vi "Striptest.vi"(1 "Simulation?":bool) -> ()   [LabVIEW 2019]
uses:
  InstrControl/LCRControl/LCRControl.lvclass
  C:/Users/Graham Greig/Desktop/itk-strip-sensor-qc/LabVIEW 2019/InstrControl/InstrControl.lvclass
  general_VIs/globals/QC_MeasurementSetup.vi
  striptest/ProbePlan/ProbePlanParams.vi
  general_VIs/globals/QC_RunInformation.vi
  InstrControl/InstrumentSetup.vi
  <vilib>/regexp/Match Regular Expression.xnode
  InstrControl/SupplyControl/SupplyControl.lvclass
  InstrControl/Switching/Switching.lvclass
  InstrControl/ProbeStationControl/ProbeStationControl.lvclass
  InstrControl/InstrControl.lvclass
  InstrControl/ArduinoControl/ArduinoControl.lvclass
  <vilib>/Analysis/NI_AALBase.lvlib
panel:
  out "Tab Control":enum32{"Striptest Setup", "Striptest"}(tab)
  in  "Switching":string(combo)="LXIPXI Switching"
  in  "Bias Voltage [V]":dbl=-150.0 format="%.1f"
  in  "Frequency [Hz] Setup":i32=1000 caption="Frequency [Hz]" format="%#.3p"
  in  "Minimum fraction\nof good strips":dbl=98.0 format="%.1g"
  in  "Quit":bool
  in  "Continue":bool
  in  "Measurement Configurations":bool
  in  "Pinholes Y/N":bool=TRUE
  in  "Capacitance Y/N":bool=TRUE
  in  "Resistance Y/N":bool=TRUE
  in  "Striptest SMU":string(combo)="Keithley 2657A"
  in  "LCR Meter":string(combo)="WayneKerr 6440B"
  in  "Temperature":enum16{"Read Arduino", "Enter manually"}(ring)
  in  "Bias Supply":string(combo)="Keithley 2410"
  in  "Hardware Configurations":bool
  in  "DB Serial No. IN:":string caption="DB Serial No.:"
  in  "User:":string(combo)="Graham"
  in  "Batch No. IN:":string caption="Batch No.:"
  in  "Device Category IN:":string(combo)="ATLAS12EC" caption="Device Category:"
  in  "Sensor Serial No. IN:":string caption="Sensor Serial No.:"
  in  "From4":u16(ring) items=["Strip 0", "Strip 1", "Strip 2", "Strip 3", "Strip 4", "Strip 5", "Strip 6", "Strip 7", "Strip 8", "Strip 9", "Strip 10", "Strip 11", "Strip 12", "Strip 13", "Strip 14", "Strip 15", "Strip 16", "Strip 17", "Strip 18", "Strip 19", "Strip 20", "Strip 21", "Strip 22", "Strip 23", "Strip 24", "Strip 25", "Strip 26", "Strip 27", "Strip 28", "Strip 29", "Strip 30", "Strip 31", "Strip 32", "Strip 33", "Strip 34", "Strip 35", "Strip 36", "Strip 37", "Strip 38", "Strip 39", "Strip 40", "Strip 41", "Strip 42", "Strip 43", "Strip 44", "Strip 45", "Strip 46", "Strip 47", "Strip 48", "Strip 49", "Strip 50", "Strip 51", "Strip 52", "Strip 53", "Strip 54", "Strip 55", "Strip 56", "Strip 57", "Strip 58", "Strip 59", "Strip 60", "Strip 61", "Strip 62", "Strip 63", "Strip 64", "Strip 65", "Strip 66", "Strip 67", "Strip 68", "Strip 69", "Strip 70", "Strip 71", "Strip 72", "Strip 73", "Strip 74", "Strip 75", "Strip 76", "Strip 77", "Strip 78", "Strip 79", "Strip 80", "Strip 81", "Strip 82", "Strip 83", "Strip 84", "Strip 85", "Strip 86", "Strip 87", "Strip 88", "Strip 89", "Strip 90", "Strip 91", "Strip 92", "Strip 93", "Strip 94", "Strip 95", "Strip 96", "Strip 97", "Strip 98", "Strip 99", "Strip 100", "Strip 101", "Strip 102", "Strip 103", "Strip 104", "Strip 105", "Strip 106", "Strip 107", "Strip 108", "Strip 109", "Strip 110", "Strip 111", "Strip 112", "Strip 113", "Strip 114", "Strip 115", "Strip 116", "Strip 117", "Strip 118", "Strip 119", "Strip 120", "Strip 121", "Strip 122", "Strip 123", "Strip 124", "Strip 125", "Strip 126", "Strip 127", "Strip 128", "Strip 129", "Strip 130", "Strip 131", "Strip 132", "Strip 133", "Strip 134", "Strip 135", "Strip 136", "Strip 137", "Strip 138", "Strip 139", "Strip 140", "Strip 141", "Strip 142", "Strip 143", "Strip 144", "Strip 145", "Strip 146", "Strip 147", "Strip 148", "Strip 149", "Strip 150", "Strip 151", "Strip 152", "Strip 153", "Strip 154", "Strip 155", "Strip 156", "Strip 157", "Strip 158", "Strip 159", "Strip 160", "Strip 161", "Strip 162", "Strip 163", "Strip 164", "Strip 165", "Strip 166", "Strip 167", "Strip 168", "Strip 169", "Strip 170", "Strip 171", "Strip 172", "Strip 173", "Strip 174", "Strip 175", "Strip 176", "Strip 177", "Strip 178", "Strip 179", "Strip 180", "Strip 181", "Strip 182", "Strip 183", "Strip 184", "Strip 185", "Strip 186", "Strip 187", "Strip 188", "Strip 189", "Strip 190", "Strip 191", "Strip 192", "Strip 193", "Strip 194", "Strip 195", "Strip 196", "Strip 197", "Strip 198", "Strip 199", "Strip 200", "Strip 201", "Strip 202", "Strip 203", "Strip 204", "Strip 205", "Strip 206", "Strip 207", "Strip 208", "Strip 209", "Strip 210", "Strip 211", "Strip 212", "Strip 213", "Strip 214", "Strip 215", "Strip 216", "Strip 217", "Strip 218", "Strip 219", "Strip 220", "Strip 221", "Strip 222", "Strip 223", "Strip 224", "Strip 225", "Strip 226", "Strip 227", "Strip 228", "Strip 229", "Strip 230", "Strip 231", "Strip 232", "Strip 233", "Strip 234", "Strip 235", "Strip 236", "Strip 237", "Strip 238", "Strip 239", "Strip 240", "Strip 241", "Strip 242", "Strip 243", "Strip 244", "Strip 245", "Strip 246", "Strip 247", "Strip 248", "Strip 249", "Strip 250", "Strip 251", "Strip 252", "Strip 253", "Strip 254", "Strip 255", "Strip 256", "Strip 257", "Strip 258", "Strip 259", "Strip 260", "Strip 261", "Strip 262", "Strip 263", "Strip 264", "Strip 265", "Strip 266", "Strip 267", "Strip 268", "Strip 269", "Strip 270", "Strip 271", "Strip 272", "Strip 273", "Strip 274", "Strip 275", "Strip 276", "Strip 277", "Strip 278", "Strip 279", "Strip 280", "Strip 281", "Strip 282", "Strip 283", "Strip 284", "Strip 285", "Strip 286", "Strip 287", "Strip 288", "Strip 289", "Strip 290", "Strip 291", "Strip 292", "Strip 293", "Strip 294", "Strip 295", "Strip 296", "Strip 297", "Strip 298", "Strip 299", "Strip 300", "Strip 301", "Strip 302", "Strip 303", "Strip 304", "Strip 305", "Strip 306", "Strip 307", "Strip 308", "Strip 309", "Strip 310", "Strip 311", "Strip 312", "Strip 313", "Strip 314", "Strip 315", "Strip 316", "Strip 317", "Strip 318", "Strip 319", "Strip 320", "Strip 321", "Strip 322", "Strip 323", "Strip 324", "Strip 325", "Strip 326", "Strip 327", "Strip 328", "Strip 329", "Strip 330", "Strip 331", "Strip 332", "Strip 333", "Strip 334", "Strip 335", "Strip 336", "Strip 337", "Strip 338", "Strip 339", "Strip 340", "Strip 341", "Strip 342", "Strip 343", "Strip 344", "Strip 345", "Strip 346", "Strip 347", "Strip 348", "Strip 349", "Strip 350", "Strip 351", "Strip 352", "Strip 353", "Strip 354", "Strip 355", "Strip 356", "Strip 357", "Strip 358", "Strip 359", "Strip 360", "Strip 361", "Strip 362", "Strip 363", "Strip 364", "Strip 365", "Strip 366", "Strip 367", "Strip 368", "Strip 369", "Strip 370", "Strip 371", "Strip 372", "Strip 373", "Strip 374", "Strip 375", "Strip 376", "Strip 377", "Strip 378", "Strip 379", "Strip 380", "Strip 381", "Strip 382", "Strip 383", "Strip 384", "Strip 385", "Strip 386", "Strip 387", "Strip 388", "Strip 389", "Strip 390", "Strip 391", "Strip 392", "Strip 393", "Strip 394", "Strip 395", "Strip 396", "Strip 397", "Strip 398", "Strip 399", "Strip 400", "Strip 401", "Strip 402", "Strip 403", "Strip 404", "Strip 405", "Strip 406", "Strip 407", "Strip 408", "Strip 409", "Strip 410", "Strip 411", "Strip 412", "Strip 413", "Strip 414", "Strip 415", "Strip 416", "Strip 417", "Strip 418", "Strip 419", "Strip 420", "Strip 421", "Strip 422", "Strip 423", "Strip 424", "Strip 425", "Strip 426", "Strip 427", "Strip 428", "Strip 429", "Strip 430", "Strip 431", "Strip 432", "Strip 433", "Strip 434", "Strip 435", "Strip 436", "Strip 437", "Strip 438", "Strip 439", "Strip 440", "Strip 441", "Strip 442", "Strip 443", "Strip 444", "Strip 445", "Strip 446", "Strip 447", "Strip 448", "Strip 449", "Strip 450", "Strip 451", "Strip 452", "Strip 453", "Strip 454", "Strip 455", "Strip 456", "Strip 457", "Strip 458", "Strip 459", "Strip 460", "Strip 461", "Strip 462", "Strip 463", "Strip 464", "Strip 465", "Strip 466", "Strip 467", "Strip 468", "Strip 469", "Strip 470", "Strip 471", "Strip 472", "Strip 473", "Strip 474", "Strip 475", "Strip 476", "Strip 477", "Strip 478", "Strip 479", "Strip 480", "Strip 481", "Strip 482", "Strip 483", "Strip 484", "Strip 485", "Strip 486", "Strip 487", "Strip 488", "Strip 489", "Strip 490", "Strip 491", "Strip 492", "Strip 493", "Strip 494", "Strip 495", "Strip 496", "Strip 497", "Strip 498", "Strip 499", "Strip 500", "Strip 501", "Strip 502", "Strip 503", "Strip 504", "Strip 505", "Strip 506", "Strip 507", "Strip 508", "Strip 509", "Strip 510", "Strip 511", "Strip 512", "Strip 513", "Strip 514", "Strip 515", "Strip 516", "Strip 517", "Strip 518", "Strip 519", "Strip 520", "Strip 521", "Strip 522", "Strip 523", "Strip 524", "Strip 525", "Strip 526", "Strip 527", "Strip 528", "Strip 529", "Strip 530", "Strip 531", "Strip 532", "Strip 533", "Strip 534", "Strip 535", "Strip 536", "Strip 537", "Strip 538", "Strip 539", "Strip 540", "Strip 541", "Strip 542", "Strip 543", "Strip 544", "Strip 545", "Strip 546", "Strip 547", "Strip 548", "Strip 549", "Strip 550", "Strip 551", "Strip 552", "Strip 553", "Strip 554", "Strip 555", "Strip 556", "Strip 557", "Strip 558", "Strip 559", "Strip 560", "Strip 561", "Strip 562", "Strip 563", "Strip 564", "Strip 565", "Strip 566", "Strip 567", "Strip 568", "Strip 569", "Strip 570", "Strip 571", "Strip 572", "Strip 573", "Strip 574", "Strip 575", "Strip 576", "Strip 577", "Strip 578", "Strip 579", "Strip 580", "Strip 581", "Strip 582", "Strip 583", "Strip 584", "Strip 585", "Strip 586", "Strip 587", "Strip 588", "Strip 589", "Strip 590", "Strip 591", "Strip 592", "Strip 593", "Strip 594", "Strip 595", "Strip 596", "Strip 597", "Strip 598", "Strip 599", "Strip 600", "Strip 601", "Strip 602", "Strip 603", "Strip 604", "Strip 605", "Strip 606", "Strip 607", "Strip 608", "Strip 609", "Strip 610", "Strip 611", "Strip 612", "Strip 613", "Strip 614", "Strip 615", "Strip 616", "Strip 617", "Strip 618", "Strip 619", "Strip 620", "Strip 621", "Strip 622", "Strip 623", "Strip 624", "Strip 625", "Strip 626", "Strip 627", "Strip 628", "Strip 629", "Strip 630", "Strip 631", "Strip 632", "Strip 633", "Strip 634", "Strip 635", "Strip 636", "Strip 637", "Strip 638", "Strip 639", "Strip 640", "Strip 641", "Strip 642", "Strip 643", "Strip 644", "Strip 645", "Strip 646", "Strip 647", "Strip 648", "Strip 649", "Strip 650", "Strip 651", "Strip 652", "Strip 653", "Strip 654", "Strip 655", "Strip 656", "Strip 657", "Strip 658", "Strip 659", "Strip 660", "Strip 661", "Strip 662", "Strip 663", "Strip 664", "Strip 665", "Strip 666", "Strip 667", "Strip 668", "Strip 669", "Strip 670", "Strip 671", "Strip 672", "Strip 673", "Strip 674", "Strip 675", "Strip 676", "Strip 677", "Strip 678", "Strip 679", "Strip 680", "Strip 681", "Strip 682", "Strip 683", "Strip 684", "Strip 685", "Strip 686", "Strip 687", "Strip 688", "Strip 689", "Strip 690", "Strip 691", "Strip 692", "Strip 693", "Strip 694", "Strip 695", "Strip 696", "Strip 697", "Strip 698", "Strip 699", "Strip 700", "Strip 701", "Strip 702", "Strip 703", "Strip 704", "Strip 705", "Strip 706", "Strip 707", "Strip 708", "Strip 709", "Strip 710", "Strip 711", "Strip 712", "Strip 713", "Strip 714", "Strip 715", "Strip 716", "Strip 717", "Strip 718", "Strip 719", "Strip 720", "Strip 721", "Strip 722", "Strip 723", "Strip 724", "Strip 725", "Strip 726", "Strip 727", "Strip 728", "Strip 729", "Strip 730", "Strip 731", "Strip 732", "Strip 733", "Strip 734", "Strip 735", "Strip 736", "Strip 737", "Strip 738", "Strip 739", "Strip 740", "Strip 741", "Strip 742", "Strip 743", "Strip 744", "Strip 745", "Strip 746", "Strip 747", "Strip 748", "Strip 749", "Strip 750", "Strip 751", "Strip 752", "Strip 753", "Strip 754", "Strip 755", "Strip 756", "Strip 757", "Strip 758", "Strip 759", "Strip 760", "Strip 761", "Strip 762", "Strip 763", "Strip 764", "Strip 765", "Strip 766", "Strip 767", "Strip 768", "Strip 769", "Strip 770", "Strip 771", "Strip 772", "Strip 773", "Strip 774", "Strip 775", "Strip 776", "Strip 777", "Strip 778", "Strip 779", "Strip 780", "Strip 781", "Strip 782", "Strip 783", "Strip 784", "Strip 785", "Strip 786", "Strip 787", "Strip 788", "Strip 789", "Strip 790", "Strip 791", "Strip 792", "Strip 793", "Strip 794", "Strip 795", "Strip 796", "Strip 797", "Strip 798", "Strip 799", "Strip 800", "Strip 801", "Strip 802", "Strip 803", "Strip 804", "Strip 805", "Strip 806", "Strip 807", "Strip 808", "Strip 809", "Strip 810", "Strip 811", "Strip 812", "Strip 813", "Strip 814", "Strip 815", "Strip 816", "Strip 817", "Strip 818", "Strip 819", "Strip 820", "Strip 821", "Strip 822", "Strip 823", "Strip 824", "Strip 825", "Strip 826", "Strip 827", "Strip 828", "Strip 829", "Strip 830", "Strip 831", "Strip 832", "Strip 833", "Strip 834", "Strip 835", "Strip 836", "Strip 837", "Strip 838", "Strip 839", "Strip 840", "Strip 841", "Strip 842", "Strip 843", "Strip 844", "Strip 845", "Strip 846", "Strip 847", "Strip 848", "Strip 849", "Strip 850", "Strip 851", "Strip 852", "Strip 853", "Strip 854", "Strip 855", "Strip 856", "Strip 857", "Strip 858", "Strip 859", "Strip 860", "Strip 861", "Strip 862", "Strip 863", "Strip 864", "Strip 865", "Strip 866", "Strip 867", "Strip 868", "Strip 869", "Strip 870", "Strip 871", "Strip 872", "Strip 873", "Strip 874", "Strip 875", "Strip 876", "Strip 877", "Strip 878", "Strip 879", "Strip 880", "Strip 881", "Strip 882", "Strip 883", "Strip 884", "Strip 885", "Strip 886", "Strip 887", "Strip 888", "Strip 889", "Strip 890", "Strip 891", "Strip 892", "Strip 893", "Strip 894", "Strip 895", "Strip 896", "Strip 897", "Strip 898", "Strip 899", "Strip 900", "Strip 901", "Strip 902", "Strip 903", "Strip 904", "Strip 905", "Strip 906", "Strip 907", "Strip 908", "Strip 909", "Strip 910", "Strip 911", "Strip 912", "Strip 913", "Strip 914", "Strip 915", "Strip 916", "Strip 917", "Strip 918", "Strip 919", "Strip 920", "Strip 921", "Strip 922", "Strip 923", "Strip 924", "Strip 925", "Strip 926", "Strip 927", "Strip 928", "Strip 929", "Strip 930", "Strip 931", "Strip 932", "Strip 933", "Strip 934", "Strip 935", "Strip 936", "Strip 937", "Strip 938", "Strip 939", "Strip 940", "Strip 941", "Strip 942", "Strip 943", "Strip 944", "Strip 945", "Strip 946", "Strip 947", "Strip 948", "Strip 949", "Strip 950", "Strip 951", "Strip 952", "Strip 953", "Strip 954", "Strip 955", "Strip 956", "Strip 957", "Strip 958", "Strip 959", "Strip 960", "Strip 961", "Strip 962", "Strip 963", "Strip 964", "Strip 965", "Strip 966", "Strip 967", "Strip 968", "Strip 969", "Strip 970", "Strip 971", "Strip 972", "Strip 973", "Strip 974", "Strip 975", "Strip 976", "Strip 977", "Strip 978", "Strip 979", "Strip 980", "Strip 981", "Strip 982", "Strip 983", "Strip 984", "Strip 985", "Strip 986", "Strip 987", "Strip 988", "Strip 989", "Strip 990", "Strip 991", "Strip 992", "Strip 993", "Strip 994", "Strip 995", "Strip 996", "Strip 997", "Strip 998", "Strip 999", "Strip 1000", "Strip 1001", "Strip 1002", "Strip 1003", "Strip 1004", "Strip 1005", "Strip 1006", "Strip 1007", "Strip 1008", "Strip 1009", "Strip 1010", "Strip 1011", "Strip 1012", "Strip 1013", "Strip 1014", "Strip 1015", "Strip 1016", "Strip 1017", "Strip 1018", "Strip 1019", "Strip 1020", "Strip 1021", "Strip 1022", "Strip 1023", "Strip 1024", "Strip 1025", "Strip 1026", "Strip 1027", "Strip 1028", "Strip 1029", "Strip 1030", "Strip 1031", "Strip 1032", "Strip 1033", "Strip 1034", "Strip 1035", "Strip 1036", "Strip 1037", "Strip 1038", "Strip 1039", "Strip 1040", "Strip 1041", "Strip 1042", "Strip 1043", "Strip 1044", "Strip 1045", "Strip 1046", "Strip 1047", "Strip 1048", "Strip 1049", "Strip 1050", "Strip 1051", "Strip 1052", "Strip 1053", "Strip 1054", "Strip 1055", "Strip 1056", "Strip 1057", "Strip 1058", "Strip 1059", "Strip 1060", "Strip 1061", "Strip 1062", "Strip 1063", "Strip 1064", "Strip 1065", "Strip 1066", "Strip 1067", "Strip 1068", "Strip 1069", "Strip 1070", "Strip 1071", "Strip 1072", "Strip 1073", "Strip 1074", "Strip 1075", "Strip 1076", "Strip 1077", "Strip 1078", "Strip 1079", "Strip 1080", "Strip 1081", "Strip 1082", "Strip 1083", "Strip 1084", "Strip 1085", "Strip 1086", "Strip 1087", "Strip 1088", "Strip 1089", "Strip 1090", "Strip 1091", "Strip 1092", "Strip 1093", "Strip 1094", "Strip 1095", "Strip 1096", "Strip 1097", "Strip 1098", "Strip 1099", "Strip 1100", "Strip 1101", "Strip 1102", "Strip 1103", "Strip 1104", "Strip 1105", "Strip 1106", "Strip 1107", "Strip 1108", "Strip 1109", "Strip 1110", "Strip 1111", "Strip 1112", "Strip 1113", "Strip 1114", "Strip 1115", "Strip 1116", "Strip 1117", "Strip 1118", "Strip 1119", "Strip 1120", "Strip 1121", "Strip 1122", "Strip 1123", "Strip 1124", "Strip 1125", "Strip 1126", "Strip 1127", "Strip 1128", "Strip 1129", "Strip 1130", "Strip 1131", "Strip 1132", "Strip 1133", "Strip 1134", "Strip 1135", "Strip 1136", "Strip 1137", "Strip 1138", "Strip 1139", "Strip 1140", "Strip 1141", "Strip 1142", "Strip 1143", "Strip 1144", "Strip 1145", "Strip 1146", "Strip 1147", "Strip 1148", "Strip 1149", "Strip 1150", "Strip 1151", "Strip 1152", "Strip 1153", "Strip 1154", "Strip 1155", "Strip 1156", "Strip 1157", "Strip 1158", "Strip 1159", "Strip 1160", "Strip 1161", "Strip 1162", "Strip 1163", "Strip 1164", "Strip 1165", "Strip 1166", "Strip 1167", "Strip 1168", "Strip 1169", "Strip 1170", "Strip 1171", "Strip 1172", "Strip 1173", "Strip 1174", "Strip 1175", "Strip 1176", "Strip 1177", "Strip 1178", "Strip 1179", "Strip 1180", "Strip 1181", "Strip 1182", "Strip 1183", "Strip 1184", "Strip 1185", "Strip 1186", "Strip 1187", "Strip 1188", "Strip 1189", "Strip 1190", "Strip 1191", "Strip 1192", "Strip 1193", "Strip 1194", "Strip 1195", "Strip 1196", "Strip 1197", "Strip 1198", "Strip 1199", "Strip 1200", "Strip 1201", "Strip 1202", "Strip 1203", "Strip 1204", "Strip 1205", "Strip 1206", "Strip 1207", "Strip 1208", "Strip 1209", "Strip 1210", "Strip 1211", "Strip 1212", "Strip 1213", "Strip 1214", "Strip 1215", "Strip 1216", "Strip 1217", "Strip 1218", "Strip 1219", "Strip 1220", "Strip 1221", "Strip 1222", "Strip 1223", "Strip 1224", "Strip 1225", "Strip 1226", "Strip 1227", "Strip 1228", "Strip 1229", "Strip 1230", "Strip 1231", "Strip 1232", "Strip 1233", "Strip 1234", "Strip 1235", "Strip 1236", "Strip 1237", "Strip 1238", "Strip 1239", "Strip 1240", "Strip 1241", "Strip 1242", "Strip 1243", "Strip 1244", "Strip 1245", "Strip 1246", "Strip 1247", "Strip 1248", "Strip 1249", "Strip 1250", "Strip 1251", "Strip 1252", "Strip 1253", "Strip 1254", "Strip 1255", "Strip 1256", "Strip 1257", "Strip 1258", "Strip 1259", "Strip 1260", "Strip 1261", "Strip 1262", "Strip 1263", "Strip 1264", "Strip 1265", "Strip 1266", "Strip 1267", "Strip 1268", "Strip 1269", "Strip 1270", "Strip 1271", "Strip 1272", "Strip 1273", "Strip 1274", "Strip 1275", "Strip 1276", "Strip 1277", "Strip 1278", "Strip 1279", "Strip 1280", "Strip 1281", "Strip 1282", "Strip 1283", "Strip 1284", "Strip 1285", "Strip 1286", "Strip 1287", "Strip 1288", "Strip 1289", "Strip 1290", "Strip 1291", "Strip 1292", "Strip 1293", "Strip 1294", "Strip 1295", "Strip 1296", "Strip 1297", "Strip 1298", "Strip 1299", "Strip 1300", "Strip 1301", "Strip 1302", "Strip 1303", "Strip 1304", "Strip 1305", "Strip 1306", "Strip 1307", "Strip 1308", "Strip 1309", "Strip 1310", "Strip 1311", "Strip 1312", "Strip 1313", "Strip 1314", "Strip 1315", "Strip 1316", "Strip 1317", "Strip 1318", "Strip 1319", "Strip 1320", "Strip 1321", "Strip 1322", "Strip 1323", "Strip 1324", "Strip 1325", "Strip 1326", "Strip 1327", "Strip 1328", "Strip 1329", "Strip 1330", "Strip 1331", "Strip 1332", "Strip 1333", "Strip 1334", "Strip 1335", "Strip 1336", "Strip 1337", "Strip 1338", "Strip 1339", "Strip 1340", "Strip 1341", "Strip 1342", "Strip 1343", "Strip 1344", "Strip 1345", "Strip 1346", "Strip 1347", "Strip 1348", "Strip 1349", "Strip 1350", "Strip 1351", "Strip 1352", "Strip 1353", "Strip 1354", "Strip 1355", "Strip 1356", "Strip 1357", "Strip 1358", "Strip 1359", "Strip 1360", "Strip 1361", "Strip 1362", "Strip 1363", "Strip 1364", "Strip 1365", "Strip 1366", "Strip 1367", "Strip 1368", "Strip 1369", "Strip 1370", "Strip 1371", "Strip 1372", "Strip 1373", "Strip 1374", "Strip 1375", "Strip 1376", "Strip 1377", "Strip 1378", "Strip 1379", "Strip 1380", "Strip 1381", "Strip 1382", "Strip 1383", "Strip 1384", "Strip 1385", "Strip 1386", "Strip 1387", "Strip 1388", "Strip 1389", "Strip 1390", "Strip 1391", "Strip 1392", "Strip 1393", "Strip 1394", "Strip 1395", "Strip 1396", "Strip 1397", "Strip 1398", "Strip 1399", "Strip 1400", "Strip 1401", "Strip 1402", "Strip 1403", "Strip 1404", "Strip 1405", "Strip 1406", "Strip 1407", "Strip 1408", "Strip 1409"]
  in  "From3":u16(ring) items=["Strip 0", "Strip 1", "Strip 2", "Strip 3", "Strip 4", "Strip 5", "Strip 6", "Strip 7", "Strip 8", "Strip 9", "Strip 10", "Strip 11", "Strip 12", "Strip 13", "Strip 14", "Strip 15", "Strip 16", "Strip 17", "Strip 18", "Strip 19", "Strip 20", "Strip 21", "Strip 22", "Strip 23", "Strip 24", "Strip 25", "Strip 26", "Strip 27", "Strip 28", "Strip 29", "Strip 30", "Strip 31", "Strip 32", "Strip 33", "Strip 34", "Strip 35", "Strip 36", "Strip 37", "Strip 38", "Strip 39", "Strip 40", "Strip 41", "Strip 42", "Strip 43", "Strip 44", "Strip 45", "Strip 46", "Strip 47", "Strip 48", "Strip 49", "Strip 50", "Strip 51", "Strip 52", "Strip 53", "Strip 54", "Strip 55", "Strip 56", "Strip 57", "Strip 58", "Strip 59", "Strip 60", "Strip 61", "Strip 62", "Strip 63", "Strip 64", "Strip 65", "Strip 66", "Strip 67", "Strip 68", "Strip 69", "Strip 70", "Strip 71", "Strip 72", "Strip 73", "Strip 74", "Strip 75", "Strip 76", "Strip 77", "Strip 78", "Strip 79", "Strip 80", "Strip 81", "Strip 82", "Strip 83", "Strip 84", "Strip 85", "Strip 86", "Strip 87", "Strip 88", "Strip 89", "Strip 90", "Strip 91", "Strip 92", "Strip 93", "Strip 94", "Strip 95", "Strip 96", "Strip 97", "Strip 98", "Strip 99", "Strip 100", "Strip 101", "Strip 102", "Strip 103", "Strip 104", "Strip 105", "Strip 106", "Strip 107", "Strip 108", "Strip 109", "Strip 110", "Strip 111", "Strip 112", "Strip 113", "Strip 114", "Strip 115", "Strip 116", "Strip 117", "Strip 118", "Strip 119", "Strip 120", "Strip 121", "Strip 122", "Strip 123", "Strip 124", "Strip 125", "Strip 126", "Strip 127", "Strip 128", "Strip 129", "Strip 130", "Strip 131", "Strip 132", "Strip 133", "Strip 134", "Strip 135", "Strip 136", "Strip 137", "Strip 138", "Strip 139", "Strip 140", "Strip 141", "Strip 142", "Strip 143", "Strip 144", "Strip 145", "Strip 146", "Strip 147", "Strip 148", "Strip 149", "Strip 150", "Strip 151", "Strip 152", "Strip 153", "Strip 154", "Strip 155", "Strip 156", "Strip 157", "Strip 158", "Strip 159", "Strip 160", "Strip 161", "Strip 162", "Strip 163", "Strip 164", "Strip 165", "Strip 166", "Strip 167", "Strip 168", "Strip 169", "Strip 170", "Strip 171", "Strip 172", "Strip 173", "Strip 174", "Strip 175", "Strip 176", "Strip 177", "Strip 178", "Strip 179", "Strip 180", "Strip 181", "Strip 182", "Strip 183", "Strip 184", "Strip 185", "Strip 186", "Strip 187", "Strip 188", "Strip 189", "Strip 190", "Strip 191", "Strip 192", "Strip 193", "Strip 194", "Strip 195", "Strip 196", "Strip 197", "Strip 198", "Strip 199", "Strip 200", "Strip 201", "Strip 202", "Strip 203", "Strip 204", "Strip 205", "Strip 206", "Strip 207", "Strip 208", "Strip 209", "Strip 210", "Strip 211", "Strip 212", "Strip 213", "Strip 214", "Strip 215", "Strip 216", "Strip 217", "Strip 218", "Strip 219", "Strip 220", "Strip 221", "Strip 222", "Strip 223", "Strip 224", "Strip 225", "Strip 226", "Strip 227", "Strip 228", "Strip 229", "Strip 230", "Strip 231", "Strip 232", "Strip 233", "Strip 234", "Strip 235", "Strip 236", "Strip 237", "Strip 238", "Strip 239", "Strip 240", "Strip 241", "Strip 242", "Strip 243", "Strip 244", "Strip 245", "Strip 246", "Strip 247", "Strip 248", "Strip 249", "Strip 250", "Strip 251", "Strip 252", "Strip 253", "Strip 254", "Strip 255", "Strip 256", "Strip 257", "Strip 258", "Strip 259", "Strip 260", "Strip 261", "Strip 262", "Strip 263", "Strip 264", "Strip 265", "Strip 266", "Strip 267", "Strip 268", "Strip 269", "Strip 270", "Strip 271", "Strip 272", "Strip 273", "Strip 274", "Strip 275", "Strip 276", "Strip 277", "Strip 278", "Strip 279", "Strip 280", "Strip 281", "Strip 282", "Strip 283", "Strip 284", "Strip 285", "Strip 286", "Strip 287", "Strip 288", "Strip 289", "Strip 290", "Strip 291", "Strip 292", "Strip 293", "Strip 294", "Strip 295", "Strip 296", "Strip 297", "Strip 298", "Strip 299", "Strip 300", "Strip 301", "Strip 302", "Strip 303", "Strip 304", "Strip 305", "Strip 306", "Strip 307", "Strip 308", "Strip 309", "Strip 310", "Strip 311", "Strip 312", "Strip 313", "Strip 314", "Strip 315", "Strip 316", "Strip 317", "Strip 318", "Strip 319", "Strip 320", "Strip 321", "Strip 322", "Strip 323", "Strip 324", "Strip 325", "Strip 326", "Strip 327", "Strip 328", "Strip 329", "Strip 330", "Strip 331", "Strip 332", "Strip 333", "Strip 334", "Strip 335", "Strip 336", "Strip 337", "Strip 338", "Strip 339", "Strip 340", "Strip 341", "Strip 342", "Strip 343", "Strip 344", "Strip 345", "Strip 346", "Strip 347", "Strip 348", "Strip 349", "Strip 350", "Strip 351", "Strip 352", "Strip 353", "Strip 354", "Strip 355", "Strip 356", "Strip 357", "Strip 358", "Strip 359", "Strip 360", "Strip 361", "Strip 362", "Strip 363", "Strip 364", "Strip 365", "Strip 366", "Strip 367", "Strip 368", "Strip 369", "Strip 370", "Strip 371", "Strip 372", "Strip 373", "Strip 374", "Strip 375", "Strip 376", "Strip 377", "Strip 378", "Strip 379", "Strip 380", "Strip 381", "Strip 382", "Strip 383", "Strip 384", "Strip 385", "Strip 386", "Strip 387", "Strip 388", "Strip 389", "Strip 390", "Strip 391", "Strip 392", "Strip 393", "Strip 394", "Strip 395", "Strip 396", "Strip 397", "Strip 398", "Strip 399", "Strip 400", "Strip 401", "Strip 402", "Strip 403", "Strip 404", "Strip 405", "Strip 406", "Strip 407", "Strip 408", "Strip 409", "Strip 410", "Strip 411", "Strip 412", "Strip 413", "Strip 414", "Strip 415", "Strip 416", "Strip 417", "Strip 418", "Strip 419", "Strip 420", "Strip 421", "Strip 422", "Strip 423", "Strip 424", "Strip 425", "Strip 426", "Strip 427", "Strip 428", "Strip 429", "Strip 430", "Strip 431", "Strip 432", "Strip 433", "Strip 434", "Strip 435", "Strip 436", "Strip 437", "Strip 438", "Strip 439", "Strip 440", "Strip 441", "Strip 442", "Strip 443", "Strip 444", "Strip 445", "Strip 446", "Strip 447", "Strip 448", "Strip 449", "Strip 450", "Strip 451", "Strip 452", "Strip 453", "Strip 454", "Strip 455", "Strip 456", "Strip 457", "Strip 458", "Strip 459", "Strip 460", "Strip 461", "Strip 462", "Strip 463", "Strip 464", "Strip 465", "Strip 466", "Strip 467", "Strip 468", "Strip 469", "Strip 470", "Strip 471", "Strip 472", "Strip 473", "Strip 474", "Strip 475", "Strip 476", "Strip 477", "Strip 478", "Strip 479", "Strip 480", "Strip 481", "Strip 482", "Strip 483", "Strip 484", "Strip 485", "Strip 486", "Strip 487", "Strip 488", "Strip 489", "Strip 490", "Strip 491", "Strip 492", "Strip 493", "Strip 494", "Strip 495", "Strip 496", "Strip 497", "Strip 498", "Strip 499", "Strip 500", "Strip 501", "Strip 502", "Strip 503", "Strip 504", "Strip 505", "Strip 506", "Strip 507", "Strip 508", "Strip 509", "Strip 510", "Strip 511", "Strip 512", "Strip 513", "Strip 514", "Strip 515", "Strip 516", "Strip 517", "Strip 518", "Strip 519", "Strip 520", "Strip 521", "Strip 522", "Strip 523", "Strip 524", "Strip 525", "Strip 526", "Strip 527", "Strip 528", "Strip 529", "Strip 530", "Strip 531", "Strip 532", "Strip 533", "Strip 534", "Strip 535", "Strip 536", "Strip 537", "Strip 538", "Strip 539", "Strip 540", "Strip 541", "Strip 542", "Strip 543", "Strip 544", "Strip 545", "Strip 546", "Strip 547", "Strip 548", "Strip 549", "Strip 550", "Strip 551", "Strip 552", "Strip 553", "Strip 554", "Strip 555", "Strip 556", "Strip 557", "Strip 558", "Strip 559", "Strip 560", "Strip 561", "Strip 562", "Strip 563", "Strip 564", "Strip 565", "Strip 566", "Strip 567", "Strip 568", "Strip 569", "Strip 570", "Strip 571", "Strip 572", "Strip 573", "Strip 574", "Strip 575", "Strip 576", "Strip 577", "Strip 578", "Strip 579", "Strip 580", "Strip 581", "Strip 582", "Strip 583", "Strip 584", "Strip 585", "Strip 586", "Strip 587", "Strip 588", "Strip 589", "Strip 590", "Strip 591", "Strip 592", "Strip 593", "Strip 594", "Strip 595", "Strip 596", "Strip 597", "Strip 598", "Strip 599", "Strip 600", "Strip 601", "Strip 602", "Strip 603", "Strip 604", "Strip 605", "Strip 606", "Strip 607", "Strip 608", "Strip 609", "Strip 610", "Strip 611", "Strip 612", "Strip 613", "Strip 614", "Strip 615", "Strip 616", "Strip 617", "Strip 618", "Strip 619", "Strip 620", "Strip 621", "Strip 622", "Strip 623", "Strip 624", "Strip 625", "Strip 626", "Strip 627", "Strip 628", "Strip 629", "Strip 630", "Strip 631", "Strip 632", "Strip 633", "Strip 634", "Strip 635", "Strip 636", "Strip 637", "Strip 638", "Strip 639", "Strip 640", "Strip 641", "Strip 642", "Strip 643", "Strip 644", "Strip 645", "Strip 646", "Strip 647", "Strip 648", "Strip 649", "Strip 650", "Strip 651", "Strip 652", "Strip 653", "Strip 654", "Strip 655", "Strip 656", "Strip 657", "Strip 658", "Strip 659", "Strip 660", "Strip 661", "Strip 662", "Strip 663", "Strip 664", "Strip 665", "Strip 666", "Strip 667", "Strip 668", "Strip 669", "Strip 670", "Strip 671", "Strip 672", "Strip 673", "Strip 674", "Strip 675", "Strip 676", "Strip 677", "Strip 678", "Strip 679", "Strip 680", "Strip 681", "Strip 682", "Strip 683", "Strip 684", "Strip 685", "Strip 686", "Strip 687", "Strip 688", "Strip 689", "Strip 690", "Strip 691", "Strip 692", "Strip 693", "Strip 694", "Strip 695", "Strip 696", "Strip 697", "Strip 698", "Strip 699", "Strip 700", "Strip 701", "Strip 702", "Strip 703", "Strip 704", "Strip 705", "Strip 706", "Strip 707", "Strip 708", "Strip 709", "Strip 710", "Strip 711", "Strip 712", "Strip 713", "Strip 714", "Strip 715", "Strip 716", "Strip 717", "Strip 718", "Strip 719", "Strip 720", "Strip 721", "Strip 722", "Strip 723", "Strip 724", "Strip 725", "Strip 726", "Strip 727", "Strip 728", "Strip 729", "Strip 730", "Strip 731", "Strip 732", "Strip 733", "Strip 734", "Strip 735", "Strip 736", "Strip 737", "Strip 738", "Strip 739", "Strip 740", "Strip 741", "Strip 742", "Strip 743", "Strip 744", "Strip 745", "Strip 746", "Strip 747", "Strip 748", "Strip 749", "Strip 750", "Strip 751", "Strip 752", "Strip 753", "Strip 754", "Strip 755", "Strip 756", "Strip 757", "Strip 758", "Strip 759", "Strip 760", "Strip 761", "Strip 762", "Strip 763", "Strip 764", "Strip 765", "Strip 766", "Strip 767", "Strip 768", "Strip 769", "Strip 770", "Strip 771", "Strip 772", "Strip 773", "Strip 774", "Strip 775", "Strip 776", "Strip 777", "Strip 778", "Strip 779", "Strip 780", "Strip 781", "Strip 782", "Strip 783", "Strip 784", "Strip 785", "Strip 786", "Strip 787", "Strip 788", "Strip 789", "Strip 790", "Strip 791", "Strip 792", "Strip 793", "Strip 794", "Strip 795", "Strip 796", "Strip 797", "Strip 798", "Strip 799", "Strip 800", "Strip 801", "Strip 802", "Strip 803", "Strip 804", "Strip 805", "Strip 806", "Strip 807", "Strip 808", "Strip 809", "Strip 810", "Strip 811", "Strip 812", "Strip 813", "Strip 814", "Strip 815", "Strip 816", "Strip 817", "Strip 818", "Strip 819", "Strip 820", "Strip 821", "Strip 822", "Strip 823", "Strip 824", "Strip 825", "Strip 826", "Strip 827", "Strip 828", "Strip 829", "Strip 830", "Strip 831", "Strip 832", "Strip 833", "Strip 834", "Strip 835", "Strip 836", "Strip 837", "Strip 838", "Strip 839", "Strip 840", "Strip 841", "Strip 842", "Strip 843", "Strip 844", "Strip 845", "Strip 846", "Strip 847", "Strip 848", "Strip 849", "Strip 850", "Strip 851", "Strip 852", "Strip 853", "Strip 854", "Strip 855", "Strip 856", "Strip 857", "Strip 858", "Strip 859", "Strip 860", "Strip 861", "Strip 862", "Strip 863", "Strip 864", "Strip 865", "Strip 866", "Strip 867", "Strip 868", "Strip 869", "Strip 870", "Strip 871", "Strip 872", "Strip 873", "Strip 874", "Strip 875", "Strip 876", "Strip 877", "Strip 878", "Strip 879", "Strip 880", "Strip 881", "Strip 882", "Strip 883", "Strip 884", "Strip 885", "Strip 886", "Strip 887", "Strip 888", "Strip 889", "Strip 890", "Strip 891", "Strip 892", "Strip 893", "Strip 894", "Strip 895", "Strip 896", "Strip 897", "Strip 898", "Strip 899", "Strip 900", "Strip 901", "Strip 902", "Strip 903", "Strip 904", "Strip 905", "Strip 906", "Strip 907", "Strip 908", "Strip 909", "Strip 910", "Strip 911", "Strip 912", "Strip 913", "Strip 914", "Strip 915", "Strip 916", "Strip 917", "Strip 918", "Strip 919", "Strip 920", "Strip 921", "Strip 922", "Strip 923", "Strip 924", "Strip 925", "Strip 926", "Strip 927", "Strip 928", "Strip 929", "Strip 930", "Strip 931", "Strip 932", "Strip 933", "Strip 934", "Strip 935", "Strip 936", "Strip 937", "Strip 938", "Strip 939", "Strip 940", "Strip 941", "Strip 942", "Strip 943", "Strip 944", "Strip 945", "Strip 946", "Strip 947", "Strip 948", "Strip 949", "Strip 950", "Strip 951", "Strip 952", "Strip 953", "Strip 954", "Strip 955", "Strip 956", "Strip 957", "Strip 958", "Strip 959", "Strip 960", "Strip 961", "Strip 962", "Strip 963", "Strip 964", "Strip 965", "Strip 966", "Strip 967", "Strip 968", "Strip 969", "Strip 970", "Strip 971", "Strip 972", "Strip 973", "Strip 974", "Strip 975", "Strip 976", "Strip 977", "Strip 978", "Strip 979", "Strip 980", "Strip 981", "Strip 982", "Strip 983", "Strip 984", "Strip 985", "Strip 986", "Strip 987", "Strip 988", "Strip 989", "Strip 990", "Strip 991", "Strip 992", "Strip 993", "Strip 994", "Strip 995", "Strip 996", "Strip 997", "Strip 998", "Strip 999", "Strip 1000", "Strip 1001", "Strip 1002", "Strip 1003", "Strip 1004", "Strip 1005", "Strip 1006", "Strip 1007", "Strip 1008", "Strip 1009", "Strip 1010", "Strip 1011", "Strip 1012", "Strip 1013", "Strip 1014", "Strip 1015", "Strip 1016", "Strip 1017", "Strip 1018", "Strip 1019", "Strip 1020", "Strip 1021", "Strip 1022", "Strip 1023", "Strip 1024", "Strip 1025", "Strip 1026", "Strip 1027", "Strip 1028", "Strip 1029", "Strip 1030", "Strip 1031", "Strip 1032", "Strip 1033", "Strip 1034", "Strip 1035", "Strip 1036", "Strip 1037", "Strip 1038", "Strip 1039", "Strip 1040", "Strip 1041", "Strip 1042", "Strip 1043", "Strip 1044", "Strip 1045", "Strip 1046", "Strip 1047", "Strip 1048", "Strip 1049", "Strip 1050", "Strip 1051", "Strip 1052", "Strip 1053", "Strip 1054", "Strip 1055", "Strip 1056", "Strip 1057", "Strip 1058", "Strip 1059", "Strip 1060", "Strip 1061", "Strip 1062", "Strip 1063", "Strip 1064", "Strip 1065", "Strip 1066", "Strip 1067", "Strip 1068", "Strip 1069", "Strip 1070", "Strip 1071", "Strip 1072", "Strip 1073", "Strip 1074", "Strip 1075", "Strip 1076", "Strip 1077", "Strip 1078", "Strip 1079", "Strip 1080", "Strip 1081", "Strip 1082", "Strip 1083", "Strip 1084", "Strip 1085", "Strip 1086", "Strip 1087", "Strip 1088", "Strip 1089", "Strip 1090", "Strip 1091", "Strip 1092", "Strip 1093", "Strip 1094", "Strip 1095", "Strip 1096", "Strip 1097", "Strip 1098", "Strip 1099", "Strip 1100", "Strip 1101", "Strip 1102", "Strip 1103", "Strip 1104", "Strip 1105", "Strip 1106", "Strip 1107", "Strip 1108", "Strip 1109", "Strip 1110", "Strip 1111", "Strip 1112", "Strip 1113", "Strip 1114", "Strip 1115", "Strip 1116", "Strip 1117", "Strip 1118", "Strip 1119", "Strip 1120", "Strip 1121", "Strip 1122", "Strip 1123", "Strip 1124", "Strip 1125", "Strip 1126", "Strip 1127", "Strip 1128", "Strip 1129", "Strip 1130", "Strip 1131", "Strip 1132", "Strip 1133", "Strip 1134", "Strip 1135", "Strip 1136", "Strip 1137", "Strip 1138", "Strip 1139", "Strip 1140", "Strip 1141", "Strip 1142", "Strip 1143", "Strip 1144", "Strip 1145", "Strip 1146", "Strip 1147", "Strip 1148", "Strip 1149", "Strip 1150", "Strip 1151", "Strip 1152", "Strip 1153", "Strip 1154", "Strip 1155", "Strip 1156", "Strip 1157", "Strip 1158", "Strip 1159", "Strip 1160", "Strip 1161", "Strip 1162", "Strip 1163", "Strip 1164", "Strip 1165", "Strip 1166", "Strip 1167", "Strip 1168", "Strip 1169", "Strip 1170", "Strip 1171", "Strip 1172", "Strip 1173", "Strip 1174", "Strip 1175", "Strip 1176", "Strip 1177", "Strip 1178", "Strip 1179", "Strip 1180", "Strip 1181", "Strip 1182", "Strip 1183", "Strip 1184", "Strip 1185", "Strip 1186", "Strip 1187", "Strip 1188", "Strip 1189", "Strip 1190", "Strip 1191", "Strip 1192", "Strip 1193", "Strip 1194", "Strip 1195", "Strip 1196", "Strip 1197", "Strip 1198", "Strip 1199", "Strip 1200", "Strip 1201", "Strip 1202", "Strip 1203", "Strip 1204", "Strip 1205", "Strip 1206", "Strip 1207", "Strip 1208", "Strip 1209", "Strip 1210", "Strip 1211", "Strip 1212", "Strip 1213", "Strip 1214", "Strip 1215", "Strip 1216", "Strip 1217", "Strip 1218", "Strip 1219", "Strip 1220", "Strip 1221", "Strip 1222", "Strip 1223", "Strip 1224", "Strip 1225", "Strip 1226", "Strip 1227", "Strip 1228", "Strip 1229", "Strip 1230", "Strip 1231", "Strip 1232", "Strip 1233", "Strip 1234", "Strip 1235", "Strip 1236", "Strip 1237", "Strip 1238", "Strip 1239", "Strip 1240", "Strip 1241", "Strip 1242", "Strip 1243", "Strip 1244", "Strip 1245", "Strip 1246", "Strip 1247", "Strip 1248", "Strip 1249", "Strip 1250", "Strip 1251", "Strip 1252", "Strip 1253", "Strip 1254", "Strip 1255", "Strip 1256", "Strip 1257", "Strip 1258", "Strip 1259", "Strip 1260", "Strip 1261", "Strip 1262", "Strip 1263", "Strip 1264", "Strip 1265", "Strip 1266", "Strip 1267", "Strip 1268", "Strip 1269", "Strip 1270", "Strip 1271", "Strip 1272", "Strip 1273", "Strip 1274", "Strip 1275", "Strip 1276", "Strip 1277", "Strip 1278", "Strip 1279", "Strip 1280", "Strip 1281", "Strip 1282", "Strip 1283", "Strip 1284", "Strip 1285", "Strip 1286", "Strip 1287", "Strip 1288", "Strip 1289", "Strip 1290", "Strip 1291", "Strip 1292", "Strip 1293", "Strip 1294", "Strip 1295", "Strip 1296", "Strip 1297", "Strip 1298", "Strip 1299", "Strip 1300", "Strip 1301", "Strip 1302", "Strip 1303", "Strip 1304", "Strip 1305", "Strip 1306", "Strip 1307", "Strip 1308", "Strip 1309", "Strip 1310", "Strip 1311", "Strip 1312", "Strip 1313", "Strip 1314", "Strip 1315", "Strip 1316", "Strip 1317", "Strip 1318", "Strip 1319", "Strip 1320", "Strip 1321", "Strip 1322", "Strip 1323", "Strip 1324", "Strip 1325", "Strip 1326", "Strip 1327", "Strip 1328", "Strip 1329", "Strip 1330", "Strip 1331", "Strip 1332", "Strip 1333", "Strip 1334", "Strip 1335", "Strip 1336", "Strip 1337", "Strip 1338", "Strip 1339", "Strip 1340", "Strip 1341", "Strip 1342", "Strip 1343", "Strip 1344", "Strip 1345", "Strip 1346", "Strip 1347", "Strip 1348", "Strip 1349", "Strip 1350", "Strip 1351", "Strip 1352", "Strip 1353", "Strip 1354", "Strip 1355", "Strip 1356", "Strip 1357", "Strip 1358", "Strip 1359", "Strip 1360", "Strip 1361", "Strip 1362", "Strip 1363", "Strip 1364", "Strip 1365", "Strip 1366", "Strip 1367", "Strip 1368", "Strip 1369", "Strip 1370", "Strip 1371", "Strip 1372", "Strip 1373", "Strip 1374", "Strip 1375", "Strip 1376", "Strip 1377", "Strip 1378", "Strip 1379", "Strip 1380", "Strip 1381", "Strip 1382", "Strip 1383", "Strip 1384", "Strip 1385", "Strip 1386", "Strip 1387", "Strip 1388", "Strip 1389", "Strip 1390", "Strip 1391", "Strip 1392", "Strip 1393", "Strip 1394", "Strip 1395", "Strip 1396", "Strip 1397", "Strip 1398", "Strip 1399", "Strip 1400", "Strip 1401", "Strip 1402", "Strip 1403", "Strip 1404", "Strip 1405", "Strip 1406", "Strip 1407", "Strip 1408", "Strip 1409"]
  in  "From2":u16(ring) items=["Strip 0", "Strip 1", "Strip 2", "Strip 3", "Strip 4", "Strip 5", "Strip 6", "Strip 7", "Strip 8", "Strip 9", "Strip 10", "Strip 11", "Strip 12", "Strip 13", "Strip 14", "Strip 15", "Strip 16", "Strip 17", "Strip 18", "Strip 19", "Strip 20", "Strip 21", "Strip 22", "Strip 23", "Strip 24", "Strip 25", "Strip 26", "Strip 27", "Strip 28", "Strip 29", "Strip 30", "Strip 31", "Strip 32", "Strip 33", "Strip 34", "Strip 35", "Strip 36", "Strip 37", "Strip 38", "Strip 39", "Strip 40", "Strip 41", "Strip 42", "Strip 43", "Strip 44", "Strip 45", "Strip 46", "Strip 47", "Strip 48", "Strip 49", "Strip 50", "Strip 51", "Strip 52", "Strip 53", "Strip 54", "Strip 55", "Strip 56", "Strip 57", "Strip 58", "Strip 59", "Strip 60", "Strip 61", "Strip 62", "Strip 63", "Strip 64", "Strip 65", "Strip 66", "Strip 67", "Strip 68", "Strip 69", "Strip 70", "Strip 71", "Strip 72", "Strip 73", "Strip 74", "Strip 75", "Strip 76", "Strip 77", "Strip 78", "Strip 79", "Strip 80", "Strip 81", "Strip 82", "Strip 83", "Strip 84", "Strip 85", "Strip 86", "Strip 87", "Strip 88", "Strip 89", "Strip 90", "Strip 91", "Strip 92", "Strip 93", "Strip 94", "Strip 95", "Strip 96", "Strip 97", "Strip 98", "Strip 99", "Strip 100", "Strip 101", "Strip 102", "Strip 103", "Strip 104", "Strip 105", "Strip 106", "Strip 107", "Strip 108", "Strip 109", "Strip 110", "Strip 111", "Strip 112", "Strip 113", "Strip 114", "Strip 115", "Strip 116", "Strip 117", "Strip 118", "Strip 119", "Strip 120", "Strip 121", "Strip 122", "Strip 123", "Strip 124", "Strip 125", "Strip 126", "Strip 127", "Strip 128", "Strip 129", "Strip 130", "Strip 131", "Strip 132", "Strip 133", "Strip 134", "Strip 135", "Strip 136", "Strip 137", "Strip 138", "Strip 139", "Strip 140", "Strip 141", "Strip 142", "Strip 143", "Strip 144", "Strip 145", "Strip 146", "Strip 147", "Strip 148", "Strip 149", "Strip 150", "Strip 151", "Strip 152", "Strip 153", "Strip 154", "Strip 155", "Strip 156", "Strip 157", "Strip 158", "Strip 159", "Strip 160", "Strip 161", "Strip 162", "Strip 163", "Strip 164", "Strip 165", "Strip 166", "Strip 167", "Strip 168", "Strip 169", "Strip 170", "Strip 171", "Strip 172", "Strip 173", "Strip 174", "Strip 175", "Strip 176", "Strip 177", "Strip 178", "Strip 179", "Strip 180", "Strip 181", "Strip 182", "Strip 183", "Strip 184", "Strip 185", "Strip 186", "Strip 187", "Strip 188", "Strip 189", "Strip 190", "Strip 191", "Strip 192", "Strip 193", "Strip 194", "Strip 195", "Strip 196", "Strip 197", "Strip 198", "Strip 199", "Strip 200", "Strip 201", "Strip 202", "Strip 203", "Strip 204", "Strip 205", "Strip 206", "Strip 207", "Strip 208", "Strip 209", "Strip 210", "Strip 211", "Strip 212", "Strip 213", "Strip 214", "Strip 215", "Strip 216", "Strip 217", "Strip 218", "Strip 219", "Strip 220", "Strip 221", "Strip 222", "Strip 223", "Strip 224", "Strip 225", "Strip 226", "Strip 227", "Strip 228", "Strip 229", "Strip 230", "Strip 231", "Strip 232", "Strip 233", "Strip 234", "Strip 235", "Strip 236", "Strip 237", "Strip 238", "Strip 239", "Strip 240", "Strip 241", "Strip 242", "Strip 243", "Strip 244", "Strip 245", "Strip 246", "Strip 247", "Strip 248", "Strip 249", "Strip 250", "Strip 251", "Strip 252", "Strip 253", "Strip 254", "Strip 255", "Strip 256", "Strip 257", "Strip 258", "Strip 259", "Strip 260", "Strip 261", "Strip 262", "Strip 263", "Strip 264", "Strip 265", "Strip 266", "Strip 267", "Strip 268", "Strip 269", "Strip 270", "Strip 271", "Strip 272", "Strip 273", "Strip 274", "Strip 275", "Strip 276", "Strip 277", "Strip 278", "Strip 279", "Strip 280", "Strip 281", "Strip 282", "Strip 283", "Strip 284", "Strip 285", "Strip 286", "Strip 287", "Strip 288", "Strip 289", "Strip 290", "Strip 291", "Strip 292", "Strip 293", "Strip 294", "Strip 295", "Strip 296", "Strip 297", "Strip 298", "Strip 299", "Strip 300", "Strip 301", "Strip 302", "Strip 303", "Strip 304", "Strip 305", "Strip 306", "Strip 307", "Strip 308", "Strip 309", "Strip 310", "Strip 311", "Strip 312", "Strip 313", "Strip 314", "Strip 315", "Strip 316", "Strip 317", "Strip 318", "Strip 319", "Strip 320", "Strip 321", "Strip 322", "Strip 323", "Strip 324", "Strip 325", "Strip 326", "Strip 327", "Strip 328", "Strip 329", "Strip 330", "Strip 331", "Strip 332", "Strip 333", "Strip 334", "Strip 335", "Strip 336", "Strip 337", "Strip 338", "Strip 339", "Strip 340", "Strip 341", "Strip 342", "Strip 343", "Strip 344", "Strip 345", "Strip 346", "Strip 347", "Strip 348", "Strip 349", "Strip 350", "Strip 351", "Strip 352", "Strip 353", "Strip 354", "Strip 355", "Strip 356", "Strip 357", "Strip 358", "Strip 359", "Strip 360", "Strip 361", "Strip 362", "Strip 363", "Strip 364", "Strip 365", "Strip 366", "Strip 367", "Strip 368", "Strip 369", "Strip 370", "Strip 371", "Strip 372", "Strip 373", "Strip 374", "Strip 375", "Strip 376", "Strip 377", "Strip 378", "Strip 379", "Strip 380", "Strip 381", "Strip 382", "Strip 383", "Strip 384", "Strip 385", "Strip 386", "Strip 387", "Strip 388", "Strip 389", "Strip 390", "Strip 391", "Strip 392", "Strip 393", "Strip 394", "Strip 395", "Strip 396", "Strip 397", "Strip 398", "Strip 399", "Strip 400", "Strip 401", "Strip 402", "Strip 403", "Strip 404", "Strip 405", "Strip 406", "Strip 407", "Strip 408", "Strip 409", "Strip 410", "Strip 411", "Strip 412", "Strip 413", "Strip 414", "Strip 415", "Strip 416", "Strip 417", "Strip 418", "Strip 419", "Strip 420", "Strip 421", "Strip 422", "Strip 423", "Strip 424", "Strip 425", "Strip 426", "Strip 427", "Strip 428", "Strip 429", "Strip 430", "Strip 431", "Strip 432", "Strip 433", "Strip 434", "Strip 435", "Strip 436", "Strip 437", "Strip 438", "Strip 439", "Strip 440", "Strip 441", "Strip 442", "Strip 443", "Strip 444", "Strip 445", "Strip 446", "Strip 447", "Strip 448", "Strip 449", "Strip 450", "Strip 451", "Strip 452", "Strip 453", "Strip 454", "Strip 455", "Strip 456", "Strip 457", "Strip 458", "Strip 459", "Strip 460", "Strip 461", "Strip 462", "Strip 463", "Strip 464", "Strip 465", "Strip 466", "Strip 467", "Strip 468", "Strip 469", "Strip 470", "Strip 471", "Strip 472", "Strip 473", "Strip 474", "Strip 475", "Strip 476", "Strip 477", "Strip 478", "Strip 479", "Strip 480", "Strip 481", "Strip 482", "Strip 483", "Strip 484", "Strip 485", "Strip 486", "Strip 487", "Strip 488", "Strip 489", "Strip 490", "Strip 491", "Strip 492", "Strip 493", "Strip 494", "Strip 495", "Strip 496", "Strip 497", "Strip 498", "Strip 499", "Strip 500", "Strip 501", "Strip 502", "Strip 503", "Strip 504", "Strip 505", "Strip 506", "Strip 507", "Strip 508", "Strip 509", "Strip 510", "Strip 511", "Strip 512", "Strip 513", "Strip 514", "Strip 515", "Strip 516", "Strip 517", "Strip 518", "Strip 519", "Strip 520", "Strip 521", "Strip 522", "Strip 523", "Strip 524", "Strip 525", "Strip 526", "Strip 527", "Strip 528", "Strip 529", "Strip 530", "Strip 531", "Strip 532", "Strip 533", "Strip 534", "Strip 535", "Strip 536", "Strip 537", "Strip 538", "Strip 539", "Strip 540", "Strip 541", "Strip 542", "Strip 543", "Strip 544", "Strip 545", "Strip 546", "Strip 547", "Strip 548", "Strip 549", "Strip 550", "Strip 551", "Strip 552", "Strip 553", "Strip 554", "Strip 555", "Strip 556", "Strip 557", "Strip 558", "Strip 559", "Strip 560", "Strip 561", "Strip 562", "Strip 563", "Strip 564", "Strip 565", "Strip 566", "Strip 567", "Strip 568", "Strip 569", "Strip 570", "Strip 571", "Strip 572", "Strip 573", "Strip 574", "Strip 575", "Strip 576", "Strip 577", "Strip 578", "Strip 579", "Strip 580", "Strip 581", "Strip 582", "Strip 583", "Strip 584", "Strip 585", "Strip 586", "Strip 587", "Strip 588", "Strip 589", "Strip 590", "Strip 591", "Strip 592", "Strip 593", "Strip 594", "Strip 595", "Strip 596", "Strip 597", "Strip 598", "Strip 599", "Strip 600", "Strip 601", "Strip 602", "Strip 603", "Strip 604", "Strip 605", "Strip 606", "Strip 607", "Strip 608", "Strip 609", "Strip 610", "Strip 611", "Strip 612", "Strip 613", "Strip 614", "Strip 615", "Strip 616", "Strip 617", "Strip 618", "Strip 619", "Strip 620", "Strip 621", "Strip 622", "Strip 623", "Strip 624", "Strip 625", "Strip 626", "Strip 627", "Strip 628", "Strip 629", "Strip 630", "Strip 631", "Strip 632", "Strip 633", "Strip 634", "Strip 635", "Strip 636", "Strip 637", "Strip 638", "Strip 639", "Strip 640", "Strip 641", "Strip 642", "Strip 643", "Strip 644", "Strip 645", "Strip 646", "Strip 647", "Strip 648", "Strip 649", "Strip 650", "Strip 651", "Strip 652", "Strip 653", "Strip 654", "Strip 655", "Strip 656", "Strip 657", "Strip 658", "Strip 659", "Strip 660", "Strip 661", "Strip 662", "Strip 663", "Strip 664", "Strip 665", "Strip 666", "Strip 667", "Strip 668", "Strip 669", "Strip 670", "Strip 671", "Strip 672", "Strip 673", "Strip 674", "Strip 675", "Strip 676", "Strip 677", "Strip 678", "Strip 679", "Strip 680", "Strip 681", "Strip 682", "Strip 683", "Strip 684", "Strip 685", "Strip 686", "Strip 687", "Strip 688", "Strip 689", "Strip 690", "Strip 691", "Strip 692", "Strip 693", "Strip 694", "Strip 695", "Strip 696", "Strip 697", "Strip 698", "Strip 699", "Strip 700", "Strip 701", "Strip 702", "Strip 703", "Strip 704", "Strip 705", "Strip 706", "Strip 707", "Strip 708", "Strip 709", "Strip 710", "Strip 711", "Strip 712", "Strip 713", "Strip 714", "Strip 715", "Strip 716", "Strip 717", "Strip 718", "Strip 719", "Strip 720", "Strip 721", "Strip 722", "Strip 723", "Strip 724", "Strip 725", "Strip 726", "Strip 727", "Strip 728", "Strip 729", "Strip 730", "Strip 731", "Strip 732", "Strip 733", "Strip 734", "Strip 735", "Strip 736", "Strip 737", "Strip 738", "Strip 739", "Strip 740", "Strip 741", "Strip 742", "Strip 743", "Strip 744", "Strip 745", "Strip 746", "Strip 747", "Strip 748", "Strip 749", "Strip 750", "Strip 751", "Strip 752", "Strip 753", "Strip 754", "Strip 755", "Strip 756", "Strip 757", "Strip 758", "Strip 759", "Strip 760", "Strip 761", "Strip 762", "Strip 763", "Strip 764", "Strip 765", "Strip 766", "Strip 767", "Strip 768", "Strip 769", "Strip 770", "Strip 771", "Strip 772", "Strip 773", "Strip 774", "Strip 775", "Strip 776", "Strip 777", "Strip 778", "Strip 779", "Strip 780", "Strip 781", "Strip 782", "Strip 783", "Strip 784", "Strip 785", "Strip 786", "Strip 787", "Strip 788", "Strip 789", "Strip 790", "Strip 791", "Strip 792", "Strip 793", "Strip 794", "Strip 795", "Strip 796", "Strip 797", "Strip 798", "Strip 799", "Strip 800", "Strip 801", "Strip 802", "Strip 803", "Strip 804", "Strip 805", "Strip 806", "Strip 807", "Strip 808", "Strip 809", "Strip 810", "Strip 811", "Strip 812", "Strip 813", "Strip 814", "Strip 815", "Strip 816", "Strip 817", "Strip 818", "Strip 819", "Strip 820", "Strip 821", "Strip 822", "Strip 823", "Strip 824", "Strip 825", "Strip 826", "Strip 827", "Strip 828", "Strip 829", "Strip 830", "Strip 831", "Strip 832", "Strip 833", "Strip 834", "Strip 835", "Strip 836", "Strip 837", "Strip 838", "Strip 839", "Strip 840", "Strip 841", "Strip 842", "Strip 843", "Strip 844", "Strip 845", "Strip 846", "Strip 847", "Strip 848", "Strip 849", "Strip 850", "Strip 851", "Strip 852", "Strip 853", "Strip 854", "Strip 855", "Strip 856", "Strip 857", "Strip 858", "Strip 859", "Strip 860", "Strip 861", "Strip 862", "Strip 863", "Strip 864", "Strip 865", "Strip 866", "Strip 867", "Strip 868", "Strip 869", "Strip 870", "Strip 871", "Strip 872", "Strip 873", "Strip 874", "Strip 875", "Strip 876", "Strip 877", "Strip 878", "Strip 879", "Strip 880", "Strip 881", "Strip 882", "Strip 883", "Strip 884", "Strip 885", "Strip 886", "Strip 887", "Strip 888", "Strip 889", "Strip 890", "Strip 891", "Strip 892", "Strip 893", "Strip 894", "Strip 895", "Strip 896", "Strip 897", "Strip 898", "Strip 899", "Strip 900", "Strip 901", "Strip 902", "Strip 903", "Strip 904", "Strip 905", "Strip 906", "Strip 907", "Strip 908", "Strip 909", "Strip 910", "Strip 911", "Strip 912", "Strip 913", "Strip 914", "Strip 915", "Strip 916", "Strip 917", "Strip 918", "Strip 919", "Strip 920", "Strip 921", "Strip 922", "Strip 923", "Strip 924", "Strip 925", "Strip 926", "Strip 927", "Strip 928", "Strip 929", "Strip 930", "Strip 931", "Strip 932", "Strip 933", "Strip 934", "Strip 935", "Strip 936", "Strip 937", "Strip 938", "Strip 939", "Strip 940", "Strip 941", "Strip 942", "Strip 943", "Strip 944", "Strip 945", "Strip 946", "Strip 947", "Strip 948", "Strip 949", "Strip 950", "Strip 951", "Strip 952", "Strip 953", "Strip 954", "Strip 955", "Strip 956", "Strip 957", "Strip 958", "Strip 959", "Strip 960", "Strip 961", "Strip 962", "Strip 963", "Strip 964", "Strip 965", "Strip 966", "Strip 967", "Strip 968", "Strip 969", "Strip 970", "Strip 971", "Strip 972", "Strip 973", "Strip 974", "Strip 975", "Strip 976", "Strip 977", "Strip 978", "Strip 979", "Strip 980", "Strip 981", "Strip 982", "Strip 983", "Strip 984", "Strip 985", "Strip 986", "Strip 987", "Strip 988", "Strip 989", "Strip 990", "Strip 991", "Strip 992", "Strip 993", "Strip 994", "Strip 995", "Strip 996", "Strip 997", "Strip 998", "Strip 999", "Strip 1000", "Strip 1001", "Strip 1002", "Strip 1003", "Strip 1004", "Strip 1005", "Strip 1006", "Strip 1007", "Strip 1008", "Strip 1009", "Strip 1010", "Strip 1011", "Strip 1012", "Strip 1013", "Strip 1014", "Strip 1015", "Strip 1016", "Strip 1017", "Strip 1018", "Strip 1019", "Strip 1020", "Strip 1021", "Strip 1022", "Strip 1023", "Strip 1024", "Strip 1025", "Strip 1026", "Strip 1027", "Strip 1028", "Strip 1029", "Strip 1030", "Strip 1031", "Strip 1032", "Strip 1033", "Strip 1034", "Strip 1035", "Strip 1036", "Strip 1037", "Strip 1038", "Strip 1039", "Strip 1040", "Strip 1041", "Strip 1042", "Strip 1043", "Strip 1044", "Strip 1045", "Strip 1046", "Strip 1047", "Strip 1048", "Strip 1049", "Strip 1050", "Strip 1051", "Strip 1052", "Strip 1053", "Strip 1054", "Strip 1055", "Strip 1056", "Strip 1057", "Strip 1058", "Strip 1059", "Strip 1060", "Strip 1061", "Strip 1062", "Strip 1063", "Strip 1064", "Strip 1065", "Strip 1066", "Strip 1067", "Strip 1068", "Strip 1069", "Strip 1070", "Strip 1071", "Strip 1072", "Strip 1073", "Strip 1074", "Strip 1075", "Strip 1076", "Strip 1077", "Strip 1078", "Strip 1079", "Strip 1080", "Strip 1081", "Strip 1082", "Strip 1083", "Strip 1084", "Strip 1085", "Strip 1086", "Strip 1087", "Strip 1088", "Strip 1089", "Strip 1090", "Strip 1091", "Strip 1092", "Strip 1093", "Strip 1094", "Strip 1095", "Strip 1096", "Strip 1097", "Strip 1098", "Strip 1099", "Strip 1100", "Strip 1101", "Strip 1102", "Strip 1103", "Strip 1104", "Strip 1105", "Strip 1106", "Strip 1107", "Strip 1108", "Strip 1109", "Strip 1110", "Strip 1111", "Strip 1112", "Strip 1113", "Strip 1114", "Strip 1115", "Strip 1116", "Strip 1117", "Strip 1118", "Strip 1119", "Strip 1120", "Strip 1121", "Strip 1122", "Strip 1123", "Strip 1124", "Strip 1125", "Strip 1126", "Strip 1127", "Strip 1128", "Strip 1129", "Strip 1130", "Strip 1131", "Strip 1132", "Strip 1133", "Strip 1134", "Strip 1135", "Strip 1136", "Strip 1137", "Strip 1138", "Strip 1139", "Strip 1140", "Strip 1141", "Strip 1142", "Strip 1143", "Strip 1144", "Strip 1145", "Strip 1146", "Strip 1147", "Strip 1148", "Strip 1149", "Strip 1150", "Strip 1151", "Strip 1152", "Strip 1153"]
  in  "From 1":u16(ring) caption="From" items=["Strip 0", "Strip 1", "Strip 2", "Strip 3", "Strip 4", "Strip 5", "Strip 6", "Strip 7", "Strip 8", "Strip 9", "Strip 10", "Strip 11", "Strip 12", "Strip 13", "Strip 14", "Strip 15", "Strip 16", "Strip 17", "Strip 18", "Strip 19", "Strip 20", "Strip 21", "Strip 22", "Strip 23", "Strip 24", "Strip 25", "Strip 26", "Strip 27", "Strip 28", "Strip 29", "Strip 30", "Strip 31", "Strip 32", "Strip 33", "Strip 34", "Strip 35", "Strip 36", "Strip 37", "Strip 38", "Strip 39", "Strip 40", "Strip 41", "Strip 42", "Strip 43", "Strip 44", "Strip 45", "Strip 46", "Strip 47", "Strip 48", "Strip 49", "Strip 50", "Strip 51", "Strip 52", "Strip 53", "Strip 54", "Strip 55", "Strip 56", "Strip 57", "Strip 58", "Strip 59", "Strip 60", "Strip 61", "Strip 62", "Strip 63", "Strip 64", "Strip 65", "Strip 66", "Strip 67", "Strip 68", "Strip 69", "Strip 70", "Strip 71", "Strip 72", "Strip 73", "Strip 74", "Strip 75", "Strip 76", "Strip 77", "Strip 78", "Strip 79", "Strip 80", "Strip 81", "Strip 82", "Strip 83", "Strip 84", "Strip 85", "Strip 86", "Strip 87", "Strip 88", "Strip 89", "Strip 90", "Strip 91", "Strip 92", "Strip 93", "Strip 94", "Strip 95", "Strip 96", "Strip 97", "Strip 98", "Strip 99", "Strip 100", "Strip 101", "Strip 102", "Strip 103", "Strip 104", "Strip 105", "Strip 106", "Strip 107", "Strip 108", "Strip 109", "Strip 110", "Strip 111", "Strip 112", "Strip 113", "Strip 114", "Strip 115", "Strip 116", "Strip 117", "Strip 118", "Strip 119", "Strip 120", "Strip 121", "Strip 122", "Strip 123", "Strip 124", "Strip 125", "Strip 126", "Strip 127", "Strip 128", "Strip 129", "Strip 130", "Strip 131", "Strip 132", "Strip 133", "Strip 134", "Strip 135", "Strip 136", "Strip 137", "Strip 138", "Strip 139", "Strip 140", "Strip 141", "Strip 142", "Strip 143", "Strip 144", "Strip 145", "Strip 146", "Strip 147", "Strip 148", "Strip 149", "Strip 150", "Strip 151", "Strip 152", "Strip 153", "Strip 154", "Strip 155", "Strip 156", "Strip 157", "Strip 158", "Strip 159", "Strip 160", "Strip 161", "Strip 162", "Strip 163", "Strip 164", "Strip 165", "Strip 166", "Strip 167", "Strip 168", "Strip 169", "Strip 170", "Strip 171", "Strip 172", "Strip 173", "Strip 174", "Strip 175", "Strip 176", "Strip 177", "Strip 178", "Strip 179", "Strip 180", "Strip 181", "Strip 182", "Strip 183", "Strip 184", "Strip 185", "Strip 186", "Strip 187", "Strip 188", "Strip 189", "Strip 190", "Strip 191", "Strip 192", "Strip 193", "Strip 194", "Strip 195", "Strip 196", "Strip 197", "Strip 198", "Strip 199", "Strip 200", "Strip 201", "Strip 202", "Strip 203", "Strip 204", "Strip 205", "Strip 206", "Strip 207", "Strip 208", "Strip 209", "Strip 210", "Strip 211", "Strip 212", "Strip 213", "Strip 214", "Strip 215", "Strip 216", "Strip 217", "Strip 218", "Strip 219", "Strip 220", "Strip 221", "Strip 222", "Strip 223", "Strip 224", "Strip 225", "Strip 226", "Strip 227", "Strip 228", "Strip 229", "Strip 230", "Strip 231", "Strip 232", "Strip 233", "Strip 234", "Strip 235", "Strip 236", "Strip 237", "Strip 238", "Strip 239", "Strip 240", "Strip 241", "Strip 242", "Strip 243", "Strip 244", "Strip 245", "Strip 246", "Strip 247", "Strip 248", "Strip 249", "Strip 250", "Strip 251", "Strip 252", "Strip 253", "Strip 254", "Strip 255", "Strip 256", "Strip 257", "Strip 258", "Strip 259", "Strip 260", "Strip 261", "Strip 262", "Strip 263", "Strip 264", "Strip 265", "Strip 266", "Strip 267", "Strip 268", "Strip 269", "Strip 270", "Strip 271", "Strip 272", "Strip 273", "Strip 274", "Strip 275", "Strip 276", "Strip 277", "Strip 278", "Strip 279", "Strip 280", "Strip 281", "Strip 282", "Strip 283", "Strip 284", "Strip 285", "Strip 286", "Strip 287", "Strip 288", "Strip 289", "Strip 290", "Strip 291", "Strip 292", "Strip 293", "Strip 294", "Strip 295", "Strip 296", "Strip 297", "Strip 298", "Strip 299", "Strip 300", "Strip 301", "Strip 302", "Strip 303", "Strip 304", "Strip 305", "Strip 306", "Strip 307", "Strip 308", "Strip 309", "Strip 310", "Strip 311", "Strip 312", "Strip 313", "Strip 314", "Strip 315", "Strip 316", "Strip 317", "Strip 318", "Strip 319", "Strip 320", "Strip 321", "Strip 322", "Strip 323", "Strip 324", "Strip 325", "Strip 326", "Strip 327", "Strip 328", "Strip 329", "Strip 330", "Strip 331", "Strip 332", "Strip 333", "Strip 334", "Strip 335", "Strip 336", "Strip 337", "Strip 338", "Strip 339", "Strip 340", "Strip 341", "Strip 342", "Strip 343", "Strip 344", "Strip 345", "Strip 346", "Strip 347", "Strip 348", "Strip 349", "Strip 350", "Strip 351", "Strip 352", "Strip 353", "Strip 354", "Strip 355", "Strip 356", "Strip 357", "Strip 358", "Strip 359", "Strip 360", "Strip 361", "Strip 362", "Strip 363", "Strip 364", "Strip 365", "Strip 366", "Strip 367", "Strip 368", "Strip 369", "Strip 370", "Strip 371", "Strip 372", "Strip 373", "Strip 374", "Strip 375", "Strip 376", "Strip 377", "Strip 378", "Strip 379", "Strip 380", "Strip 381", "Strip 382", "Strip 383", "Strip 384", "Strip 385", "Strip 386", "Strip 387", "Strip 388", "Strip 389", "Strip 390", "Strip 391", "Strip 392", "Strip 393", "Strip 394", "Strip 395", "Strip 396", "Strip 397", "Strip 398", "Strip 399", "Strip 400", "Strip 401", "Strip 402", "Strip 403", "Strip 404", "Strip 405", "Strip 406", "Strip 407", "Strip 408", "Strip 409", "Strip 410", "Strip 411", "Strip 412", "Strip 413", "Strip 414", "Strip 415", "Strip 416", "Strip 417", "Strip 418", "Strip 419", "Strip 420", "Strip 421", "Strip 422", "Strip 423", "Strip 424", "Strip 425", "Strip 426", "Strip 427", "Strip 428", "Strip 429", "Strip 430", "Strip 431", "Strip 432", "Strip 433", "Strip 434", "Strip 435", "Strip 436", "Strip 437", "Strip 438", "Strip 439", "Strip 440", "Strip 441", "Strip 442", "Strip 443", "Strip 444", "Strip 445", "Strip 446", "Strip 447", "Strip 448", "Strip 449", "Strip 450", "Strip 451", "Strip 452", "Strip 453", "Strip 454", "Strip 455", "Strip 456", "Strip 457", "Strip 458", "Strip 459", "Strip 460", "Strip 461", "Strip 462", "Strip 463", "Strip 464", "Strip 465", "Strip 466", "Strip 467", "Strip 468", "Strip 469", "Strip 470", "Strip 471", "Strip 472", "Strip 473", "Strip 474", "Strip 475", "Strip 476", "Strip 477", "Strip 478", "Strip 479", "Strip 480", "Strip 481", "Strip 482", "Strip 483", "Strip 484", "Strip 485", "Strip 486", "Strip 487", "Strip 488", "Strip 489", "Strip 490", "Strip 491", "Strip 492", "Strip 493", "Strip 494", "Strip 495", "Strip 496", "Strip 497", "Strip 498", "Strip 499", "Strip 500", "Strip 501", "Strip 502", "Strip 503", "Strip 504", "Strip 505", "Strip 506", "Strip 507", "Strip 508", "Strip 509", "Strip 510", "Strip 511", "Strip 512", "Strip 513", "Strip 514", "Strip 515", "Strip 516", "Strip 517", "Strip 518", "Strip 519", "Strip 520", "Strip 521", "Strip 522", "Strip 523", "Strip 524", "Strip 525", "Strip 526", "Strip 527", "Strip 528", "Strip 529", "Strip 530", "Strip 531", "Strip 532", "Strip 533", "Strip 534", "Strip 535", "Strip 536", "Strip 537", "Strip 538", "Strip 539", "Strip 540", "Strip 541", "Strip 542", "Strip 543", "Strip 544", "Strip 545", "Strip 546", "Strip 547", "Strip 548", "Strip 549", "Strip 550", "Strip 551", "Strip 552", "Strip 553", "Strip 554", "Strip 555", "Strip 556", "Strip 557", "Strip 558", "Strip 559", "Strip 560", "Strip 561", "Strip 562", "Strip 563", "Strip 564", "Strip 565", "Strip 566", "Strip 567", "Strip 568", "Strip 569", "Strip 570", "Strip 571", "Strip 572", "Strip 573", "Strip 574", "Strip 575", "Strip 576", "Strip 577", "Strip 578", "Strip 579", "Strip 580", "Strip 581", "Strip 582", "Strip 583", "Strip 584", "Strip 585", "Strip 586", "Strip 587", "Strip 588", "Strip 589", "Strip 590", "Strip 591", "Strip 592", "Strip 593", "Strip 594", "Strip 595", "Strip 596", "Strip 597", "Strip 598", "Strip 599", "Strip 600", "Strip 601", "Strip 602", "Strip 603", "Strip 604", "Strip 605", "Strip 606", "Strip 607", "Strip 608", "Strip 609", "Strip 610", "Strip 611", "Strip 612", "Strip 613", "Strip 614", "Strip 615", "Strip 616", "Strip 617", "Strip 618", "Strip 619", "Strip 620", "Strip 621", "Strip 622", "Strip 623", "Strip 624", "Strip 625", "Strip 626", "Strip 627", "Strip 628", "Strip 629", "Strip 630", "Strip 631", "Strip 632", "Strip 633", "Strip 634", "Strip 635", "Strip 636", "Strip 637", "Strip 638", "Strip 639", "Strip 640", "Strip 641", "Strip 642", "Strip 643", "Strip 644", "Strip 645", "Strip 646", "Strip 647", "Strip 648", "Strip 649", "Strip 650", "Strip 651", "Strip 652", "Strip 653", "Strip 654", "Strip 655", "Strip 656", "Strip 657", "Strip 658", "Strip 659", "Strip 660", "Strip 661", "Strip 662", "Strip 663", "Strip 664", "Strip 665", "Strip 666", "Strip 667", "Strip 668", "Strip 669", "Strip 670", "Strip 671", "Strip 672", "Strip 673", "Strip 674", "Strip 675", "Strip 676", "Strip 677", "Strip 678", "Strip 679", "Strip 680", "Strip 681", "Strip 682", "Strip 683", "Strip 684", "Strip 685", "Strip 686", "Strip 687", "Strip 688", "Strip 689", "Strip 690", "Strip 691", "Strip 692", "Strip 693", "Strip 694", "Strip 695", "Strip 696", "Strip 697", "Strip 698", "Strip 699", "Strip 700", "Strip 701", "Strip 702", "Strip 703", "Strip 704", "Strip 705", "Strip 706", "Strip 707", "Strip 708", "Strip 709", "Strip 710", "Strip 711", "Strip 712", "Strip 713", "Strip 714", "Strip 715", "Strip 716", "Strip 717", "Strip 718", "Strip 719", "Strip 720", "Strip 721", "Strip 722", "Strip 723", "Strip 724", "Strip 725", "Strip 726", "Strip 727", "Strip 728", "Strip 729", "Strip 730", "Strip 731", "Strip 732", "Strip 733", "Strip 734", "Strip 735", "Strip 736", "Strip 737", "Strip 738", "Strip 739", "Strip 740", "Strip 741", "Strip 742", "Strip 743", "Strip 744", "Strip 745", "Strip 746", "Strip 747", "Strip 748", "Strip 749", "Strip 750", "Strip 751", "Strip 752", "Strip 753", "Strip 754", "Strip 755", "Strip 756", "Strip 757", "Strip 758", "Strip 759", "Strip 760", "Strip 761", "Strip 762", "Strip 763", "Strip 764", "Strip 765", "Strip 766", "Strip 767", "Strip 768", "Strip 769", "Strip 770", "Strip 771", "Strip 772", "Strip 773", "Strip 774", "Strip 775", "Strip 776", "Strip 777", "Strip 778", "Strip 779", "Strip 780", "Strip 781", "Strip 782", "Strip 783", "Strip 784", "Strip 785", "Strip 786", "Strip 787", "Strip 788", "Strip 789", "Strip 790", "Strip 791", "Strip 792", "Strip 793", "Strip 794", "Strip 795", "Strip 796", "Strip 797", "Strip 798", "Strip 799", "Strip 800", "Strip 801", "Strip 802", "Strip 803", "Strip 804", "Strip 805", "Strip 806", "Strip 807", "Strip 808", "Strip 809", "Strip 810", "Strip 811", "Strip 812", "Strip 813", "Strip 814", "Strip 815", "Strip 816", "Strip 817", "Strip 818", "Strip 819", "Strip 820", "Strip 821", "Strip 822", "Strip 823", "Strip 824", "Strip 825", "Strip 826", "Strip 827", "Strip 828", "Strip 829", "Strip 830", "Strip 831", "Strip 832", "Strip 833", "Strip 834", "Strip 835", "Strip 836", "Strip 837", "Strip 838", "Strip 839", "Strip 840", "Strip 841", "Strip 842", "Strip 843", "Strip 844", "Strip 845", "Strip 846", "Strip 847", "Strip 848", "Strip 849", "Strip 850", "Strip 851", "Strip 852", "Strip 853", "Strip 854", "Strip 855", "Strip 856", "Strip 857", "Strip 858", "Strip 859", "Strip 860", "Strip 861", "Strip 862", "Strip 863", "Strip 864", "Strip 865", "Strip 866", "Strip 867", "Strip 868", "Strip 869", "Strip 870", "Strip 871", "Strip 872", "Strip 873", "Strip 874", "Strip 875", "Strip 876", "Strip 877", "Strip 878", "Strip 879", "Strip 880", "Strip 881", "Strip 882", "Strip 883", "Strip 884", "Strip 885", "Strip 886", "Strip 887", "Strip 888", "Strip 889", "Strip 890", "Strip 891", "Strip 892", "Strip 893", "Strip 894", "Strip 895", "Strip 896", "Strip 897", "Strip 898", "Strip 899", "Strip 900", "Strip 901", "Strip 902", "Strip 903", "Strip 904", "Strip 905", "Strip 906", "Strip 907", "Strip 908", "Strip 909", "Strip 910", "Strip 911", "Strip 912", "Strip 913", "Strip 914", "Strip 915", "Strip 916", "Strip 917", "Strip 918", "Strip 919", "Strip 920", "Strip 921", "Strip 922", "Strip 923", "Strip 924", "Strip 925", "Strip 926", "Strip 927", "Strip 928", "Strip 929", "Strip 930", "Strip 931", "Strip 932", "Strip 933", "Strip 934", "Strip 935", "Strip 936", "Strip 937", "Strip 938", "Strip 939", "Strip 940", "Strip 941", "Strip 942", "Strip 943", "Strip 944", "Strip 945", "Strip 946", "Strip 947", "Strip 948", "Strip 949", "Strip 950", "Strip 951", "Strip 952", "Strip 953", "Strip 954", "Strip 955", "Strip 956", "Strip 957", "Strip 958", "Strip 959", "Strip 960", "Strip 961", "Strip 962", "Strip 963", "Strip 964", "Strip 965", "Strip 966", "Strip 967", "Strip 968", "Strip 969", "Strip 970", "Strip 971", "Strip 972", "Strip 973", "Strip 974", "Strip 975", "Strip 976", "Strip 977", "Strip 978", "Strip 979", "Strip 980", "Strip 981", "Strip 982", "Strip 983", "Strip 984", "Strip 985", "Strip 986", "Strip 987", "Strip 988", "Strip 989", "Strip 990", "Strip 991", "Strip 992", "Strip 993", "Strip 994", "Strip 995", "Strip 996", "Strip 997", "Strip 998", "Strip 999", "Strip 1000", "Strip 1001", "Strip 1002", "Strip 1003", "Strip 1004", "Strip 1005", "Strip 1006", "Strip 1007", "Strip 1008", "Strip 1009", "Strip 1010", "Strip 1011", "Strip 1012", "Strip 1013", "Strip 1014", "Strip 1015", "Strip 1016", "Strip 1017", "Strip 1018", "Strip 1019", "Strip 1020", "Strip 1021", "Strip 1022", "Strip 1023", "Strip 1024", "Strip 1025", "Strip 1026", "Strip 1027", "Strip 1028", "Strip 1029", "Strip 1030", "Strip 1031", "Strip 1032", "Strip 1033", "Strip 1034", "Strip 1035", "Strip 1036", "Strip 1037", "Strip 1038", "Strip 1039", "Strip 1040", "Strip 1041", "Strip 1042", "Strip 1043", "Strip 1044", "Strip 1045", "Strip 1046", "Strip 1047", "Strip 1048", "Strip 1049", "Strip 1050", "Strip 1051", "Strip 1052", "Strip 1053", "Strip 1054", "Strip 1055", "Strip 1056", "Strip 1057", "Strip 1058", "Strip 1059", "Strip 1060", "Strip 1061", "Strip 1062", "Strip 1063", "Strip 1064", "Strip 1065", "Strip 1066", "Strip 1067", "Strip 1068", "Strip 1069", "Strip 1070", "Strip 1071", "Strip 1072", "Strip 1073", "Strip 1074", "Strip 1075", "Strip 1076", "Strip 1077", "Strip 1078", "Strip 1079", "Strip 1080", "Strip 1081", "Strip 1082", "Strip 1083", "Strip 1084", "Strip 1085", "Strip 1086", "Strip 1087", "Strip 1088", "Strip 1089", "Strip 1090", "Strip 1091", "Strip 1092", "Strip 1093", "Strip 1094", "Strip 1095", "Strip 1096", "Strip 1097", "Strip 1098", "Strip 1099", "Strip 1100", "Strip 1101", "Strip 1102", "Strip 1103", "Strip 1104", "Strip 1105", "Strip 1106", "Strip 1107", "Strip 1108", "Strip 1109", "Strip 1110", "Strip 1111", "Strip 1112", "Strip 1113", "Strip 1114", "Strip 1115", "Strip 1116", "Strip 1117", "Strip 1118", "Strip 1119", "Strip 1120", "Strip 1121", "Strip 1122", "Strip 1123", "Strip 1124", "Strip 1125", "Strip 1126", "Strip 1127", "Strip 1128", "Strip 1129", "Strip 1130", "Strip 1131", "Strip 1132", "Strip 1133", "Strip 1134", "Strip 1135", "Strip 1136", "Strip 1137", "Strip 1138", "Strip 1139", "Strip 1140", "Strip 1141", "Strip 1142", "Strip 1143", "Strip 1144", "Strip 1145", "Strip 1146", "Strip 1147", "Strip 1148", "Strip 1149", "Strip 1150", "Strip 1151", "Strip 1152", "Strip 1153"]
  in  "To4":u16(ring) items=["Strip 0", "Strip 1", "Strip 2", "Strip 3", "Strip 4", "Strip 5", "Strip 6", "Strip 7", "Strip 8", "Strip 9", "Strip 10", "Strip 11", "Strip 12", "Strip 13", "Strip 14", "Strip 15", "Strip 16", "Strip 17", "Strip 18", "Strip 19", "Strip 20", "Strip 21", "Strip 22", "Strip 23", "Strip 24", "Strip 25", "Strip 26", "Strip 27", "Strip 28", "Strip 29", "Strip 30", "Strip 31", "Strip 32", "Strip 33", "Strip 34", "Strip 35", "Strip 36", "Strip 37", "Strip 38", "Strip 39", "Strip 40", "Strip 41", "Strip 42", "Strip 43", "Strip 44", "Strip 45", "Strip 46", "Strip 47", "Strip 48", "Strip 49", "Strip 50", "Strip 51", "Strip 52", "Strip 53", "Strip 54", "Strip 55", "Strip 56", "Strip 57", "Strip 58", "Strip 59", "Strip 60", "Strip 61", "Strip 62", "Strip 63", "Strip 64", "Strip 65", "Strip 66", "Strip 67", "Strip 68", "Strip 69", "Strip 70", "Strip 71", "Strip 72", "Strip 73", "Strip 74", "Strip 75", "Strip 76", "Strip 77", "Strip 78", "Strip 79", "Strip 80", "Strip 81", "Strip 82", "Strip 83", "Strip 84", "Strip 85", "Strip 86", "Strip 87", "Strip 88", "Strip 89", "Strip 90", "Strip 91", "Strip 92", "Strip 93", "Strip 94", "Strip 95", "Strip 96", "Strip 97", "Strip 98", "Strip 99", "Strip 100", "Strip 101", "Strip 102", "Strip 103", "Strip 104", "Strip 105", "Strip 106", "Strip 107", "Strip 108", "Strip 109", "Strip 110", "Strip 111", "Strip 112", "Strip 113", "Strip 114", "Strip 115", "Strip 116", "Strip 117", "Strip 118", "Strip 119", "Strip 120", "Strip 121", "Strip 122", "Strip 123", "Strip 124", "Strip 125", "Strip 126", "Strip 127", "Strip 128", "Strip 129", "Strip 130", "Strip 131", "Strip 132", "Strip 133", "Strip 134", "Strip 135", "Strip 136", "Strip 137", "Strip 138", "Strip 139", "Strip 140", "Strip 141", "Strip 142", "Strip 143", "Strip 144", "Strip 145", "Strip 146", "Strip 147", "Strip 148", "Strip 149", "Strip 150", "Strip 151", "Strip 152", "Strip 153", "Strip 154", "Strip 155", "Strip 156", "Strip 157", "Strip 158", "Strip 159", "Strip 160", "Strip 161", "Strip 162", "Strip 163", "Strip 164", "Strip 165", "Strip 166", "Strip 167", "Strip 168", "Strip 169", "Strip 170", "Strip 171", "Strip 172", "Strip 173", "Strip 174", "Strip 175", "Strip 176", "Strip 177", "Strip 178", "Strip 179", "Strip 180", "Strip 181", "Strip 182", "Strip 183", "Strip 184", "Strip 185", "Strip 186", "Strip 187", "Strip 188", "Strip 189", "Strip 190", "Strip 191", "Strip 192", "Strip 193", "Strip 194", "Strip 195", "Strip 196", "Strip 197", "Strip 198", "Strip 199", "Strip 200", "Strip 201", "Strip 202", "Strip 203", "Strip 204", "Strip 205", "Strip 206", "Strip 207", "Strip 208", "Strip 209", "Strip 210", "Strip 211", "Strip 212", "Strip 213", "Strip 214", "Strip 215", "Strip 216", "Strip 217", "Strip 218", "Strip 219", "Strip 220", "Strip 221", "Strip 222", "Strip 223", "Strip 224", "Strip 225", "Strip 226", "Strip 227", "Strip 228", "Strip 229", "Strip 230", "Strip 231", "Strip 232", "Strip 233", "Strip 234", "Strip 235", "Strip 236", "Strip 237", "Strip 238", "Strip 239", "Strip 240", "Strip 241", "Strip 242", "Strip 243", "Strip 244", "Strip 245", "Strip 246", "Strip 247", "Strip 248", "Strip 249", "Strip 250", "Strip 251", "Strip 252", "Strip 253", "Strip 254", "Strip 255", "Strip 256", "Strip 257", "Strip 258", "Strip 259", "Strip 260", "Strip 261", "Strip 262", "Strip 263", "Strip 264", "Strip 265", "Strip 266", "Strip 267", "Strip 268", "Strip 269", "Strip 270", "Strip 271", "Strip 272", "Strip 273", "Strip 274", "Strip 275", "Strip 276", "Strip 277", "Strip 278", "Strip 279", "Strip 280", "Strip 281", "Strip 282", "Strip 283", "Strip 284", "Strip 285", "Strip 286", "Strip 287", "Strip 288", "Strip 289", "Strip 290", "Strip 291", "Strip 292", "Strip 293", "Strip 294", "Strip 295", "Strip 296", "Strip 297", "Strip 298", "Strip 299", "Strip 300", "Strip 301", "Strip 302", "Strip 303", "Strip 304", "Strip 305", "Strip 306", "Strip 307", "Strip 308", "Strip 309", "Strip 310", "Strip 311", "Strip 312", "Strip 313", "Strip 314", "Strip 315", "Strip 316", "Strip 317", "Strip 318", "Strip 319", "Strip 320", "Strip 321", "Strip 322", "Strip 323", "Strip 324", "Strip 325", "Strip 326", "Strip 327", "Strip 328", "Strip 329", "Strip 330", "Strip 331", "Strip 332", "Strip 333", "Strip 334", "Strip 335", "Strip 336", "Strip 337", "Strip 338", "Strip 339", "Strip 340", "Strip 341", "Strip 342", "Strip 343", "Strip 344", "Strip 345", "Strip 346", "Strip 347", "Strip 348", "Strip 349", "Strip 350", "Strip 351", "Strip 352", "Strip 353", "Strip 354", "Strip 355", "Strip 356", "Strip 357", "Strip 358", "Strip 359", "Strip 360", "Strip 361", "Strip 362", "Strip 363", "Strip 364", "Strip 365", "Strip 366", "Strip 367", "Strip 368", "Strip 369", "Strip 370", "Strip 371", "Strip 372", "Strip 373", "Strip 374", "Strip 375", "Strip 376", "Strip 377", "Strip 378", "Strip 379", "Strip 380", "Strip 381", "Strip 382", "Strip 383", "Strip 384", "Strip 385", "Strip 386", "Strip 387", "Strip 388", "Strip 389", "Strip 390", "Strip 391", "Strip 392", "Strip 393", "Strip 394", "Strip 395", "Strip 396", "Strip 397", "Strip 398", "Strip 399", "Strip 400", "Strip 401", "Strip 402", "Strip 403", "Strip 404", "Strip 405", "Strip 406", "Strip 407", "Strip 408", "Strip 409", "Strip 410", "Strip 411", "Strip 412", "Strip 413", "Strip 414", "Strip 415", "Strip 416", "Strip 417", "Strip 418", "Strip 419", "Strip 420", "Strip 421", "Strip 422", "Strip 423", "Strip 424", "Strip 425", "Strip 426", "Strip 427", "Strip 428", "Strip 429", "Strip 430", "Strip 431", "Strip 432", "Strip 433", "Strip 434", "Strip 435", "Strip 436", "Strip 437", "Strip 438", "Strip 439", "Strip 440", "Strip 441", "Strip 442", "Strip 443", "Strip 444", "Strip 445", "Strip 446", "Strip 447", "Strip 448", "Strip 449", "Strip 450", "Strip 451", "Strip 452", "Strip 453", "Strip 454", "Strip 455", "Strip 456", "Strip 457", "Strip 458", "Strip 459", "Strip 460", "Strip 461", "Strip 462", "Strip 463", "Strip 464", "Strip 465", "Strip 466", "Strip 467", "Strip 468", "Strip 469", "Strip 470", "Strip 471", "Strip 472", "Strip 473", "Strip 474", "Strip 475", "Strip 476", "Strip 477", "Strip 478", "Strip 479", "Strip 480", "Strip 481", "Strip 482", "Strip 483", "Strip 484", "Strip 485", "Strip 486", "Strip 487", "Strip 488", "Strip 489", "Strip 490", "Strip 491", "Strip 492", "Strip 493", "Strip 494", "Strip 495", "Strip 496", "Strip 497", "Strip 498", "Strip 499", "Strip 500", "Strip 501", "Strip 502", "Strip 503", "Strip 504", "Strip 505", "Strip 506", "Strip 507", "Strip 508", "Strip 509", "Strip 510", "Strip 511", "Strip 512", "Strip 513", "Strip 514", "Strip 515", "Strip 516", "Strip 517", "Strip 518", "Strip 519", "Strip 520", "Strip 521", "Strip 522", "Strip 523", "Strip 524", "Strip 525", "Strip 526", "Strip 527", "Strip 528", "Strip 529", "Strip 530", "Strip 531", "Strip 532", "Strip 533", "Strip 534", "Strip 535", "Strip 536", "Strip 537", "Strip 538", "Strip 539", "Strip 540", "Strip 541", "Strip 542", "Strip 543", "Strip 544", "Strip 545", "Strip 546", "Strip 547", "Strip 548", "Strip 549", "Strip 550", "Strip 551", "Strip 552", "Strip 553", "Strip 554", "Strip 555", "Strip 556", "Strip 557", "Strip 558", "Strip 559", "Strip 560", "Strip 561", "Strip 562", "Strip 563", "Strip 564", "Strip 565", "Strip 566", "Strip 567", "Strip 568", "Strip 569", "Strip 570", "Strip 571", "Strip 572", "Strip 573", "Strip 574", "Strip 575", "Strip 576", "Strip 577", "Strip 578", "Strip 579", "Strip 580", "Strip 581", "Strip 582", "Strip 583", "Strip 584", "Strip 585", "Strip 586", "Strip 587", "Strip 588", "Strip 589", "Strip 590", "Strip 591", "Strip 592", "Strip 593", "Strip 594", "Strip 595", "Strip 596", "Strip 597", "Strip 598", "Strip 599", "Strip 600", "Strip 601", "Strip 602", "Strip 603", "Strip 604", "Strip 605", "Strip 606", "Strip 607", "Strip 608", "Strip 609", "Strip 610", "Strip 611", "Strip 612", "Strip 613", "Strip 614", "Strip 615", "Strip 616", "Strip 617", "Strip 618", "Strip 619", "Strip 620", "Strip 621", "Strip 622", "Strip 623", "Strip 624", "Strip 625", "Strip 626", "Strip 627", "Strip 628", "Strip 629", "Strip 630", "Strip 631", "Strip 632", "Strip 633", "Strip 634", "Strip 635", "Strip 636", "Strip 637", "Strip 638", "Strip 639", "Strip 640", "Strip 641", "Strip 642", "Strip 643", "Strip 644", "Strip 645", "Strip 646", "Strip 647", "Strip 648", "Strip 649", "Strip 650", "Strip 651", "Strip 652", "Strip 653", "Strip 654", "Strip 655", "Strip 656", "Strip 657", "Strip 658", "Strip 659", "Strip 660", "Strip 661", "Strip 662", "Strip 663", "Strip 664", "Strip 665", "Strip 666", "Strip 667", "Strip 668", "Strip 669", "Strip 670", "Strip 671", "Strip 672", "Strip 673", "Strip 674", "Strip 675", "Strip 676", "Strip 677", "Strip 678", "Strip 679", "Strip 680", "Strip 681", "Strip 682", "Strip 683", "Strip 684", "Strip 685", "Strip 686", "Strip 687", "Strip 688", "Strip 689", "Strip 690", "Strip 691", "Strip 692", "Strip 693", "Strip 694", "Strip 695", "Strip 696", "Strip 697", "Strip 698", "Strip 699", "Strip 700", "Strip 701", "Strip 702", "Strip 703", "Strip 704", "Strip 705", "Strip 706", "Strip 707", "Strip 708", "Strip 709", "Strip 710", "Strip 711", "Strip 712", "Strip 713", "Strip 714", "Strip 715", "Strip 716", "Strip 717", "Strip 718", "Strip 719", "Strip 720", "Strip 721", "Strip 722", "Strip 723", "Strip 724", "Strip 725", "Strip 726", "Strip 727", "Strip 728", "Strip 729", "Strip 730", "Strip 731", "Strip 732", "Strip 733", "Strip 734", "Strip 735", "Strip 736", "Strip 737", "Strip 738", "Strip 739", "Strip 740", "Strip 741", "Strip 742", "Strip 743", "Strip 744", "Strip 745", "Strip 746", "Strip 747", "Strip 748", "Strip 749", "Strip 750", "Strip 751", "Strip 752", "Strip 753", "Strip 754", "Strip 755", "Strip 756", "Strip 757", "Strip 758", "Strip 759", "Strip 760", "Strip 761", "Strip 762", "Strip 763", "Strip 764", "Strip 765", "Strip 766", "Strip 767", "Strip 768", "Strip 769", "Strip 770", "Strip 771", "Strip 772", "Strip 773", "Strip 774", "Strip 775", "Strip 776", "Strip 777", "Strip 778", "Strip 779", "Strip 780", "Strip 781", "Strip 782", "Strip 783", "Strip 784", "Strip 785", "Strip 786", "Strip 787", "Strip 788", "Strip 789", "Strip 790", "Strip 791", "Strip 792", "Strip 793", "Strip 794", "Strip 795", "Strip 796", "Strip 797", "Strip 798", "Strip 799", "Strip 800", "Strip 801", "Strip 802", "Strip 803", "Strip 804", "Strip 805", "Strip 806", "Strip 807", "Strip 808", "Strip 809", "Strip 810", "Strip 811", "Strip 812", "Strip 813", "Strip 814", "Strip 815", "Strip 816", "Strip 817", "Strip 818", "Strip 819", "Strip 820", "Strip 821", "Strip 822", "Strip 823", "Strip 824", "Strip 825", "Strip 826", "Strip 827", "Strip 828", "Strip 829", "Strip 830", "Strip 831", "Strip 832", "Strip 833", "Strip 834", "Strip 835", "Strip 836", "Strip 837", "Strip 838", "Strip 839", "Strip 840", "Strip 841", "Strip 842", "Strip 843", "Strip 844", "Strip 845", "Strip 846", "Strip 847", "Strip 848", "Strip 849", "Strip 850", "Strip 851", "Strip 852", "Strip 853", "Strip 854", "Strip 855", "Strip 856", "Strip 857", "Strip 858", "Strip 859", "Strip 860", "Strip 861", "Strip 862", "Strip 863", "Strip 864", "Strip 865", "Strip 866", "Strip 867", "Strip 868", "Strip 869", "Strip 870", "Strip 871", "Strip 872", "Strip 873", "Strip 874", "Strip 875", "Strip 876", "Strip 877", "Strip 878", "Strip 879", "Strip 880", "Strip 881", "Strip 882", "Strip 883", "Strip 884", "Strip 885", "Strip 886", "Strip 887", "Strip 888", "Strip 889", "Strip 890", "Strip 891", "Strip 892", "Strip 893", "Strip 894", "Strip 895", "Strip 896", "Strip 897", "Strip 898", "Strip 899", "Strip 900", "Strip 901", "Strip 902", "Strip 903", "Strip 904", "Strip 905", "Strip 906", "Strip 907", "Strip 908", "Strip 909", "Strip 910", "Strip 911", "Strip 912", "Strip 913", "Strip 914", "Strip 915", "Strip 916", "Strip 917", "Strip 918", "Strip 919", "Strip 920", "Strip 921", "Strip 922", "Strip 923", "Strip 924", "Strip 925", "Strip 926", "Strip 927", "Strip 928", "Strip 929", "Strip 930", "Strip 931", "Strip 932", "Strip 933", "Strip 934", "Strip 935", "Strip 936", "Strip 937", "Strip 938", "Strip 939", "Strip 940", "Strip 941", "Strip 942", "Strip 943", "Strip 944", "Strip 945", "Strip 946", "Strip 947", "Strip 948", "Strip 949", "Strip 950", "Strip 951", "Strip 952", "Strip 953", "Strip 954", "Strip 955", "Strip 956", "Strip 957", "Strip 958", "Strip 959", "Strip 960", "Strip 961", "Strip 962", "Strip 963", "Strip 964", "Strip 965", "Strip 966", "Strip 967", "Strip 968", "Strip 969", "Strip 970", "Strip 971", "Strip 972", "Strip 973", "Strip 974", "Strip 975", "Strip 976", "Strip 977", "Strip 978", "Strip 979", "Strip 980", "Strip 981", "Strip 982", "Strip 983", "Strip 984", "Strip 985", "Strip 986", "Strip 987", "Strip 988", "Strip 989", "Strip 990", "Strip 991", "Strip 992", "Strip 993", "Strip 994", "Strip 995", "Strip 996", "Strip 997", "Strip 998", "Strip 999", "Strip 1000", "Strip 1001", "Strip 1002", "Strip 1003", "Strip 1004", "Strip 1005", "Strip 1006", "Strip 1007", "Strip 1008", "Strip 1009", "Strip 1010", "Strip 1011", "Strip 1012", "Strip 1013", "Strip 1014", "Strip 1015", "Strip 1016", "Strip 1017", "Strip 1018", "Strip 1019", "Strip 1020", "Strip 1021", "Strip 1022", "Strip 1023", "Strip 1024", "Strip 1025", "Strip 1026", "Strip 1027", "Strip 1028", "Strip 1029", "Strip 1030", "Strip 1031", "Strip 1032", "Strip 1033", "Strip 1034", "Strip 1035", "Strip 1036", "Strip 1037", "Strip 1038", "Strip 1039", "Strip 1040", "Strip 1041", "Strip 1042", "Strip 1043", "Strip 1044", "Strip 1045", "Strip 1046", "Strip 1047", "Strip 1048", "Strip 1049", "Strip 1050", "Strip 1051", "Strip 1052", "Strip 1053", "Strip 1054", "Strip 1055", "Strip 1056", "Strip 1057", "Strip 1058", "Strip 1059", "Strip 1060", "Strip 1061", "Strip 1062", "Strip 1063", "Strip 1064", "Strip 1065", "Strip 1066", "Strip 1067", "Strip 1068", "Strip 1069", "Strip 1070", "Strip 1071", "Strip 1072", "Strip 1073", "Strip 1074", "Strip 1075", "Strip 1076", "Strip 1077", "Strip 1078", "Strip 1079", "Strip 1080", "Strip 1081", "Strip 1082", "Strip 1083", "Strip 1084", "Strip 1085", "Strip 1086", "Strip 1087", "Strip 1088", "Strip 1089", "Strip 1090", "Strip 1091", "Strip 1092", "Strip 1093", "Strip 1094", "Strip 1095", "Strip 1096", "Strip 1097", "Strip 1098", "Strip 1099", "Strip 1100", "Strip 1101", "Strip 1102", "Strip 1103", "Strip 1104", "Strip 1105", "Strip 1106", "Strip 1107", "Strip 1108", "Strip 1109", "Strip 1110", "Strip 1111", "Strip 1112", "Strip 1113", "Strip 1114", "Strip 1115", "Strip 1116", "Strip 1117", "Strip 1118", "Strip 1119", "Strip 1120", "Strip 1121", "Strip 1122", "Strip 1123", "Strip 1124", "Strip 1125", "Strip 1126", "Strip 1127", "Strip 1128", "Strip 1129", "Strip 1130", "Strip 1131", "Strip 1132", "Strip 1133", "Strip 1134", "Strip 1135", "Strip 1136", "Strip 1137", "Strip 1138", "Strip 1139", "Strip 1140", "Strip 1141", "Strip 1142", "Strip 1143", "Strip 1144", "Strip 1145", "Strip 1146", "Strip 1147", "Strip 1148", "Strip 1149", "Strip 1150", "Strip 1151", "Strip 1152", "Strip 1153", "Strip 1154", "Strip 1155", "Strip 1156", "Strip 1157", "Strip 1158", "Strip 1159", "Strip 1160", "Strip 1161", "Strip 1162", "Strip 1163", "Strip 1164", "Strip 1165", "Strip 1166", "Strip 1167", "Strip 1168", "Strip 1169", "Strip 1170", "Strip 1171", "Strip 1172", "Strip 1173", "Strip 1174", "Strip 1175", "Strip 1176", "Strip 1177", "Strip 1178", "Strip 1179", "Strip 1180", "Strip 1181", "Strip 1182", "Strip 1183", "Strip 1184", "Strip 1185", "Strip 1186", "Strip 1187", "Strip 1188", "Strip 1189", "Strip 1190", "Strip 1191", "Strip 1192", "Strip 1193", "Strip 1194", "Strip 1195", "Strip 1196", "Strip 1197", "Strip 1198", "Strip 1199", "Strip 1200", "Strip 1201", "Strip 1202", "Strip 1203", "Strip 1204", "Strip 1205", "Strip 1206", "Strip 1207", "Strip 1208", "Strip 1209", "Strip 1210", "Strip 1211", "Strip 1212", "Strip 1213", "Strip 1214", "Strip 1215", "Strip 1216", "Strip 1217", "Strip 1218", "Strip 1219", "Strip 1220", "Strip 1221", "Strip 1222", "Strip 1223", "Strip 1224", "Strip 1225", "Strip 1226", "Strip 1227", "Strip 1228", "Strip 1229", "Strip 1230", "Strip 1231", "Strip 1232", "Strip 1233", "Strip 1234", "Strip 1235", "Strip 1236", "Strip 1237", "Strip 1238", "Strip 1239", "Strip 1240", "Strip 1241", "Strip 1242", "Strip 1243", "Strip 1244", "Strip 1245", "Strip 1246", "Strip 1247", "Strip 1248", "Strip 1249", "Strip 1250", "Strip 1251", "Strip 1252", "Strip 1253", "Strip 1254", "Strip 1255", "Strip 1256", "Strip 1257", "Strip 1258", "Strip 1259", "Strip 1260", "Strip 1261", "Strip 1262", "Strip 1263", "Strip 1264", "Strip 1265", "Strip 1266", "Strip 1267", "Strip 1268", "Strip 1269", "Strip 1270", "Strip 1271", "Strip 1272", "Strip 1273", "Strip 1274", "Strip 1275", "Strip 1276", "Strip 1277", "Strip 1278", "Strip 1279", "Strip 1280", "Strip 1281", "Strip 1282", "Strip 1283", "Strip 1284", "Strip 1285", "Strip 1286", "Strip 1287", "Strip 1288", "Strip 1289", "Strip 1290", "Strip 1291", "Strip 1292", "Strip 1293", "Strip 1294", "Strip 1295", "Strip 1296", "Strip 1297", "Strip 1298", "Strip 1299", "Strip 1300", "Strip 1301", "Strip 1302", "Strip 1303", "Strip 1304", "Strip 1305", "Strip 1306", "Strip 1307", "Strip 1308", "Strip 1309", "Strip 1310", "Strip 1311", "Strip 1312", "Strip 1313", "Strip 1314", "Strip 1315", "Strip 1316", "Strip 1317", "Strip 1318", "Strip 1319", "Strip 1320", "Strip 1321", "Strip 1322", "Strip 1323", "Strip 1324", "Strip 1325", "Strip 1326", "Strip 1327", "Strip 1328", "Strip 1329", "Strip 1330", "Strip 1331", "Strip 1332", "Strip 1333", "Strip 1334", "Strip 1335", "Strip 1336", "Strip 1337", "Strip 1338", "Strip 1339", "Strip 1340", "Strip 1341", "Strip 1342", "Strip 1343", "Strip 1344", "Strip 1345", "Strip 1346", "Strip 1347", "Strip 1348", "Strip 1349", "Strip 1350", "Strip 1351", "Strip 1352", "Strip 1353", "Strip 1354", "Strip 1355", "Strip 1356", "Strip 1357", "Strip 1358", "Strip 1359", "Strip 1360", "Strip 1361", "Strip 1362", "Strip 1363", "Strip 1364", "Strip 1365", "Strip 1366", "Strip 1367", "Strip 1368", "Strip 1369", "Strip 1370", "Strip 1371", "Strip 1372", "Strip 1373", "Strip 1374", "Strip 1375", "Strip 1376", "Strip 1377", "Strip 1378", "Strip 1379", "Strip 1380", "Strip 1381", "Strip 1382", "Strip 1383", "Strip 1384", "Strip 1385", "Strip 1386", "Strip 1387", "Strip 1388", "Strip 1389", "Strip 1390", "Strip 1391", "Strip 1392", "Strip 1393", "Strip 1394", "Strip 1395", "Strip 1396", "Strip 1397", "Strip 1398", "Strip 1399", "Strip 1400", "Strip 1401", "Strip 1402", "Strip 1403", "Strip 1404", "Strip 1405", "Strip 1406", "Strip 1407", "Strip 1408", "Strip 1409"]
  in  "To3":u16(ring) items=["Strip 0", "Strip 1", "Strip 2", "Strip 3", "Strip 4", "Strip 5", "Strip 6", "Strip 7", "Strip 8", "Strip 9", "Strip 10", "Strip 11", "Strip 12", "Strip 13", "Strip 14", "Strip 15", "Strip 16", "Strip 17", "Strip 18", "Strip 19", "Strip 20", "Strip 21", "Strip 22", "Strip 23", "Strip 24", "Strip 25", "Strip 26", "Strip 27", "Strip 28", "Strip 29", "Strip 30", "Strip 31", "Strip 32", "Strip 33", "Strip 34", "Strip 35", "Strip 36", "Strip 37", "Strip 38", "Strip 39", "Strip 40", "Strip 41", "Strip 42", "Strip 43", "Strip 44", "Strip 45", "Strip 46", "Strip 47", "Strip 48", "Strip 49", "Strip 50", "Strip 51", "Strip 52", "Strip 53", "Strip 54", "Strip 55", "Strip 56", "Strip 57", "Strip 58", "Strip 59", "Strip 60", "Strip 61", "Strip 62", "Strip 63", "Strip 64", "Strip 65", "Strip 66", "Strip 67", "Strip 68", "Strip 69", "Strip 70", "Strip 71", "Strip 72", "Strip 73", "Strip 74", "Strip 75", "Strip 76", "Strip 77", "Strip 78", "Strip 79", "Strip 80", "Strip 81", "Strip 82", "Strip 83", "Strip 84", "Strip 85", "Strip 86", "Strip 87", "Strip 88", "Strip 89", "Strip 90", "Strip 91", "Strip 92", "Strip 93", "Strip 94", "Strip 95", "Strip 96", "Strip 97", "Strip 98", "Strip 99", "Strip 100", "Strip 101", "Strip 102", "Strip 103", "Strip 104", "Strip 105", "Strip 106", "Strip 107", "Strip 108", "Strip 109", "Strip 110", "Strip 111", "Strip 112", "Strip 113", "Strip 114", "Strip 115", "Strip 116", "Strip 117", "Strip 118", "Strip 119", "Strip 120", "Strip 121", "Strip 122", "Strip 123", "Strip 124", "Strip 125", "Strip 126", "Strip 127", "Strip 128", "Strip 129", "Strip 130", "Strip 131", "Strip 132", "Strip 133", "Strip 134", "Strip 135", "Strip 136", "Strip 137", "Strip 138", "Strip 139", "Strip 140", "Strip 141", "Strip 142", "Strip 143", "Strip 144", "Strip 145", "Strip 146", "Strip 147", "Strip 148", "Strip 149", "Strip 150", "Strip 151", "Strip 152", "Strip 153", "Strip 154", "Strip 155", "Strip 156", "Strip 157", "Strip 158", "Strip 159", "Strip 160", "Strip 161", "Strip 162", "Strip 163", "Strip 164", "Strip 165", "Strip 166", "Strip 167", "Strip 168", "Strip 169", "Strip 170", "Strip 171", "Strip 172", "Strip 173", "Strip 174", "Strip 175", "Strip 176", "Strip 177", "Strip 178", "Strip 179", "Strip 180", "Strip 181", "Strip 182", "Strip 183", "Strip 184", "Strip 185", "Strip 186", "Strip 187", "Strip 188", "Strip 189", "Strip 190", "Strip 191", "Strip 192", "Strip 193", "Strip 194", "Strip 195", "Strip 196", "Strip 197", "Strip 198", "Strip 199", "Strip 200", "Strip 201", "Strip 202", "Strip 203", "Strip 204", "Strip 205", "Strip 206", "Strip 207", "Strip 208", "Strip 209", "Strip 210", "Strip 211", "Strip 212", "Strip 213", "Strip 214", "Strip 215", "Strip 216", "Strip 217", "Strip 218", "Strip 219", "Strip 220", "Strip 221", "Strip 222", "Strip 223", "Strip 224", "Strip 225", "Strip 226", "Strip 227", "Strip 228", "Strip 229", "Strip 230", "Strip 231", "Strip 232", "Strip 233", "Strip 234", "Strip 235", "Strip 236", "Strip 237", "Strip 238", "Strip 239", "Strip 240", "Strip 241", "Strip 242", "Strip 243", "Strip 244", "Strip 245", "Strip 246", "Strip 247", "Strip 248", "Strip 249", "Strip 250", "Strip 251", "Strip 252", "Strip 253", "Strip 254", "Strip 255", "Strip 256", "Strip 257", "Strip 258", "Strip 259", "Strip 260", "Strip 261", "Strip 262", "Strip 263", "Strip 264", "Strip 265", "Strip 266", "Strip 267", "Strip 268", "Strip 269", "Strip 270", "Strip 271", "Strip 272", "Strip 273", "Strip 274", "Strip 275", "Strip 276", "Strip 277", "Strip 278", "Strip 279", "Strip 280", "Strip 281", "Strip 282", "Strip 283", "Strip 284", "Strip 285", "Strip 286", "Strip 287", "Strip 288", "Strip 289", "Strip 290", "Strip 291", "Strip 292", "Strip 293", "Strip 294", "Strip 295", "Strip 296", "Strip 297", "Strip 298", "Strip 299", "Strip 300", "Strip 301", "Strip 302", "Strip 303", "Strip 304", "Strip 305", "Strip 306", "Strip 307", "Strip 308", "Strip 309", "Strip 310", "Strip 311", "Strip 312", "Strip 313", "Strip 314", "Strip 315", "Strip 316", "Strip 317", "Strip 318", "Strip 319", "Strip 320", "Strip 321", "Strip 322", "Strip 323", "Strip 324", "Strip 325", "Strip 326", "Strip 327", "Strip 328", "Strip 329", "Strip 330", "Strip 331", "Strip 332", "Strip 333", "Strip 334", "Strip 335", "Strip 336", "Strip 337", "Strip 338", "Strip 339", "Strip 340", "Strip 341", "Strip 342", "Strip 343", "Strip 344", "Strip 345", "Strip 346", "Strip 347", "Strip 348", "Strip 349", "Strip 350", "Strip 351", "Strip 352", "Strip 353", "Strip 354", "Strip 355", "Strip 356", "Strip 357", "Strip 358", "Strip 359", "Strip 360", "Strip 361", "Strip 362", "Strip 363", "Strip 364", "Strip 365", "Strip 366", "Strip 367", "Strip 368", "Strip 369", "Strip 370", "Strip 371", "Strip 372", "Strip 373", "Strip 374", "Strip 375", "Strip 376", "Strip 377", "Strip 378", "Strip 379", "Strip 380", "Strip 381", "Strip 382", "Strip 383", "Strip 384", "Strip 385", "Strip 386", "Strip 387", "Strip 388", "Strip 389", "Strip 390", "Strip 391", "Strip 392", "Strip 393", "Strip 394", "Strip 395", "Strip 396", "Strip 397", "Strip 398", "Strip 399", "Strip 400", "Strip 401", "Strip 402", "Strip 403", "Strip 404", "Strip 405", "Strip 406", "Strip 407", "Strip 408", "Strip 409", "Strip 410", "Strip 411", "Strip 412", "Strip 413", "Strip 414", "Strip 415", "Strip 416", "Strip 417", "Strip 418", "Strip 419", "Strip 420", "Strip 421", "Strip 422", "Strip 423", "Strip 424", "Strip 425", "Strip 426", "Strip 427", "Strip 428", "Strip 429", "Strip 430", "Strip 431", "Strip 432", "Strip 433", "Strip 434", "Strip 435", "Strip 436", "Strip 437", "Strip 438", "Strip 439", "Strip 440", "Strip 441", "Strip 442", "Strip 443", "Strip 444", "Strip 445", "Strip 446", "Strip 447", "Strip 448", "Strip 449", "Strip 450", "Strip 451", "Strip 452", "Strip 453", "Strip 454", "Strip 455", "Strip 456", "Strip 457", "Strip 458", "Strip 459", "Strip 460", "Strip 461", "Strip 462", "Strip 463", "Strip 464", "Strip 465", "Strip 466", "Strip 467", "Strip 468", "Strip 469", "Strip 470", "Strip 471", "Strip 472", "Strip 473", "Strip 474", "Strip 475", "Strip 476", "Strip 477", "Strip 478", "Strip 479", "Strip 480", "Strip 481", "Strip 482", "Strip 483", "Strip 484", "Strip 485", "Strip 486", "Strip 487", "Strip 488", "Strip 489", "Strip 490", "Strip 491", "Strip 492", "Strip 493", "Strip 494", "Strip 495", "Strip 496", "Strip 497", "Strip 498", "Strip 499", "Strip 500", "Strip 501", "Strip 502", "Strip 503", "Strip 504", "Strip 505", "Strip 506", "Strip 507", "Strip 508", "Strip 509", "Strip 510", "Strip 511", "Strip 512", "Strip 513", "Strip 514", "Strip 515", "Strip 516", "Strip 517", "Strip 518", "Strip 519", "Strip 520", "Strip 521", "Strip 522", "Strip 523", "Strip 524", "Strip 525", "Strip 526", "Strip 527", "Strip 528", "Strip 529", "Strip 530", "Strip 531", "Strip 532", "Strip 533", "Strip 534", "Strip 535", "Strip 536", "Strip 537", "Strip 538", "Strip 539", "Strip 540", "Strip 541", "Strip 542", "Strip 543", "Strip 544", "Strip 545", "Strip 546", "Strip 547", "Strip 548", "Strip 549", "Strip 550", "Strip 551", "Strip 552", "Strip 553", "Strip 554", "Strip 555", "Strip 556", "Strip 557", "Strip 558", "Strip 559", "Strip 560", "Strip 561", "Strip 562", "Strip 563", "Strip 564", "Strip 565", "Strip 566", "Strip 567", "Strip 568", "Strip 569", "Strip 570", "Strip 571", "Strip 572", "Strip 573", "Strip 574", "Strip 575", "Strip 576", "Strip 577", "Strip 578", "Strip 579", "Strip 580", "Strip 581", "Strip 582", "Strip 583", "Strip 584", "Strip 585", "Strip 586", "Strip 587", "Strip 588", "Strip 589", "Strip 590", "Strip 591", "Strip 592", "Strip 593", "Strip 594", "Strip 595", "Strip 596", "Strip 597", "Strip 598", "Strip 599", "Strip 600", "Strip 601", "Strip 602", "Strip 603", "Strip 604", "Strip 605", "Strip 606", "Strip 607", "Strip 608", "Strip 609", "Strip 610", "Strip 611", "Strip 612", "Strip 613", "Strip 614", "Strip 615", "Strip 616", "Strip 617", "Strip 618", "Strip 619", "Strip 620", "Strip 621", "Strip 622", "Strip 623", "Strip 624", "Strip 625", "Strip 626", "Strip 627", "Strip 628", "Strip 629", "Strip 630", "Strip 631", "Strip 632", "Strip 633", "Strip 634", "Strip 635", "Strip 636", "Strip 637", "Strip 638", "Strip 639", "Strip 640", "Strip 641", "Strip 642", "Strip 643", "Strip 644", "Strip 645", "Strip 646", "Strip 647", "Strip 648", "Strip 649", "Strip 650", "Strip 651", "Strip 652", "Strip 653", "Strip 654", "Strip 655", "Strip 656", "Strip 657", "Strip 658", "Strip 659", "Strip 660", "Strip 661", "Strip 662", "Strip 663", "Strip 664", "Strip 665", "Strip 666", "Strip 667", "Strip 668", "Strip 669", "Strip 670", "Strip 671", "Strip 672", "Strip 673", "Strip 674", "Strip 675", "Strip 676", "Strip 677", "Strip 678", "Strip 679", "Strip 680", "Strip 681", "Strip 682", "Strip 683", "Strip 684", "Strip 685", "Strip 686", "Strip 687", "Strip 688", "Strip 689", "Strip 690", "Strip 691", "Strip 692", "Strip 693", "Strip 694", "Strip 695", "Strip 696", "Strip 697", "Strip 698", "Strip 699", "Strip 700", "Strip 701", "Strip 702", "Strip 703", "Strip 704", "Strip 705", "Strip 706", "Strip 707", "Strip 708", "Strip 709", "Strip 710", "Strip 711", "Strip 712", "Strip 713", "Strip 714", "Strip 715", "Strip 716", "Strip 717", "Strip 718", "Strip 719", "Strip 720", "Strip 721", "Strip 722", "Strip 723", "Strip 724", "Strip 725", "Strip 726", "Strip 727", "Strip 728", "Strip 729", "Strip 730", "Strip 731", "Strip 732", "Strip 733", "Strip 734", "Strip 735", "Strip 736", "Strip 737", "Strip 738", "Strip 739", "Strip 740", "Strip 741", "Strip 742", "Strip 743", "Strip 744", "Strip 745", "Strip 746", "Strip 747", "Strip 748", "Strip 749", "Strip 750", "Strip 751", "Strip 752", "Strip 753", "Strip 754", "Strip 755", "Strip 756", "Strip 757", "Strip 758", "Strip 759", "Strip 760", "Strip 761", "Strip 762", "Strip 763", "Strip 764", "Strip 765", "Strip 766", "Strip 767", "Strip 768", "Strip 769", "Strip 770", "Strip 771", "Strip 772", "Strip 773", "Strip 774", "Strip 775", "Strip 776", "Strip 777", "Strip 778", "Strip 779", "Strip 780", "Strip 781", "Strip 782", "Strip 783", "Strip 784", "Strip 785", "Strip 786", "Strip 787", "Strip 788", "Strip 789", "Strip 790", "Strip 791", "Strip 792", "Strip 793", "Strip 794", "Strip 795", "Strip 796", "Strip 797", "Strip 798", "Strip 799", "Strip 800", "Strip 801", "Strip 802", "Strip 803", "Strip 804", "Strip 805", "Strip 806", "Strip 807", "Strip 808", "Strip 809", "Strip 810", "Strip 811", "Strip 812", "Strip 813", "Strip 814", "Strip 815", "Strip 816", "Strip 817", "Strip 818", "Strip 819", "Strip 820", "Strip 821", "Strip 822", "Strip 823", "Strip 824", "Strip 825", "Strip 826", "Strip 827", "Strip 828", "Strip 829", "Strip 830", "Strip 831", "Strip 832", "Strip 833", "Strip 834", "Strip 835", "Strip 836", "Strip 837", "Strip 838", "Strip 839", "Strip 840", "Strip 841", "Strip 842", "Strip 843", "Strip 844", "Strip 845", "Strip 846", "Strip 847", "Strip 848", "Strip 849", "Strip 850", "Strip 851", "Strip 852", "Strip 853", "Strip 854", "Strip 855", "Strip 856", "Strip 857", "Strip 858", "Strip 859", "Strip 860", "Strip 861", "Strip 862", "Strip 863", "Strip 864", "Strip 865", "Strip 866", "Strip 867", "Strip 868", "Strip 869", "Strip 870", "Strip 871", "Strip 872", "Strip 873", "Strip 874", "Strip 875", "Strip 876", "Strip 877", "Strip 878", "Strip 879", "Strip 880", "Strip 881", "Strip 882", "Strip 883", "Strip 884", "Strip 885", "Strip 886", "Strip 887", "Strip 888", "Strip 889", "Strip 890", "Strip 891", "Strip 892", "Strip 893", "Strip 894", "Strip 895", "Strip 896", "Strip 897", "Strip 898", "Strip 899", "Strip 900", "Strip 901", "Strip 902", "Strip 903", "Strip 904", "Strip 905", "Strip 906", "Strip 907", "Strip 908", "Strip 909", "Strip 910", "Strip 911", "Strip 912", "Strip 913", "Strip 914", "Strip 915", "Strip 916", "Strip 917", "Strip 918", "Strip 919", "Strip 920", "Strip 921", "Strip 922", "Strip 923", "Strip 924", "Strip 925", "Strip 926", "Strip 927", "Strip 928", "Strip 929", "Strip 930", "Strip 931", "Strip 932", "Strip 933", "Strip 934", "Strip 935", "Strip 936", "Strip 937", "Strip 938", "Strip 939", "Strip 940", "Strip 941", "Strip 942", "Strip 943", "Strip 944", "Strip 945", "Strip 946", "Strip 947", "Strip 948", "Strip 949", "Strip 950", "Strip 951", "Strip 952", "Strip 953", "Strip 954", "Strip 955", "Strip 956", "Strip 957", "Strip 958", "Strip 959", "Strip 960", "Strip 961", "Strip 962", "Strip 963", "Strip 964", "Strip 965", "Strip 966", "Strip 967", "Strip 968", "Strip 969", "Strip 970", "Strip 971", "Strip 972", "Strip 973", "Strip 974", "Strip 975", "Strip 976", "Strip 977", "Strip 978", "Strip 979", "Strip 980", "Strip 981", "Strip 982", "Strip 983", "Strip 984", "Strip 985", "Strip 986", "Strip 987", "Strip 988", "Strip 989", "Strip 990", "Strip 991", "Strip 992", "Strip 993", "Strip 994", "Strip 995", "Strip 996", "Strip 997", "Strip 998", "Strip 999", "Strip 1000", "Strip 1001", "Strip 1002", "Strip 1003", "Strip 1004", "Strip 1005", "Strip 1006", "Strip 1007", "Strip 1008", "Strip 1009", "Strip 1010", "Strip 1011", "Strip 1012", "Strip 1013", "Strip 1014", "Strip 1015", "Strip 1016", "Strip 1017", "Strip 1018", "Strip 1019", "Strip 1020", "Strip 1021", "Strip 1022", "Strip 1023", "Strip 1024", "Strip 1025", "Strip 1026", "Strip 1027", "Strip 1028", "Strip 1029", "Strip 1030", "Strip 1031", "Strip 1032", "Strip 1033", "Strip 1034", "Strip 1035", "Strip 1036", "Strip 1037", "Strip 1038", "Strip 1039", "Strip 1040", "Strip 1041", "Strip 1042", "Strip 1043", "Strip 1044", "Strip 1045", "Strip 1046", "Strip 1047", "Strip 1048", "Strip 1049", "Strip 1050", "Strip 1051", "Strip 1052", "Strip 1053", "Strip 1054", "Strip 1055", "Strip 1056", "Strip 1057", "Strip 1058", "Strip 1059", "Strip 1060", "Strip 1061", "Strip 1062", "Strip 1063", "Strip 1064", "Strip 1065", "Strip 1066", "Strip 1067", "Strip 1068", "Strip 1069", "Strip 1070", "Strip 1071", "Strip 1072", "Strip 1073", "Strip 1074", "Strip 1075", "Strip 1076", "Strip 1077", "Strip 1078", "Strip 1079", "Strip 1080", "Strip 1081", "Strip 1082", "Strip 1083", "Strip 1084", "Strip 1085", "Strip 1086", "Strip 1087", "Strip 1088", "Strip 1089", "Strip 1090", "Strip 1091", "Strip 1092", "Strip 1093", "Strip 1094", "Strip 1095", "Strip 1096", "Strip 1097", "Strip 1098", "Strip 1099", "Strip 1100", "Strip 1101", "Strip 1102", "Strip 1103", "Strip 1104", "Strip 1105", "Strip 1106", "Strip 1107", "Strip 1108", "Strip 1109", "Strip 1110", "Strip 1111", "Strip 1112", "Strip 1113", "Strip 1114", "Strip 1115", "Strip 1116", "Strip 1117", "Strip 1118", "Strip 1119", "Strip 1120", "Strip 1121", "Strip 1122", "Strip 1123", "Strip 1124", "Strip 1125", "Strip 1126", "Strip 1127", "Strip 1128", "Strip 1129", "Strip 1130", "Strip 1131", "Strip 1132", "Strip 1133", "Strip 1134", "Strip 1135", "Strip 1136", "Strip 1137", "Strip 1138", "Strip 1139", "Strip 1140", "Strip 1141", "Strip 1142", "Strip 1143", "Strip 1144", "Strip 1145", "Strip 1146", "Strip 1147", "Strip 1148", "Strip 1149", "Strip 1150", "Strip 1151", "Strip 1152", "Strip 1153", "Strip 1154", "Strip 1155", "Strip 1156", "Strip 1157", "Strip 1158", "Strip 1159", "Strip 1160", "Strip 1161", "Strip 1162", "Strip 1163", "Strip 1164", "Strip 1165", "Strip 1166", "Strip 1167", "Strip 1168", "Strip 1169", "Strip 1170", "Strip 1171", "Strip 1172", "Strip 1173", "Strip 1174", "Strip 1175", "Strip 1176", "Strip 1177", "Strip 1178", "Strip 1179", "Strip 1180", "Strip 1181", "Strip 1182", "Strip 1183", "Strip 1184", "Strip 1185", "Strip 1186", "Strip 1187", "Strip 1188", "Strip 1189", "Strip 1190", "Strip 1191", "Strip 1192", "Strip 1193", "Strip 1194", "Strip 1195", "Strip 1196", "Strip 1197", "Strip 1198", "Strip 1199", "Strip 1200", "Strip 1201", "Strip 1202", "Strip 1203", "Strip 1204", "Strip 1205", "Strip 1206", "Strip 1207", "Strip 1208", "Strip 1209", "Strip 1210", "Strip 1211", "Strip 1212", "Strip 1213", "Strip 1214", "Strip 1215", "Strip 1216", "Strip 1217", "Strip 1218", "Strip 1219", "Strip 1220", "Strip 1221", "Strip 1222", "Strip 1223", "Strip 1224", "Strip 1225", "Strip 1226", "Strip 1227", "Strip 1228", "Strip 1229", "Strip 1230", "Strip 1231", "Strip 1232", "Strip 1233", "Strip 1234", "Strip 1235", "Strip 1236", "Strip 1237", "Strip 1238", "Strip 1239", "Strip 1240", "Strip 1241", "Strip 1242", "Strip 1243", "Strip 1244", "Strip 1245", "Strip 1246", "Strip 1247", "Strip 1248", "Strip 1249", "Strip 1250", "Strip 1251", "Strip 1252", "Strip 1253", "Strip 1254", "Strip 1255", "Strip 1256", "Strip 1257", "Strip 1258", "Strip 1259", "Strip 1260", "Strip 1261", "Strip 1262", "Strip 1263", "Strip 1264", "Strip 1265", "Strip 1266", "Strip 1267", "Strip 1268", "Strip 1269", "Strip 1270", "Strip 1271", "Strip 1272", "Strip 1273", "Strip 1274", "Strip 1275", "Strip 1276", "Strip 1277", "Strip 1278", "Strip 1279", "Strip 1280", "Strip 1281", "Strip 1282", "Strip 1283", "Strip 1284", "Strip 1285", "Strip 1286", "Strip 1287", "Strip 1288", "Strip 1289", "Strip 1290", "Strip 1291", "Strip 1292", "Strip 1293", "Strip 1294", "Strip 1295", "Strip 1296", "Strip 1297", "Strip 1298", "Strip 1299", "Strip 1300", "Strip 1301", "Strip 1302", "Strip 1303", "Strip 1304", "Strip 1305", "Strip 1306", "Strip 1307", "Strip 1308", "Strip 1309", "Strip 1310", "Strip 1311", "Strip 1312", "Strip 1313", "Strip 1314", "Strip 1315", "Strip 1316", "Strip 1317", "Strip 1318", "Strip 1319", "Strip 1320", "Strip 1321", "Strip 1322", "Strip 1323", "Strip 1324", "Strip 1325", "Strip 1326", "Strip 1327", "Strip 1328", "Strip 1329", "Strip 1330", "Strip 1331", "Strip 1332", "Strip 1333", "Strip 1334", "Strip 1335", "Strip 1336", "Strip 1337", "Strip 1338", "Strip 1339", "Strip 1340", "Strip 1341", "Strip 1342", "Strip 1343", "Strip 1344", "Strip 1345", "Strip 1346", "Strip 1347", "Strip 1348", "Strip 1349", "Strip 1350", "Strip 1351", "Strip 1352", "Strip 1353", "Strip 1354", "Strip 1355", "Strip 1356", "Strip 1357", "Strip 1358", "Strip 1359", "Strip 1360", "Strip 1361", "Strip 1362", "Strip 1363", "Strip 1364", "Strip 1365", "Strip 1366", "Strip 1367", "Strip 1368", "Strip 1369", "Strip 1370", "Strip 1371", "Strip 1372", "Strip 1373", "Strip 1374", "Strip 1375", "Strip 1376", "Strip 1377", "Strip 1378", "Strip 1379", "Strip 1380", "Strip 1381", "Strip 1382", "Strip 1383", "Strip 1384", "Strip 1385", "Strip 1386", "Strip 1387", "Strip 1388", "Strip 1389", "Strip 1390", "Strip 1391", "Strip 1392", "Strip 1393", "Strip 1394", "Strip 1395", "Strip 1396", "Strip 1397", "Strip 1398", "Strip 1399", "Strip 1400", "Strip 1401", "Strip 1402", "Strip 1403", "Strip 1404", "Strip 1405", "Strip 1406", "Strip 1407", "Strip 1408", "Strip 1409"]
  in  "To2":u16(ring) items=["Strip 0", "Strip 1", "Strip 2", "Strip 3", "Strip 4", "Strip 5", "Strip 6", "Strip 7", "Strip 8", "Strip 9", "Strip 10", "Strip 11", "Strip 12", "Strip 13", "Strip 14", "Strip 15", "Strip 16", "Strip 17", "Strip 18", "Strip 19", "Strip 20", "Strip 21", "Strip 22", "Strip 23", "Strip 24", "Strip 25", "Strip 26", "Strip 27", "Strip 28", "Strip 29", "Strip 30", "Strip 31", "Strip 32", "Strip 33", "Strip 34", "Strip 35", "Strip 36", "Strip 37", "Strip 38", "Strip 39", "Strip 40", "Strip 41", "Strip 42", "Strip 43", "Strip 44", "Strip 45", "Strip 46", "Strip 47", "Strip 48", "Strip 49", "Strip 50", "Strip 51", "Strip 52", "Strip 53", "Strip 54", "Strip 55", "Strip 56", "Strip 57", "Strip 58", "Strip 59", "Strip 60", "Strip 61", "Strip 62", "Strip 63", "Strip 64", "Strip 65", "Strip 66", "Strip 67", "Strip 68", "Strip 69", "Strip 70", "Strip 71", "Strip 72", "Strip 73", "Strip 74", "Strip 75", "Strip 76", "Strip 77", "Strip 78", "Strip 79", "Strip 80", "Strip 81", "Strip 82", "Strip 83", "Strip 84", "Strip 85", "Strip 86", "Strip 87", "Strip 88", "Strip 89", "Strip 90", "Strip 91", "Strip 92", "Strip 93", "Strip 94", "Strip 95", "Strip 96", "Strip 97", "Strip 98", "Strip 99", "Strip 100", "Strip 101", "Strip 102", "Strip 103", "Strip 104", "Strip 105", "Strip 106", "Strip 107", "Strip 108", "Strip 109", "Strip 110", "Strip 111", "Strip 112", "Strip 113", "Strip 114", "Strip 115", "Strip 116", "Strip 117", "Strip 118", "Strip 119", "Strip 120", "Strip 121", "Strip 122", "Strip 123", "Strip 124", "Strip 125", "Strip 126", "Strip 127", "Strip 128", "Strip 129", "Strip 130", "Strip 131", "Strip 132", "Strip 133", "Strip 134", "Strip 135", "Strip 136", "Strip 137", "Strip 138", "Strip 139", "Strip 140", "Strip 141", "Strip 142", "Strip 143", "Strip 144", "Strip 145", "Strip 146", "Strip 147", "Strip 148", "Strip 149", "Strip 150", "Strip 151", "Strip 152", "Strip 153", "Strip 154", "Strip 155", "Strip 156", "Strip 157", "Strip 158", "Strip 159", "Strip 160", "Strip 161", "Strip 162", "Strip 163", "Strip 164", "Strip 165", "Strip 166", "Strip 167", "Strip 168", "Strip 169", "Strip 170", "Strip 171", "Strip 172", "Strip 173", "Strip 174", "Strip 175", "Strip 176", "Strip 177", "Strip 178", "Strip 179", "Strip 180", "Strip 181", "Strip 182", "Strip 183", "Strip 184", "Strip 185", "Strip 186", "Strip 187", "Strip 188", "Strip 189", "Strip 190", "Strip 191", "Strip 192", "Strip 193", "Strip 194", "Strip 195", "Strip 196", "Strip 197", "Strip 198", "Strip 199", "Strip 200", "Strip 201", "Strip 202", "Strip 203", "Strip 204", "Strip 205", "Strip 206", "Strip 207", "Strip 208", "Strip 209", "Strip 210", "Strip 211", "Strip 212", "Strip 213", "Strip 214", "Strip 215", "Strip 216", "Strip 217", "Strip 218", "Strip 219", "Strip 220", "Strip 221", "Strip 222", "Strip 223", "Strip 224", "Strip 225", "Strip 226", "Strip 227", "Strip 228", "Strip 229", "Strip 230", "Strip 231", "Strip 232", "Strip 233", "Strip 234", "Strip 235", "Strip 236", "Strip 237", "Strip 238", "Strip 239", "Strip 240", "Strip 241", "Strip 242", "Strip 243", "Strip 244", "Strip 245", "Strip 246", "Strip 247", "Strip 248", "Strip 249", "Strip 250", "Strip 251", "Strip 252", "Strip 253", "Strip 254", "Strip 255", "Strip 256", "Strip 257", "Strip 258", "Strip 259", "Strip 260", "Strip 261", "Strip 262", "Strip 263", "Strip 264", "Strip 265", "Strip 266", "Strip 267", "Strip 268", "Strip 269", "Strip 270", "Strip 271", "Strip 272", "Strip 273", "Strip 274", "Strip 275", "Strip 276", "Strip 277", "Strip 278", "Strip 279", "Strip 280", "Strip 281", "Strip 282", "Strip 283", "Strip 284", "Strip 285", "Strip 286", "Strip 287", "Strip 288", "Strip 289", "Strip 290", "Strip 291", "Strip 292", "Strip 293", "Strip 294", "Strip 295", "Strip 296", "Strip 297", "Strip 298", "Strip 299", "Strip 300", "Strip 301", "Strip 302", "Strip 303", "Strip 304", "Strip 305", "Strip 306", "Strip 307", "Strip 308", "Strip 309", "Strip 310", "Strip 311", "Strip 312", "Strip 313", "Strip 314", "Strip 315", "Strip 316", "Strip 317", "Strip 318", "Strip 319", "Strip 320", "Strip 321", "Strip 322", "Strip 323", "Strip 324", "Strip 325", "Strip 326", "Strip 327", "Strip 328", "Strip 329", "Strip 330", "Strip 331", "Strip 332", "Strip 333", "Strip 334", "Strip 335", "Strip 336", "Strip 337", "Strip 338", "Strip 339", "Strip 340", "Strip 341", "Strip 342", "Strip 343", "Strip 344", "Strip 345", "Strip 346", "Strip 347", "Strip 348", "Strip 349", "Strip 350", "Strip 351", "Strip 352", "Strip 353", "Strip 354", "Strip 355", "Strip 356", "Strip 357", "Strip 358", "Strip 359", "Strip 360", "Strip 361", "Strip 362", "Strip 363", "Strip 364", "Strip 365", "Strip 366", "Strip 367", "Strip 368", "Strip 369", "Strip 370", "Strip 371", "Strip 372", "Strip 373", "Strip 374", "Strip 375", "Strip 376", "Strip 377", "Strip 378", "Strip 379", "Strip 380", "Strip 381", "Strip 382", "Strip 383", "Strip 384", "Strip 385", "Strip 386", "Strip 387", "Strip 388", "Strip 389", "Strip 390", "Strip 391", "Strip 392", "Strip 393", "Strip 394", "Strip 395", "Strip 396", "Strip 397", "Strip 398", "Strip 399", "Strip 400", "Strip 401", "Strip 402", "Strip 403", "Strip 404", "Strip 405", "Strip 406", "Strip 407", "Strip 408", "Strip 409", "Strip 410", "Strip 411", "Strip 412", "Strip 413", "Strip 414", "Strip 415", "Strip 416", "Strip 417", "Strip 418", "Strip 419", "Strip 420", "Strip 421", "Strip 422", "Strip 423", "Strip 424", "Strip 425", "Strip 426", "Strip 427", "Strip 428", "Strip 429", "Strip 430", "Strip 431", "Strip 432", "Strip 433", "Strip 434", "Strip 435", "Strip 436", "Strip 437", "Strip 438", "Strip 439", "Strip 440", "Strip 441", "Strip 442", "Strip 443", "Strip 444", "Strip 445", "Strip 446", "Strip 447", "Strip 448", "Strip 449", "Strip 450", "Strip 451", "Strip 452", "Strip 453", "Strip 454", "Strip 455", "Strip 456", "Strip 457", "Strip 458", "Strip 459", "Strip 460", "Strip 461", "Strip 462", "Strip 463", "Strip 464", "Strip 465", "Strip 466", "Strip 467", "Strip 468", "Strip 469", "Strip 470", "Strip 471", "Strip 472", "Strip 473", "Strip 474", "Strip 475", "Strip 476", "Strip 477", "Strip 478", "Strip 479", "Strip 480", "Strip 481", "Strip 482", "Strip 483", "Strip 484", "Strip 485", "Strip 486", "Strip 487", "Strip 488", "Strip 489", "Strip 490", "Strip 491", "Strip 492", "Strip 493", "Strip 494", "Strip 495", "Strip 496", "Strip 497", "Strip 498", "Strip 499", "Strip 500", "Strip 501", "Strip 502", "Strip 503", "Strip 504", "Strip 505", "Strip 506", "Strip 507", "Strip 508", "Strip 509", "Strip 510", "Strip 511", "Strip 512", "Strip 513", "Strip 514", "Strip 515", "Strip 516", "Strip 517", "Strip 518", "Strip 519", "Strip 520", "Strip 521", "Strip 522", "Strip 523", "Strip 524", "Strip 525", "Strip 526", "Strip 527", "Strip 528", "Strip 529", "Strip 530", "Strip 531", "Strip 532", "Strip 533", "Strip 534", "Strip 535", "Strip 536", "Strip 537", "Strip 538", "Strip 539", "Strip 540", "Strip 541", "Strip 542", "Strip 543", "Strip 544", "Strip 545", "Strip 546", "Strip 547", "Strip 548", "Strip 549", "Strip 550", "Strip 551", "Strip 552", "Strip 553", "Strip 554", "Strip 555", "Strip 556", "Strip 557", "Strip 558", "Strip 559", "Strip 560", "Strip 561", "Strip 562", "Strip 563", "Strip 564", "Strip 565", "Strip 566", "Strip 567", "Strip 568", "Strip 569", "Strip 570", "Strip 571", "Strip 572", "Strip 573", "Strip 574", "Strip 575", "Strip 576", "Strip 577", "Strip 578", "Strip 579", "Strip 580", "Strip 581", "Strip 582", "Strip 583", "Strip 584", "Strip 585", "Strip 586", "Strip 587", "Strip 588", "Strip 589", "Strip 590", "Strip 591", "Strip 592", "Strip 593", "Strip 594", "Strip 595", "Strip 596", "Strip 597", "Strip 598", "Strip 599", "Strip 600", "Strip 601", "Strip 602", "Strip 603", "Strip 604", "Strip 605", "Strip 606", "Strip 607", "Strip 608", "Strip 609", "Strip 610", "Strip 611", "Strip 612", "Strip 613", "Strip 614", "Strip 615", "Strip 616", "Strip 617", "Strip 618", "Strip 619", "Strip 620", "Strip 621", "Strip 622", "Strip 623", "Strip 624", "Strip 625", "Strip 626", "Strip 627", "Strip 628", "Strip 629", "Strip 630", "Strip 631", "Strip 632", "Strip 633", "Strip 634", "Strip 635", "Strip 636", "Strip 637", "Strip 638", "Strip 639", "Strip 640", "Strip 641", "Strip 642", "Strip 643", "Strip 644", "Strip 645", "Strip 646", "Strip 647", "Strip 648", "Strip 649", "Strip 650", "Strip 651", "Strip 652", "Strip 653", "Strip 654", "Strip 655", "Strip 656", "Strip 657", "Strip 658", "Strip 659", "Strip 660", "Strip 661", "Strip 662", "Strip 663", "Strip 664", "Strip 665", "Strip 666", "Strip 667", "Strip 668", "Strip 669", "Strip 670", "Strip 671", "Strip 672", "Strip 673", "Strip 674", "Strip 675", "Strip 676", "Strip 677", "Strip 678", "Strip 679", "Strip 680", "Strip 681", "Strip 682", "Strip 683", "Strip 684", "Strip 685", "Strip 686", "Strip 687", "Strip 688", "Strip 689", "Strip 690", "Strip 691", "Strip 692", "Strip 693", "Strip 694", "Strip 695", "Strip 696", "Strip 697", "Strip 698", "Strip 699", "Strip 700", "Strip 701", "Strip 702", "Strip 703", "Strip 704", "Strip 705", "Strip 706", "Strip 707", "Strip 708", "Strip 709", "Strip 710", "Strip 711", "Strip 712", "Strip 713", "Strip 714", "Strip 715", "Strip 716", "Strip 717", "Strip 718", "Strip 719", "Strip 720", "Strip 721", "Strip 722", "Strip 723", "Strip 724", "Strip 725", "Strip 726", "Strip 727", "Strip 728", "Strip 729", "Strip 730", "Strip 731", "Strip 732", "Strip 733", "Strip 734", "Strip 735", "Strip 736", "Strip 737", "Strip 738", "Strip 739", "Strip 740", "Strip 741", "Strip 742", "Strip 743", "Strip 744", "Strip 745", "Strip 746", "Strip 747", "Strip 748", "Strip 749", "Strip 750", "Strip 751", "Strip 752", "Strip 753", "Strip 754", "Strip 755", "Strip 756", "Strip 757", "Strip 758", "Strip 759", "Strip 760", "Strip 761", "Strip 762", "Strip 763", "Strip 764", "Strip 765", "Strip 766", "Strip 767", "Strip 768", "Strip 769", "Strip 770", "Strip 771", "Strip 772", "Strip 773", "Strip 774", "Strip 775", "Strip 776", "Strip 777", "Strip 778", "Strip 779", "Strip 780", "Strip 781", "Strip 782", "Strip 783", "Strip 784", "Strip 785", "Strip 786", "Strip 787", "Strip 788", "Strip 789", "Strip 790", "Strip 791", "Strip 792", "Strip 793", "Strip 794", "Strip 795", "Strip 796", "Strip 797", "Strip 798", "Strip 799", "Strip 800", "Strip 801", "Strip 802", "Strip 803", "Strip 804", "Strip 805", "Strip 806", "Strip 807", "Strip 808", "Strip 809", "Strip 810", "Strip 811", "Strip 812", "Strip 813", "Strip 814", "Strip 815", "Strip 816", "Strip 817", "Strip 818", "Strip 819", "Strip 820", "Strip 821", "Strip 822", "Strip 823", "Strip 824", "Strip 825", "Strip 826", "Strip 827", "Strip 828", "Strip 829", "Strip 830", "Strip 831", "Strip 832", "Strip 833", "Strip 834", "Strip 835", "Strip 836", "Strip 837", "Strip 838", "Strip 839", "Strip 840", "Strip 841", "Strip 842", "Strip 843", "Strip 844", "Strip 845", "Strip 846", "Strip 847", "Strip 848", "Strip 849", "Strip 850", "Strip 851", "Strip 852", "Strip 853", "Strip 854", "Strip 855", "Strip 856", "Strip 857", "Strip 858", "Strip 859", "Strip 860", "Strip 861", "Strip 862", "Strip 863", "Strip 864", "Strip 865", "Strip 866", "Strip 867", "Strip 868", "Strip 869", "Strip 870", "Strip 871", "Strip 872", "Strip 873", "Strip 874", "Strip 875", "Strip 876", "Strip 877", "Strip 878", "Strip 879", "Strip 880", "Strip 881", "Strip 882", "Strip 883", "Strip 884", "Strip 885", "Strip 886", "Strip 887", "Strip 888", "Strip 889", "Strip 890", "Strip 891", "Strip 892", "Strip 893", "Strip 894", "Strip 895", "Strip 896", "Strip 897", "Strip 898", "Strip 899", "Strip 900", "Strip 901", "Strip 902", "Strip 903", "Strip 904", "Strip 905", "Strip 906", "Strip 907", "Strip 908", "Strip 909", "Strip 910", "Strip 911", "Strip 912", "Strip 913", "Strip 914", "Strip 915", "Strip 916", "Strip 917", "Strip 918", "Strip 919", "Strip 920", "Strip 921", "Strip 922", "Strip 923", "Strip 924", "Strip 925", "Strip 926", "Strip 927", "Strip 928", "Strip 929", "Strip 930", "Strip 931", "Strip 932", "Strip 933", "Strip 934", "Strip 935", "Strip 936", "Strip 937", "Strip 938", "Strip 939", "Strip 940", "Strip 941", "Strip 942", "Strip 943", "Strip 944", "Strip 945", "Strip 946", "Strip 947", "Strip 948", "Strip 949", "Strip 950", "Strip 951", "Strip 952", "Strip 953", "Strip 954", "Strip 955", "Strip 956", "Strip 957", "Strip 958", "Strip 959", "Strip 960", "Strip 961", "Strip 962", "Strip 963", "Strip 964", "Strip 965", "Strip 966", "Strip 967", "Strip 968", "Strip 969", "Strip 970", "Strip 971", "Strip 972", "Strip 973", "Strip 974", "Strip 975", "Strip 976", "Strip 977", "Strip 978", "Strip 979", "Strip 980", "Strip 981", "Strip 982", "Strip 983", "Strip 984", "Strip 985", "Strip 986", "Strip 987", "Strip 988", "Strip 989", "Strip 990", "Strip 991", "Strip 992", "Strip 993", "Strip 994", "Strip 995", "Strip 996", "Strip 997", "Strip 998", "Strip 999", "Strip 1000", "Strip 1001", "Strip 1002", "Strip 1003", "Strip 1004", "Strip 1005", "Strip 1006", "Strip 1007", "Strip 1008", "Strip 1009", "Strip 1010", "Strip 1011", "Strip 1012", "Strip 1013", "Strip 1014", "Strip 1015", "Strip 1016", "Strip 1017", "Strip 1018", "Strip 1019", "Strip 1020", "Strip 1021", "Strip 1022", "Strip 1023", "Strip 1024", "Strip 1025", "Strip 1026", "Strip 1027", "Strip 1028", "Strip 1029", "Strip 1030", "Strip 1031", "Strip 1032", "Strip 1033", "Strip 1034", "Strip 1035", "Strip 1036", "Strip 1037", "Strip 1038", "Strip 1039", "Strip 1040", "Strip 1041", "Strip 1042", "Strip 1043", "Strip 1044", "Strip 1045", "Strip 1046", "Strip 1047", "Strip 1048", "Strip 1049", "Strip 1050", "Strip 1051", "Strip 1052", "Strip 1053", "Strip 1054", "Strip 1055", "Strip 1056", "Strip 1057", "Strip 1058", "Strip 1059", "Strip 1060", "Strip 1061", "Strip 1062", "Strip 1063", "Strip 1064", "Strip 1065", "Strip 1066", "Strip 1067", "Strip 1068", "Strip 1069", "Strip 1070", "Strip 1071", "Strip 1072", "Strip 1073", "Strip 1074", "Strip 1075", "Strip 1076", "Strip 1077", "Strip 1078", "Strip 1079", "Strip 1080", "Strip 1081", "Strip 1082", "Strip 1083", "Strip 1084", "Strip 1085", "Strip 1086", "Strip 1087", "Strip 1088", "Strip 1089", "Strip 1090", "Strip 1091", "Strip 1092", "Strip 1093", "Strip 1094", "Strip 1095", "Strip 1096", "Strip 1097", "Strip 1098", "Strip 1099", "Strip 1100", "Strip 1101", "Strip 1102", "Strip 1103", "Strip 1104", "Strip 1105", "Strip 1106", "Strip 1107", "Strip 1108", "Strip 1109", "Strip 1110", "Strip 1111", "Strip 1112", "Strip 1113", "Strip 1114", "Strip 1115", "Strip 1116", "Strip 1117", "Strip 1118", "Strip 1119", "Strip 1120", "Strip 1121", "Strip 1122", "Strip 1123", "Strip 1124", "Strip 1125", "Strip 1126", "Strip 1127", "Strip 1128", "Strip 1129", "Strip 1130", "Strip 1131", "Strip 1132", "Strip 1133", "Strip 1134", "Strip 1135", "Strip 1136", "Strip 1137", "Strip 1138", "Strip 1139", "Strip 1140", "Strip 1141", "Strip 1142", "Strip 1143", "Strip 1144", "Strip 1145", "Strip 1146", "Strip 1147", "Strip 1148", "Strip 1149", "Strip 1150", "Strip 1151", "Strip 1152", "Strip 1153"]
  in  "To 1":u16(ring) caption="To" items=["Strip 0", "Strip 1", "Strip 2", "Strip 3", "Strip 4", "Strip 5", "Strip 6", "Strip 7", "Strip 8", "Strip 9", "Strip 10", "Strip 11", "Strip 12", "Strip 13", "Strip 14", "Strip 15", "Strip 16", "Strip 17", "Strip 18", "Strip 19", "Strip 20", "Strip 21", "Strip 22", "Strip 23", "Strip 24", "Strip 25", "Strip 26", "Strip 27", "Strip 28", "Strip 29", "Strip 30", "Strip 31", "Strip 32", "Strip 33", "Strip 34", "Strip 35", "Strip 36", "Strip 37", "Strip 38", "Strip 39", "Strip 40", "Strip 41", "Strip 42", "Strip 43", "Strip 44", "Strip 45", "Strip 46", "Strip 47", "Strip 48", "Strip 49", "Strip 50", "Strip 51", "Strip 52", "Strip 53", "Strip 54", "Strip 55", "Strip 56", "Strip 57", "Strip 58", "Strip 59", "Strip 60", "Strip 61", "Strip 62", "Strip 63", "Strip 64", "Strip 65", "Strip 66", "Strip 67", "Strip 68", "Strip 69", "Strip 70", "Strip 71", "Strip 72", "Strip 73", "Strip 74", "Strip 75", "Strip 76", "Strip 77", "Strip 78", "Strip 79", "Strip 80", "Strip 81", "Strip 82", "Strip 83", "Strip 84", "Strip 85", "Strip 86", "Strip 87", "Strip 88", "Strip 89", "Strip 90", "Strip 91", "Strip 92", "Strip 93", "Strip 94", "Strip 95", "Strip 96", "Strip 97", "Strip 98", "Strip 99", "Strip 100", "Strip 101", "Strip 102", "Strip 103", "Strip 104", "Strip 105", "Strip 106", "Strip 107", "Strip 108", "Strip 109", "Strip 110", "Strip 111", "Strip 112", "Strip 113", "Strip 114", "Strip 115", "Strip 116", "Strip 117", "Strip 118", "Strip 119", "Strip 120", "Strip 121", "Strip 122", "Strip 123", "Strip 124", "Strip 125", "Strip 126", "Strip 127", "Strip 128", "Strip 129", "Strip 130", "Strip 131", "Strip 132", "Strip 133", "Strip 134", "Strip 135", "Strip 136", "Strip 137", "Strip 138", "Strip 139", "Strip 140", "Strip 141", "Strip 142", "Strip 143", "Strip 144", "Strip 145", "Strip 146", "Strip 147", "Strip 148", "Strip 149", "Strip 150", "Strip 151", "Strip 152", "Strip 153", "Strip 154", "Strip 155", "Strip 156", "Strip 157", "Strip 158", "Strip 159", "Strip 160", "Strip 161", "Strip 162", "Strip 163", "Strip 164", "Strip 165", "Strip 166", "Strip 167", "Strip 168", "Strip 169", "Strip 170", "Strip 171", "Strip 172", "Strip 173", "Strip 174", "Strip 175", "Strip 176", "Strip 177", "Strip 178", "Strip 179", "Strip 180", "Strip 181", "Strip 182", "Strip 183", "Strip 184", "Strip 185", "Strip 186", "Strip 187", "Strip 188", "Strip 189", "Strip 190", "Strip 191", "Strip 192", "Strip 193", "Strip 194", "Strip 195", "Strip 196", "Strip 197", "Strip 198", "Strip 199", "Strip 200", "Strip 201", "Strip 202", "Strip 203", "Strip 204", "Strip 205", "Strip 206", "Strip 207", "Strip 208", "Strip 209", "Strip 210", "Strip 211", "Strip 212", "Strip 213", "Strip 214", "Strip 215", "Strip 216", "Strip 217", "Strip 218", "Strip 219", "Strip 220", "Strip 221", "Strip 222", "Strip 223", "Strip 224", "Strip 225", "Strip 226", "Strip 227", "Strip 228", "Strip 229", "Strip 230", "Strip 231", "Strip 232", "Strip 233", "Strip 234", "Strip 235", "Strip 236", "Strip 237", "Strip 238", "Strip 239", "Strip 240", "Strip 241", "Strip 242", "Strip 243", "Strip 244", "Strip 245", "Strip 246", "Strip 247", "Strip 248", "Strip 249", "Strip 250", "Strip 251", "Strip 252", "Strip 253", "Strip 254", "Strip 255", "Strip 256", "Strip 257", "Strip 258", "Strip 259", "Strip 260", "Strip 261", "Strip 262", "Strip 263", "Strip 264", "Strip 265", "Strip 266", "Strip 267", "Strip 268", "Strip 269", "Strip 270", "Strip 271", "Strip 272", "Strip 273", "Strip 274", "Strip 275", "Strip 276", "Strip 277", "Strip 278", "Strip 279", "Strip 280", "Strip 281", "Strip 282", "Strip 283", "Strip 284", "Strip 285", "Strip 286", "Strip 287", "Strip 288", "Strip 289", "Strip 290", "Strip 291", "Strip 292", "Strip 293", "Strip 294", "Strip 295", "Strip 296", "Strip 297", "Strip 298", "Strip 299", "Strip 300", "Strip 301", "Strip 302", "Strip 303", "Strip 304", "Strip 305", "Strip 306", "Strip 307", "Strip 308", "Strip 309", "Strip 310", "Strip 311", "Strip 312", "Strip 313", "Strip 314", "Strip 315", "Strip 316", "Strip 317", "Strip 318", "Strip 319", "Strip 320", "Strip 321", "Strip 322", "Strip 323", "Strip 324", "Strip 325", "Strip 326", "Strip 327", "Strip 328", "Strip 329", "Strip 330", "Strip 331", "Strip 332", "Strip 333", "Strip 334", "Strip 335", "Strip 336", "Strip 337", "Strip 338", "Strip 339", "Strip 340", "Strip 341", "Strip 342", "Strip 343", "Strip 344", "Strip 345", "Strip 346", "Strip 347", "Strip 348", "Strip 349", "Strip 350", "Strip 351", "Strip 352", "Strip 353", "Strip 354", "Strip 355", "Strip 356", "Strip 357", "Strip 358", "Strip 359", "Strip 360", "Strip 361", "Strip 362", "Strip 363", "Strip 364", "Strip 365", "Strip 366", "Strip 367", "Strip 368", "Strip 369", "Strip 370", "Strip 371", "Strip 372", "Strip 373", "Strip 374", "Strip 375", "Strip 376", "Strip 377", "Strip 378", "Strip 379", "Strip 380", "Strip 381", "Strip 382", "Strip 383", "Strip 384", "Strip 385", "Strip 386", "Strip 387", "Strip 388", "Strip 389", "Strip 390", "Strip 391", "Strip 392", "Strip 393", "Strip 394", "Strip 395", "Strip 396", "Strip 397", "Strip 398", "Strip 399", "Strip 400", "Strip 401", "Strip 402", "Strip 403", "Strip 404", "Strip 405", "Strip 406", "Strip 407", "Strip 408", "Strip 409", "Strip 410", "Strip 411", "Strip 412", "Strip 413", "Strip 414", "Strip 415", "Strip 416", "Strip 417", "Strip 418", "Strip 419", "Strip 420", "Strip 421", "Strip 422", "Strip 423", "Strip 424", "Strip 425", "Strip 426", "Strip 427", "Strip 428", "Strip 429", "Strip 430", "Strip 431", "Strip 432", "Strip 433", "Strip 434", "Strip 435", "Strip 436", "Strip 437", "Strip 438", "Strip 439", "Strip 440", "Strip 441", "Strip 442", "Strip 443", "Strip 444", "Strip 445", "Strip 446", "Strip 447", "Strip 448", "Strip 449", "Strip 450", "Strip 451", "Strip 452", "Strip 453", "Strip 454", "Strip 455", "Strip 456", "Strip 457", "Strip 458", "Strip 459", "Strip 460", "Strip 461", "Strip 462", "Strip 463", "Strip 464", "Strip 465", "Strip 466", "Strip 467", "Strip 468", "Strip 469", "Strip 470", "Strip 471", "Strip 472", "Strip 473", "Strip 474", "Strip 475", "Strip 476", "Strip 477", "Strip 478", "Strip 479", "Strip 480", "Strip 481", "Strip 482", "Strip 483", "Strip 484", "Strip 485", "Strip 486", "Strip 487", "Strip 488", "Strip 489", "Strip 490", "Strip 491", "Strip 492", "Strip 493", "Strip 494", "Strip 495", "Strip 496", "Strip 497", "Strip 498", "Strip 499", "Strip 500", "Strip 501", "Strip 502", "Strip 503", "Strip 504", "Strip 505", "Strip 506", "Strip 507", "Strip 508", "Strip 509", "Strip 510", "Strip 511", "Strip 512", "Strip 513", "Strip 514", "Strip 515", "Strip 516", "Strip 517", "Strip 518", "Strip 519", "Strip 520", "Strip 521", "Strip 522", "Strip 523", "Strip 524", "Strip 525", "Strip 526", "Strip 527", "Strip 528", "Strip 529", "Strip 530", "Strip 531", "Strip 532", "Strip 533", "Strip 534", "Strip 535", "Strip 536", "Strip 537", "Strip 538", "Strip 539", "Strip 540", "Strip 541", "Strip 542", "Strip 543", "Strip 544", "Strip 545", "Strip 546", "Strip 547", "Strip 548", "Strip 549", "Strip 550", "Strip 551", "Strip 552", "Strip 553", "Strip 554", "Strip 555", "Strip 556", "Strip 557", "Strip 558", "Strip 559", "Strip 560", "Strip 561", "Strip 562", "Strip 563", "Strip 564", "Strip 565", "Strip 566", "Strip 567", "Strip 568", "Strip 569", "Strip 570", "Strip 571", "Strip 572", "Strip 573", "Strip 574", "Strip 575", "Strip 576", "Strip 577", "Strip 578", "Strip 579", "Strip 580", "Strip 581", "Strip 582", "Strip 583", "Strip 584", "Strip 585", "Strip 586", "Strip 587", "Strip 588", "Strip 589", "Strip 590", "Strip 591", "Strip 592", "Strip 593", "Strip 594", "Strip 595", "Strip 596", "Strip 597", "Strip 598", "Strip 599", "Strip 600", "Strip 601", "Strip 602", "Strip 603", "Strip 604", "Strip 605", "Strip 606", "Strip 607", "Strip 608", "Strip 609", "Strip 610", "Strip 611", "Strip 612", "Strip 613", "Strip 614", "Strip 615", "Strip 616", "Strip 617", "Strip 618", "Strip 619", "Strip 620", "Strip 621", "Strip 622", "Strip 623", "Strip 624", "Strip 625", "Strip 626", "Strip 627", "Strip 628", "Strip 629", "Strip 630", "Strip 631", "Strip 632", "Strip 633", "Strip 634", "Strip 635", "Strip 636", "Strip 637", "Strip 638", "Strip 639", "Strip 640", "Strip 641", "Strip 642", "Strip 643", "Strip 644", "Strip 645", "Strip 646", "Strip 647", "Strip 648", "Strip 649", "Strip 650", "Strip 651", "Strip 652", "Strip 653", "Strip 654", "Strip 655", "Strip 656", "Strip 657", "Strip 658", "Strip 659", "Strip 660", "Strip 661", "Strip 662", "Strip 663", "Strip 664", "Strip 665", "Strip 666", "Strip 667", "Strip 668", "Strip 669", "Strip 670", "Strip 671", "Strip 672", "Strip 673", "Strip 674", "Strip 675", "Strip 676", "Strip 677", "Strip 678", "Strip 679", "Strip 680", "Strip 681", "Strip 682", "Strip 683", "Strip 684", "Strip 685", "Strip 686", "Strip 687", "Strip 688", "Strip 689", "Strip 690", "Strip 691", "Strip 692", "Strip 693", "Strip 694", "Strip 695", "Strip 696", "Strip 697", "Strip 698", "Strip 699", "Strip 700", "Strip 701", "Strip 702", "Strip 703", "Strip 704", "Strip 705", "Strip 706", "Strip 707", "Strip 708", "Strip 709", "Strip 710", "Strip 711", "Strip 712", "Strip 713", "Strip 714", "Strip 715", "Strip 716", "Strip 717", "Strip 718", "Strip 719", "Strip 720", "Strip 721", "Strip 722", "Strip 723", "Strip 724", "Strip 725", "Strip 726", "Strip 727", "Strip 728", "Strip 729", "Strip 730", "Strip 731", "Strip 732", "Strip 733", "Strip 734", "Strip 735", "Strip 736", "Strip 737", "Strip 738", "Strip 739", "Strip 740", "Strip 741", "Strip 742", "Strip 743", "Strip 744", "Strip 745", "Strip 746", "Strip 747", "Strip 748", "Strip 749", "Strip 750", "Strip 751", "Strip 752", "Strip 753", "Strip 754", "Strip 755", "Strip 756", "Strip 757", "Strip 758", "Strip 759", "Strip 760", "Strip 761", "Strip 762", "Strip 763", "Strip 764", "Strip 765", "Strip 766", "Strip 767", "Strip 768", "Strip 769", "Strip 770", "Strip 771", "Strip 772", "Strip 773", "Strip 774", "Strip 775", "Strip 776", "Strip 777", "Strip 778", "Strip 779", "Strip 780", "Strip 781", "Strip 782", "Strip 783", "Strip 784", "Strip 785", "Strip 786", "Strip 787", "Strip 788", "Strip 789", "Strip 790", "Strip 791", "Strip 792", "Strip 793", "Strip 794", "Strip 795", "Strip 796", "Strip 797", "Strip 798", "Strip 799", "Strip 800", "Strip 801", "Strip 802", "Strip 803", "Strip 804", "Strip 805", "Strip 806", "Strip 807", "Strip 808", "Strip 809", "Strip 810", "Strip 811", "Strip 812", "Strip 813", "Strip 814", "Strip 815", "Strip 816", "Strip 817", "Strip 818", "Strip 819", "Strip 820", "Strip 821", "Strip 822", "Strip 823", "Strip 824", "Strip 825", "Strip 826", "Strip 827", "Strip 828", "Strip 829", "Strip 830", "Strip 831", "Strip 832", "Strip 833", "Strip 834", "Strip 835", "Strip 836", "Strip 837", "Strip 838", "Strip 839", "Strip 840", "Strip 841", "Strip 842", "Strip 843", "Strip 844", "Strip 845", "Strip 846", "Strip 847", "Strip 848", "Strip 849", "Strip 850", "Strip 851", "Strip 852", "Strip 853", "Strip 854", "Strip 855", "Strip 856", "Strip 857", "Strip 858", "Strip 859", "Strip 860", "Strip 861", "Strip 862", "Strip 863", "Strip 864", "Strip 865", "Strip 866", "Strip 867", "Strip 868", "Strip 869", "Strip 870", "Strip 871", "Strip 872", "Strip 873", "Strip 874", "Strip 875", "Strip 876", "Strip 877", "Strip 878", "Strip 879", "Strip 880", "Strip 881", "Strip 882", "Strip 883", "Strip 884", "Strip 885", "Strip 886", "Strip 887", "Strip 888", "Strip 889", "Strip 890", "Strip 891", "Strip 892", "Strip 893", "Strip 894", "Strip 895", "Strip 896", "Strip 897", "Strip 898", "Strip 899", "Strip 900", "Strip 901", "Strip 902", "Strip 903", "Strip 904", "Strip 905", "Strip 906", "Strip 907", "Strip 908", "Strip 909", "Strip 910", "Strip 911", "Strip 912", "Strip 913", "Strip 914", "Strip 915", "Strip 916", "Strip 917", "Strip 918", "Strip 919", "Strip 920", "Strip 921", "Strip 922", "Strip 923", "Strip 924", "Strip 925", "Strip 926", "Strip 927", "Strip 928", "Strip 929", "Strip 930", "Strip 931", "Strip 932", "Strip 933", "Strip 934", "Strip 935", "Strip 936", "Strip 937", "Strip 938", "Strip 939", "Strip 940", "Strip 941", "Strip 942", "Strip 943", "Strip 944", "Strip 945", "Strip 946", "Strip 947", "Strip 948", "Strip 949", "Strip 950", "Strip 951", "Strip 952", "Strip 953", "Strip 954", "Strip 955", "Strip 956", "Strip 957", "Strip 958", "Strip 959", "Strip 960", "Strip 961", "Strip 962", "Strip 963", "Strip 964", "Strip 965", "Strip 966", "Strip 967", "Strip 968", "Strip 969", "Strip 970", "Strip 971", "Strip 972", "Strip 973", "Strip 974", "Strip 975", "Strip 976", "Strip 977", "Strip 978", "Strip 979", "Strip 980", "Strip 981", "Strip 982", "Strip 983", "Strip 984", "Strip 985", "Strip 986", "Strip 987", "Strip 988", "Strip 989", "Strip 990", "Strip 991", "Strip 992", "Strip 993", "Strip 994", "Strip 995", "Strip 996", "Strip 997", "Strip 998", "Strip 999", "Strip 1000", "Strip 1001", "Strip 1002", "Strip 1003", "Strip 1004", "Strip 1005", "Strip 1006", "Strip 1007", "Strip 1008", "Strip 1009", "Strip 1010", "Strip 1011", "Strip 1012", "Strip 1013", "Strip 1014", "Strip 1015", "Strip 1016", "Strip 1017", "Strip 1018", "Strip 1019", "Strip 1020", "Strip 1021", "Strip 1022", "Strip 1023", "Strip 1024", "Strip 1025", "Strip 1026", "Strip 1027", "Strip 1028", "Strip 1029", "Strip 1030", "Strip 1031", "Strip 1032", "Strip 1033", "Strip 1034", "Strip 1035", "Strip 1036", "Strip 1037", "Strip 1038", "Strip 1039", "Strip 1040", "Strip 1041", "Strip 1042", "Strip 1043", "Strip 1044", "Strip 1045", "Strip 1046", "Strip 1047", "Strip 1048", "Strip 1049", "Strip 1050", "Strip 1051", "Strip 1052", "Strip 1053", "Strip 1054", "Strip 1055", "Strip 1056", "Strip 1057", "Strip 1058", "Strip 1059", "Strip 1060", "Strip 1061", "Strip 1062", "Strip 1063", "Strip 1064", "Strip 1065", "Strip 1066", "Strip 1067", "Strip 1068", "Strip 1069", "Strip 1070", "Strip 1071", "Strip 1072", "Strip 1073", "Strip 1074", "Strip 1075", "Strip 1076", "Strip 1077", "Strip 1078", "Strip 1079", "Strip 1080", "Strip 1081", "Strip 1082", "Strip 1083", "Strip 1084", "Strip 1085", "Strip 1086", "Strip 1087", "Strip 1088", "Strip 1089", "Strip 1090", "Strip 1091", "Strip 1092", "Strip 1093", "Strip 1094", "Strip 1095", "Strip 1096", "Strip 1097", "Strip 1098", "Strip 1099", "Strip 1100", "Strip 1101", "Strip 1102", "Strip 1103", "Strip 1104", "Strip 1105", "Strip 1106", "Strip 1107", "Strip 1108", "Strip 1109", "Strip 1110", "Strip 1111", "Strip 1112", "Strip 1113", "Strip 1114", "Strip 1115", "Strip 1116", "Strip 1117", "Strip 1118", "Strip 1119", "Strip 1120", "Strip 1121", "Strip 1122", "Strip 1123", "Strip 1124", "Strip 1125", "Strip 1126", "Strip 1127", "Strip 1128", "Strip 1129", "Strip 1130", "Strip 1131", "Strip 1132", "Strip 1133", "Strip 1134", "Strip 1135", "Strip 1136", "Strip 1137", "Strip 1138", "Strip 1139", "Strip 1140", "Strip 1141", "Strip 1142", "Strip 1143", "Strip 1144", "Strip 1145", "Strip 1146", "Strip 1147", "Strip 1148", "Strip 1149", "Strip 1150", "Strip 1151", "Strip 1152", "Strip 1153"]
  out "Region 1":string caption="Region"
  out "Region2":string
  out "Region3":string
  out "Region4":string
  in  "Enable1":bool
  in  "Enable4":bool
  in  "Enable2":bool
  in  "Enable3":bool
  in  "Pinhole Parameters IN":T1={"Base Voltage"=10.0, "Base Ramp [V/step]"=10.0, "Base Step [ms]"=1000, "High Voltage"=100.0, "High Ramp [V/step]"=100.0, "High Step [ms]"=1000} caption="Pinhole Measurement Parameters"
  in  "Manufacturer:":string(combo)="Hamamatsu"
  in  "Thresholds:":T2={"Current [nA]"=200.0, "Ccoupl Lo [pF/cm]"=20.0, "Ccoupl Hi [pF/cm]"=33.0, "Rbias Lo [MW]"=1.0, "Rbias Hi [MW]"=2.0}
  in  "settling\ndelay [ms]":i32=50
  in  "Pinhole Parameters":T1={"Base Voltage"=10.0, "Base Ramp [V/step]"=10.0, "Base Step [ms]"=1000, "High Voltage"=100.0, "High Ramp [V/step]"=100.0, "High Step [ms]"=1000}
  out "Bias On/Off:":bool
  in  "Auto quit &\nswitch off bias":bool
  out "Sensor No.:":string
  out "Device Category:":string
  out "DB Serial No.:":string
  out "Initiated:":string
  in  "Save Data":bool
  in  "Abort":bool
  in  "Quit w/o saving":bool
  out "Probing Region:":string
  out "Probe Point:":string
  out "Current [nA]:":dbl
  out "Capacitance [pF]:":dbl
  out "Reistance [MW]:":dbl
  out "Last Probe at:":string
  out "Run Duration:":string
  out "Estimated Completion:":string
  out "Status:":string
  out "Probe Card Channels":i32=32
  in  "Show:":u16(ring) items=["Segment_2"=1]
  out "Defects":i32[][](graph)
  out "% OK:":dbl
  out "# total defects:":i32
  out "# probed":i32
  out "Bad Strip List":i32[](array[numeric])
  out "defect type array":i32[](array[numeric])
  out "Resistance [MW]":cluster{u32, i32, "Array OUT":dbl[]}(graph)
  out "Capacitance [pF]":cluster{u32, i32, "Array OUT":dbl[]}(graph)
  out "Current [nA]":cluster{u32, i32, "Array OUT":dbl[]}(graph)
  out "Current Reference 100V":dbl[](array[numeric])
  out "Current Reference 10V":dbl[](array[numeric])
  out "Single Needle":bool
  out "Z profile":i32[][](array[numeric])
  out "Start Temperature [°C]":dbl
  out "Last Temperature [°C]":dbl
  out "disabled channels":i32[](array[numeric])
  out "Module failed/passed":bool
  out "probe points per region":i32[](array[numeric])
  out "min scale array":i32[](array[numeric])
  out "max scale array":i32[](array[numeric])
  out "total strip number":u32
  out "Region Indices":i32[](array[numeric])
  out "Current Bias Voltage [V]":dbl
  out "Temperature Progression":T3
  # "Sensor QC: Striptest"
  # "University of \nCambridge"
  # "Current [nA]"
  # "Statistical information:"
  # "Capacitance [pF]"
  # "Pinholes:"
  # "Punchthroughs:"
  # "Shorts:"
  # "Opens:"
  # "Rpoly:"
  # "Resistance [MW]"
  # "Implant:"
  # "Current segment:"
  # "Ok  Pinhole at base  Pinhole after ramp  Short  Open  Rbias"
  # "Probe Range"
  # "Measurement Configuration"
  # "Hardware"
  # "DUT Description"
  # "Tests Included"
  # "Current status:"
  # "Measurement parameters:"
  # "DUT & Test Description:"
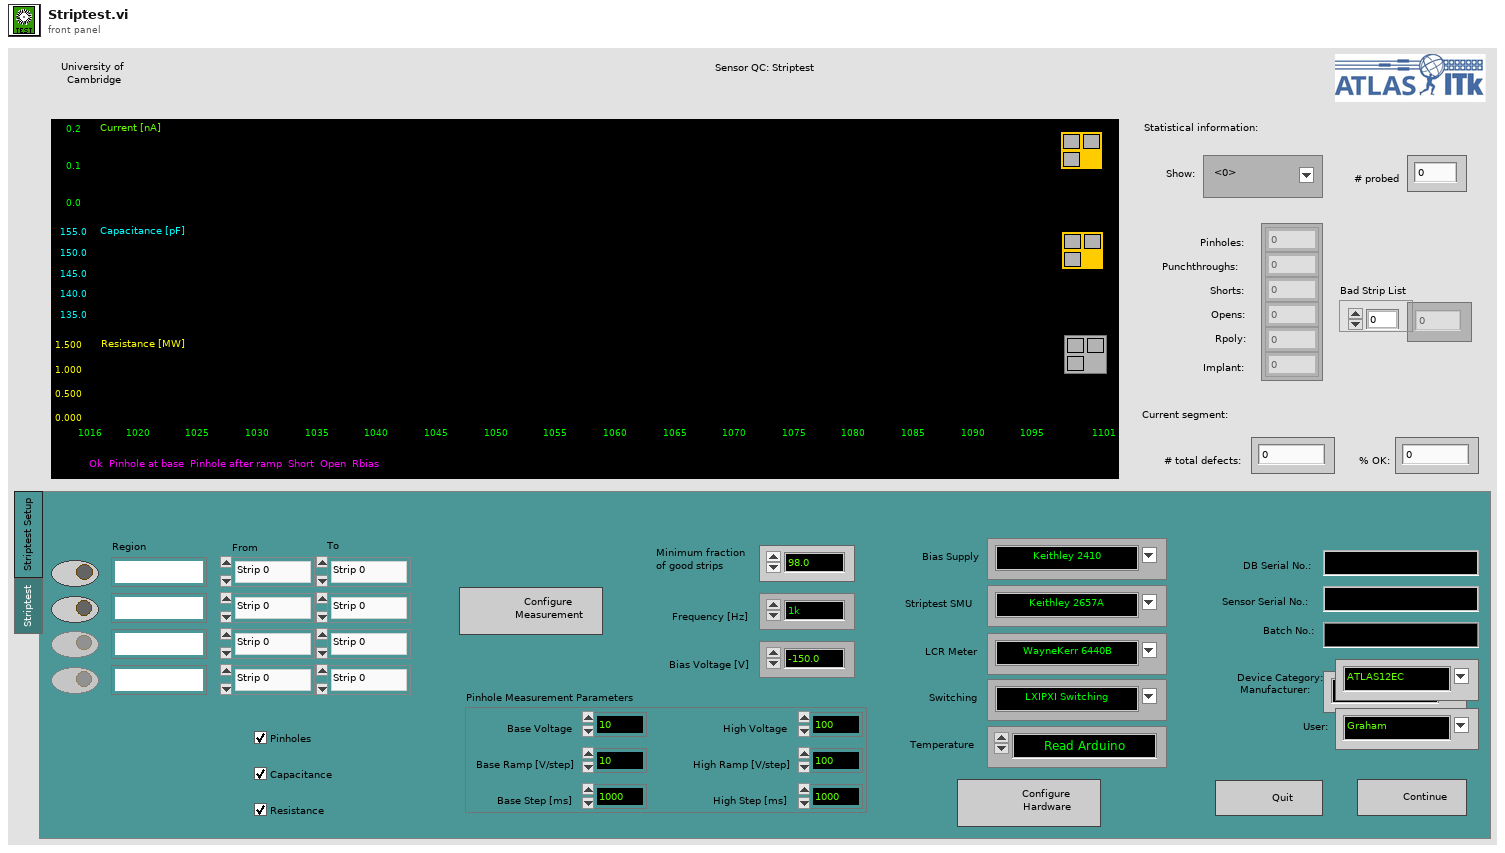
[diagram p1: front panel]
types:
  T1 = cluster{"Base Voltage":dbl, "Base Ramp [V/step]":dbl, "Base Step [ms]":i32, "High Voltage":dbl, "High Ramp [V/step]":dbl, "High Step [ms]":i32}
  T2 = cluster{"Current [nA]":dbl, "Ccoupl Lo [pF/cm]":dbl, "Ccoupl Hi [pF/cm]":dbl, "Rbias Lo [MW]":dbl, "Rbias Hi [MW]":dbl}
  T3 = cluster{"Time Array":string[], "Temperature Array [°C]":dbl[], "Humidity Array [RH %]":dbl[]}
  T4 = enum16{"Supply", "LCR", "Multimeter", "Switching"}
  T5 = enum16{"Reset", "Ground", "Striptest Bias", "Striptest SMU", "Striptest LCR", "IV", "CV", "Interstrip Cap", "Interstrip Res"}
  T6 = enum16{"Reference measurement", "Baseline correcetion 10V", "Baseline correcetion 100V", "Nothing"}
  T7 = enum16{"Reset", "Read Array", "Read Element", "Write Element", "Write Array", "Add Element", "Add Array"}
  T8 = cluster{"Bias Supply":refnum<class "SupplyControl.lvclass">, "SMU":refnum<class "SupplyControl.lvclass">, "LCR":refnum<class "LCRControl.lvclass">, "Probe Card Channels":i32, "Bias Voltage [V]":dbl, "First strip":i32, "Last strip":i32, "Base Voltage [V]":dbl, "Base Ramp Step [V]":dbl, "Base Ramp Interval [ms]":u32, "High Voltage [V]":dbl, "High Ramp Step [V]":dbl, "High Ramp Interval [ms]":u32, "AC frequency [Hz]":i32, "AC amplitude [V]":dbl, "RC Configuration":u16, "Single Needle":bool, "Temperature Readout":enum16{"Read Arduino", "Enter manually"}, "Arduino":refnum<class "ArduinoControl.lvclass">, "Fraction of good strips [%]":dbl, "ProbeStation":refnum<class "ProbeStationControl.lvclass">, "Switching":refnum<class "Switching.lvclass">, "Matrix used?":bool, "Matrix X Channels":cluster{"Bias Supply / SMU LO":i32, "Bias Supply / SMU HI":i32, "CV Box LO":i32, "CV Box HI":i32, "CV Box LO IN":i32, "CV Box HI IN":i32, "Volt meter LO":i32, "Volt meter HI":i32, "Mux1 C1":i32, "Mux1 C2":i32, "Mux2 C1":i32, "Mux2 C2":i32}, "Pinholes Y/N":bool, "Capacitance Y/N":bool, "Resistance Y/N":bool, "Bias Supply Name":string, "SMU Name":string, "LCR Name":string}
  T9 = cluster{"Strip Number OUT":i32, "X0":i32, "Y0":i32, "X1":i32, "Y1":i32, "Xref":dbl, "Yref":dbl, "ProbePlan type":u32, "Inner pads offset":ext, "Outer pads offset":ext, "l_inner":ext, "l_outer":ext, "strip numbering":u16, "Device Orientation":ext, "Stagger offset":i32, "Yoffset":dbl, "Strip pitch":dbl, "Fiducail separation":dbl, "Radius":ext, "Relative strip angles":dbl, "Probeplan description":string, "ProbePlan array":cluster{"Region":string, "ProbePoints":cluster{"X":dbl, "Y":dbl, "Label":string, "CardViable?":bool}[]}[], "Test ProbePoints":cluster{"Regions Enabled":bool[], "From index":u32[], "To index":u32[]}}
  T10 = cluster{"Sensor Serial No.:":string, "Wafer Serial No.:":string, "Batch:":string, "Manufacturer:":string, "Device Category:":string, "Database Serial No.:":string, "Date Initiated:":string, "Time Initiated:":string, "Test":string, "Instruments used:":string, "Probeplan used:":string, "End of Run comment:":string, "User:":string}
  T11 = cluster{"Region":string, "ProbePoints":cluster{"X":dbl, "Y":dbl, "Label":string, "CardViable?":bool}[]}[]
  T12 = cluster{"X":dbl, "Y":dbl, "Label":string, "CardViable?":bool}[]
  T13 = cluster{"Institute":string, "Manufacturers":string[], "Devices":string[], "Serialnumbers Lookup DB":string, "Data directory":string, "Backup & screenshot directory":string, "List of known users":string[], "Measurement switch not used":bool, "Measurement Switch":string, "DUT Switch":string}
  T14 = cluster{"VISA address":refnum<visa-resource-name>, "T sensor":enum16{"SHT", "DS"}, "Arduino":refnum<class "ArduinoControl.lvclass">}
  T15 = cluster{"X":dbl, "Y":dbl, "Label":string, "CardViable?":bool}
  T16 = cluster{"pass Rate in %":dbl, "Bad channel list":i32[], "No of bad strips":i32, "Defect description list":i32[], "Number of defects per category":i32[], "Defect lists":string[], "No of channels":i32, "Defect Flag array OUT":i32[][]}
  T17 = cluster{"Hi Cap":dbl, "Lo Cap":dbl, "Current threshold":dbl, "Lo R":dbl, "Hi R":dbl}
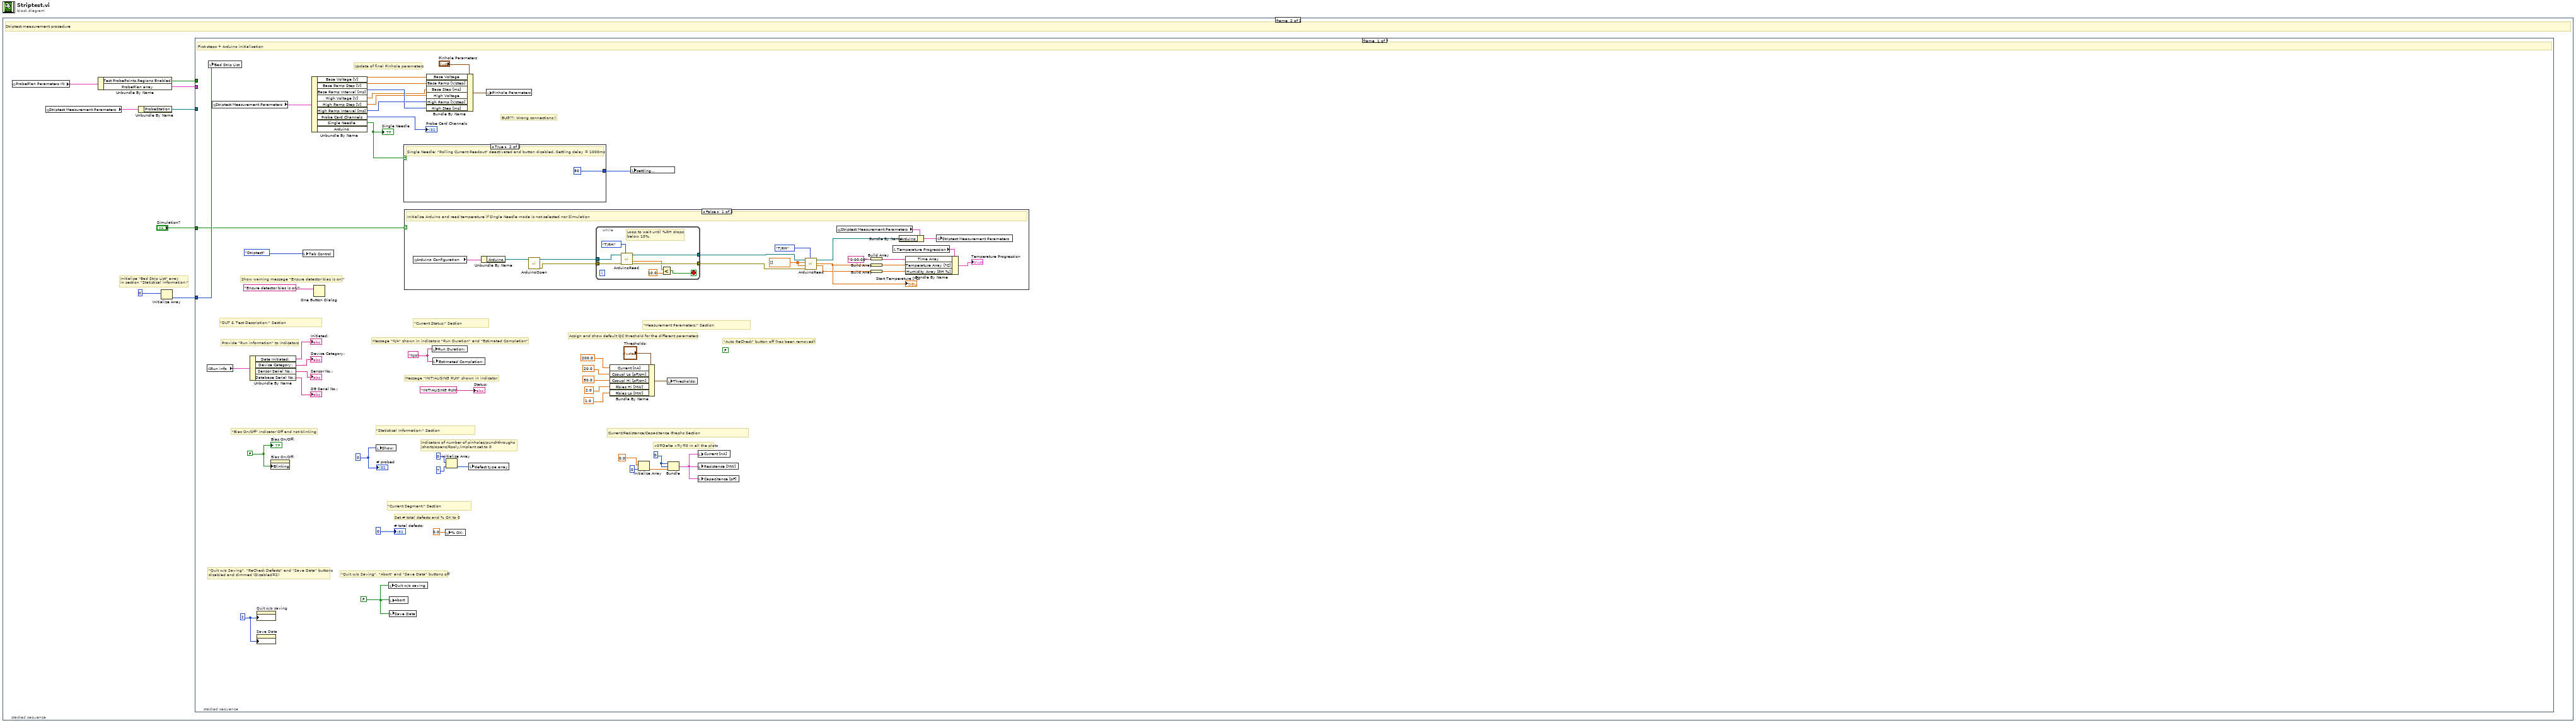
[diagram p0: block diagram]
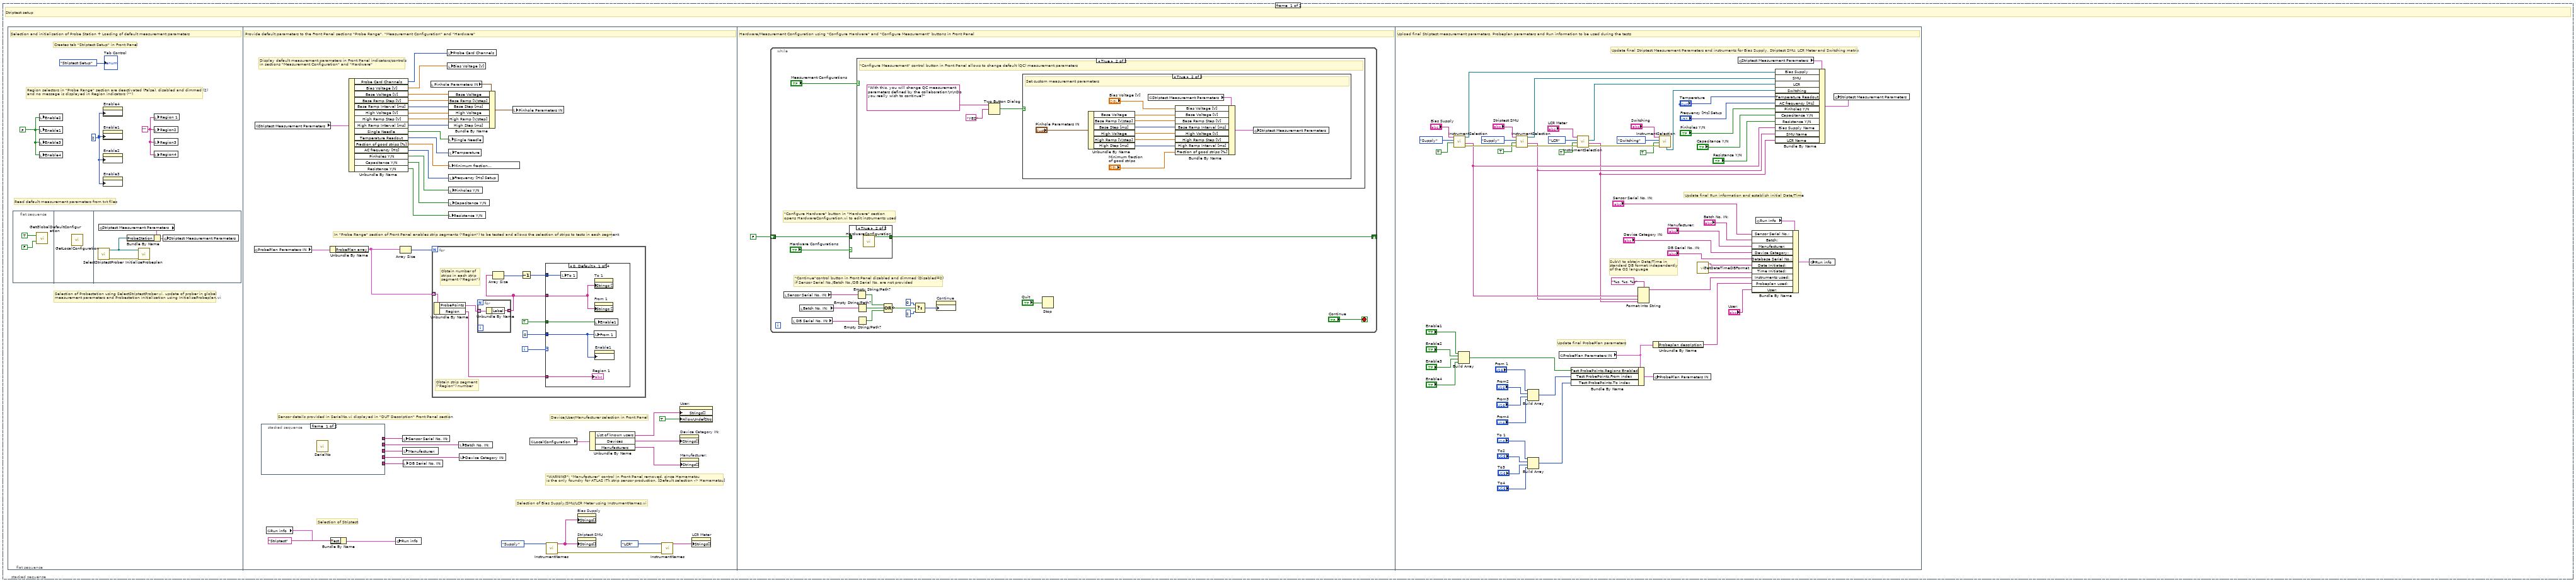
[diagram p2: hidden frame]
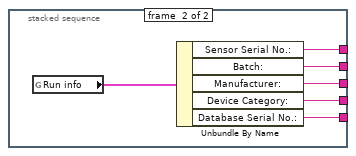
[diagram p3: hidden frame]
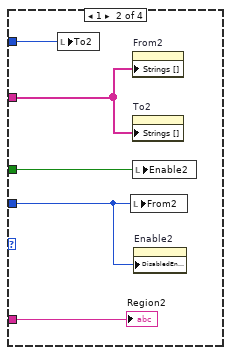
[diagram p4: hidden frame]
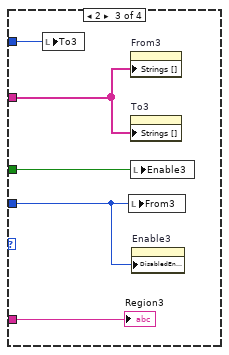
[diagram p5: hidden frame]
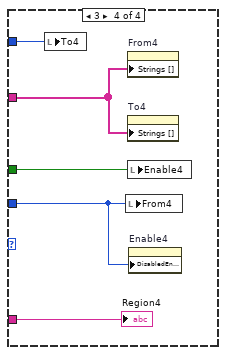
[diagram p6: hidden frame]
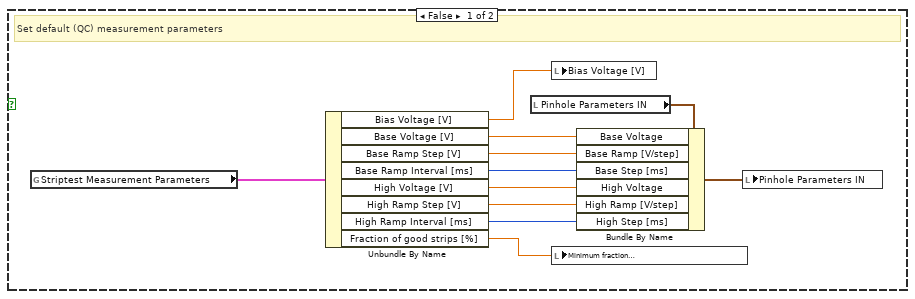
[diagram p8: hidden frame]
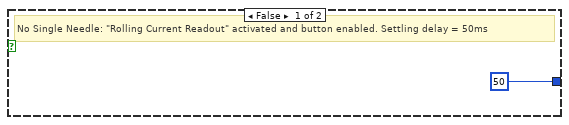
[diagram p10: hidden frame]
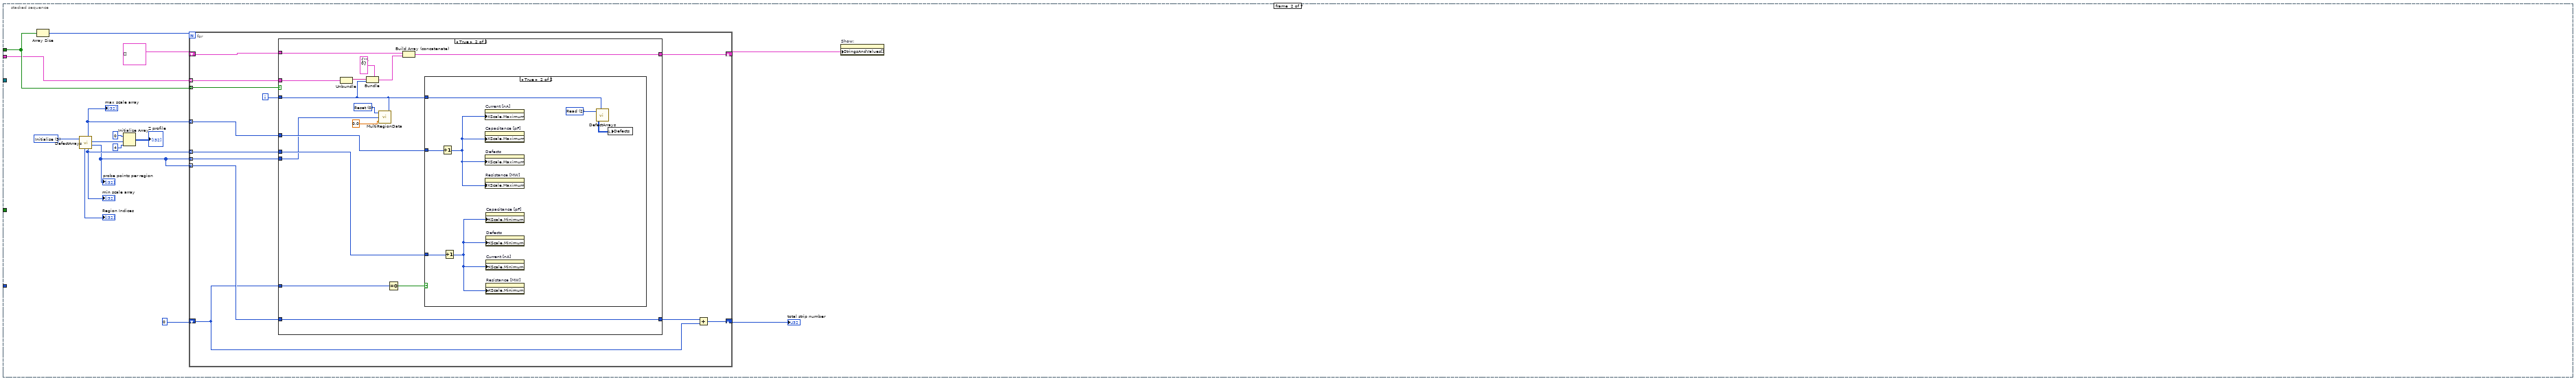
[diagram p12: hidden frame]
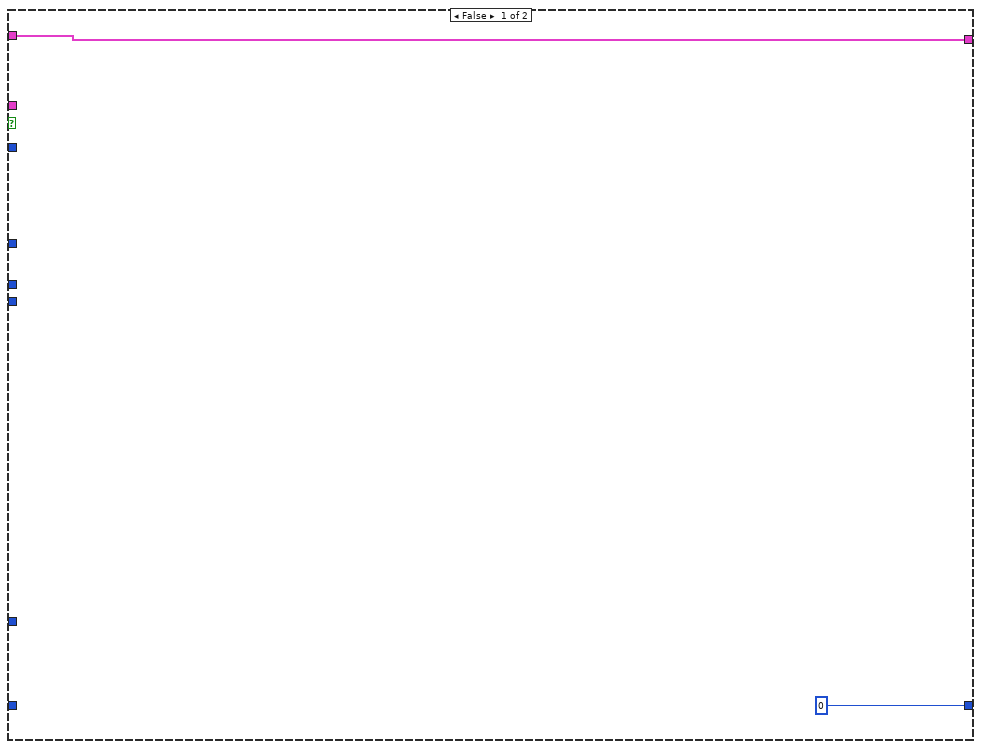
[diagram p13: hidden frame]
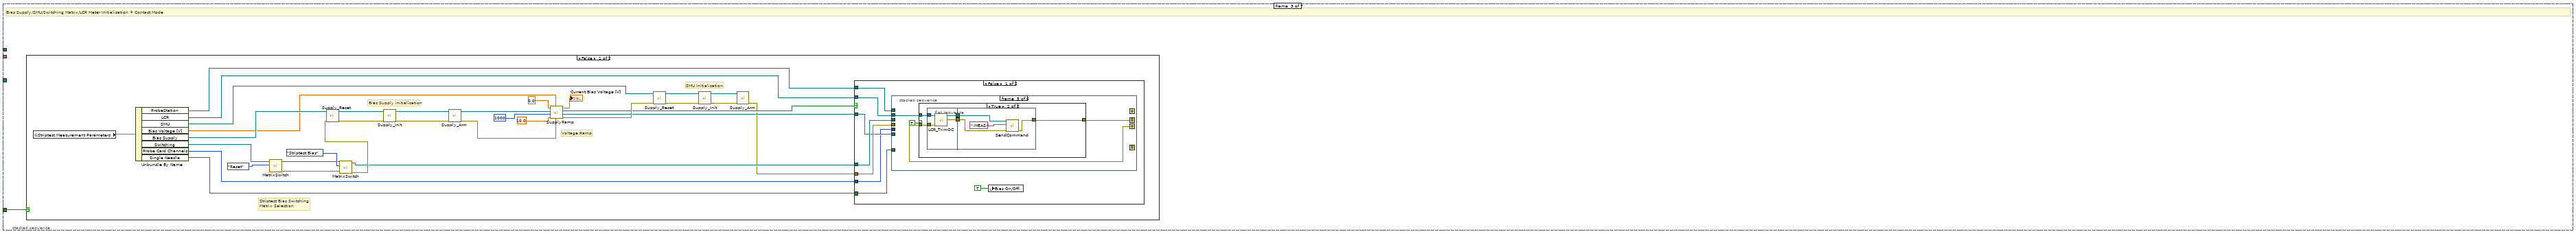
[diagram p15: hidden frame]
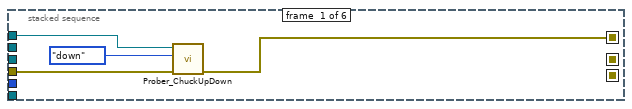
[diagram p16: hidden frame]
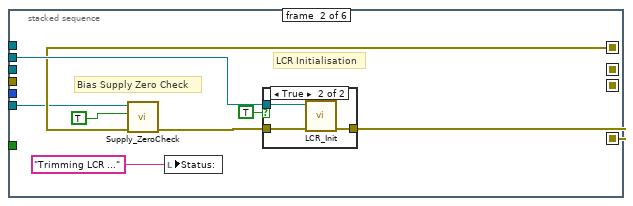
[diagram p17: hidden frame]
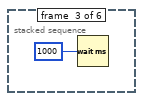
[diagram p19: hidden frame]
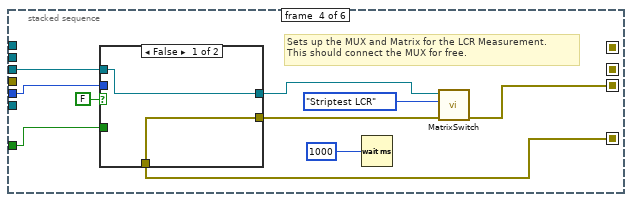
[diagram p20: hidden frame]
diagram:
  n1 = stacked-sequence {
    frame #0 {
      # "Striptest setup"
      n2 = flat-sequence {
        frame #0 {
          w2 = ""
          w3 = 2
          w4 = FALSE
          # "Creates tab \"Striptest Setup\" in Front Panel"
          # "Selection of Probestation using SelectStriptestProber.vi, update of prober in global\nmeasurement parameters and Probestation initialisation using InitialiseProbeplan.vi"
          # "Read default measurement parameters from txt files"
          # "Region selectors in \"Probe Range\" section are deactivated (False), disabled and dimmed (2)\nand no message is displayed in Region indicators (\"\")"
          # "Selection and initialisation of Probe Station + Loading of default measurement parameters"
          n3 = flat-sequence {
            frame #0 {
              n4 = call "GetGlobalDefaultConfiguration.vi"("DO NOT override instruments"=FALSE, "Read defaults?"=TRUE) -> ()  [unwired: 1 in, 1 out]
            }
            frame #1 {
              n5 = call "GetLocalConfiguration.vi"() -> ()  [unwired: 3 in, 1 out]
            }
            frame #2 {
              n6 = call "SelectStriptestProber.vi"() -> ("error out"=w10:errorcluster, "ProbeStationControl out"=w9:refnum<class "ProbeStationControl.lvclass">)  [unwired: 10 in]
              n7 = global read "QC_MeasurementSetup.vi" "Striptest Measurement Parameters"() -> (w7:T8)
              n8 = Bundle By Name(cluster=w7, "ProbeStation"=w9) -> (w8:T8)
              n9 = call "InitialiseProbeplan.vi"("error in (no error)"=w10, "ProbeStationControl in"=w9) -> ()  [unwired: 8 in, 2 out]
              n10 = global write "QC_MeasurementSetup.vi" "Striptest Measurement Parameters"(w8) -> ()
            }
          }
          n11 = local write "Enable2"(w4) -> ()
          n12 = local write "Enable1"(w4) -> ()
          n13 = local write "Enable3"(w4) -> ()
          n14 = local write "Enable4"(w4) -> ()
          n15 = property on="Enable4" class="Bool (strict)"("DisabledEnum"=w3) -> ()  [unwired: 2 in, 2 out]
          n16 = property on="Enable1" class="Bool (strict)"("DisabledEnum"=w3) -> ()  [unwired: 2 in, 2 out]
          n17 = property on="Enable2" class="Bool (strict)"("DisabledEnum"=w3) -> ()  [unwired: 2 in, 2 out]
          n18 = property on="Enable3" class="Bool (strict)"("DisabledEnum"=w3) -> ()  [unwired: 2 in, 2 out]
          n19 = local write "Region 1"(w2) -> ()
          n20 = local write "Region2"(w2) -> ()
          n21 = local write "Region3"(w2) -> ()
          n22 = local write "Region4"(w2) -> ()
          "Tab Control" <- enum32{"Striptest Setup", "Striptest"}."Striptest Setup" ("Tab Control")
        }
        frame #1 {
          # "In \"Probe Range\" section of Front Panel enables strip segments (\"Region\") to be tested and allows the selection of strips to tests in each segment"
          # "Display default measurement parameters in Front Panel indicators/controls\nin sections \"Measurement Configuration\" and \"Hardware\""
          # "*WARNING*: \"Manufacturer\" control in Front Panel removed, since Hamamatsu \nis the only foundry for ATLAS ITk strip sensor production. [Default selection -> Hamamatsu]"
          # "Device/User/Manufacturer selection in Front Panel"
          # "Selection of Bias Supply/SMU/LCR Meter using InstrumentNames.vi"
          # "Selection of Striptest"
          # "Sensor details provided in SerialNo.vi displayed in \"DUT Description\" Front Panel section"
          # "Provide default parameters to the Front Panel sections \"Probe Range\", \"Measurement Configuration\" and \"Hardware\""
          n23 = global read "ProbePlanParams.vi" "ProbePlan Parameters IN"() -> (w49:T9)
          n24 = global read "QC_MeasurementSetup.vi" "Striptest Measurement Parameters"() -> (w36:T8)
          n25 = stacked-sequence {
            tunnel: [_ w55] -> w14
            tunnel: [_ w54] -> w15
            tunnel: [_ w53] -> w16
            tunnel: [_ w52] -> w17
            tunnel: [_ w50] -> w18
            frame #0 {
              n26 = call "SerialNo.vi"() -> ()  [unwired: 5 in, 1 out]
            }
            frame #1 {
              n27 = global read "QC_RunInformation.vi" "Run info"() -> (w51:T10)
              n28 = Unbundle By Name(w51) -> ("Sensor Serial No.:"=w55:string, "Batch:"=w54:string, "Manufacturer:"=w53:string, "Device Category:"=w52:string, "Database Serial No.:"=w50:string)
            }
          }
          n29 = global read "QC_RunInformation.vi" "Run info"() -> (w11:T10)
          n30 = Unbundle By Name(w49) -> ("ProbePlan array"=w48:T11)
          n31 = Bundle By Name(cluster=w11, "Test"="Striptest") -> (w41:T10)
          n32 = Unbundle By Name(w36) -> ("Probe Card Channels"=w35:i32, "Bias Voltage [V]"=w26:dbl, "Base Voltage [V]"=w32:dbl, "Base Ramp Step [V]"=w31:dbl, "Base Ramp Interval [ms]"=w30:u32, "High Voltage [V]"=w29:dbl, "High Ramp Step [V]"=w28:dbl, "High Ramp Interval [ms]"=w27:u32, "Single Needle"=w25:bool, "Temperature Readout"=w24:enum16{"Read Arduino", "Enter manually"}, "Fraction of good strips [%]"=w23:dbl, "AC frequency [Hz]"=w22:i32, "Pinholes Y/N"=w21:bool, "Capacitance Y/N"=w20:bool, "Resistance Y/N"=w19:bool)
          n33 = global write "QC_RunInformation.vi" "Run info"(w41) -> ()
          n34 = Array Size(array=w48) -> (size(s)=w47:i32)
          n35 = local write "Sensor Serial No. IN:"(w14) -> ()
          n36 = local write "Manufacturer:"(w16) -> ()
          n37 = local write "DB Serial No. IN:"(w18) -> ()
          n38 = local read "Pinhole Parameters IN"() -> (w34:T1)
          n39 = for {
            N: w47 -> [_]
            tunnel: w48 -> [w59] mode=indexing
            i -> [w64]
            # "Obtain strip segment \n(\"Region\") number"
            # "Obtain number of\nstrips in each strip\nsegment (\"Region\")"
            n40 = Unbundle By Name(w59) -> ("ProbePoints"=w57:T12, "Region"=w56:string)
            n41 = for {
              tunnel: w57 -> [w66] mode=indexing
              tunnel: [w65] -> w58 mode=indexing
              n42 = Unbundle By Name(w66) -> ("Label"=w65:string)
            }
            n43 = Array Size(array=w58) -> (size(s)=w61:i32)
            n44 = Decrement(x=w61) -> (x-1=w60:i32)
            n45 = case shown="0, Default" w64 {
              tunnel: TRUE -> [w71 w75 w81 w86]
              tunnel: 0 -> [w67 w73 w77 w83]
              tunnel: w56 -> [w69 w74 w79 w84]
              tunnel: w58 -> [w68 w72 w78 w82]
              tunnel: w60 -> [w70 w76 w80 w85]
              frame 0, Default {
                n46 = local write "To 1"(w70) -> ()
                n47 = local write "From 1"(w67) -> ()
                n48 = property on="To 1" class="Ring (strict)"("Strings []"=w68) -> ()  [unwired: 2 in, 2 out]
                n49 = property on="From 1" class="Ring (strict)"("Strings []"=w68) -> ()  [unwired: 2 in, 2 out]
                n50 = local write "Enable1"(w71) -> ()
                n51 = property on="Enable1" class="Bool (strict)"("DisabledEnum"=w67) -> ()  [unwired: 2 in, 2 out]
                "Region 1" <- w69
              }
              frame 1 {
                n52 = local write "To2"(w76) -> ()
                n53 = local write "From2"(w73) -> ()
                n54 = property on="From2" class="Ring (strict)"("Strings []"=w72) -> ()  [unwired: 2 in, 2 out]
                n55 = property on="To2" class="Ring (strict)"("Strings []"=w72) -> ()  [unwired: 2 in, 2 out]
                n56 = local write "Enable2"(w75) -> ()
                n57 = property on="Enable2" class="Bool (strict)"("DisabledEnum"=w73) -> ()  [unwired: 2 in, 2 out]
                "Region2" <- w74
              }
              frame 2 {
                n58 = local write "To3"(w80) -> ()
                n59 = local write "From3"(w77) -> ()
                n60 = property on="From3" class="Ring (strict)"("Strings []"=w78) -> ()  [unwired: 2 in, 2 out]
                n61 = property on="To3" class="Ring (strict)"("Strings []"=w78) -> ()  [unwired: 2 in, 2 out]
                n62 = local write "Enable3"(w81) -> ()
                n63 = property on="Enable3" class="Bool (strict)"("DisabledEnum"=w77) -> ()  [unwired: 2 in, 2 out]
                "Region3" <- w79
              }
              frame 3 {
                n64 = local write "To4"(w85) -> ()
                n65 = local write "From4"(w83) -> ()
                n66 = property on="From4" class="Ring (strict)"("Strings []"=w82) -> ()  [unwired: 2 in, 2 out]
                n67 = property on="To4" class="Ring (strict)"("Strings []"=w82) -> ()  [unwired: 2 in, 2 out]
                n68 = local write "Enable4"(w86) -> ()
                n69 = property on="Enable4" class="Bool (strict)"("DisabledEnum"=w83) -> ()  [unwired: 2 in, 2 out]
                "Region4" <- w84
              }
            }
          }
          n70 = local write "Probe Card Channels"(w35) -> ()
          n71 = local write "Bias Voltage [V]"(w26) -> ()
          n72 = Bundle By Name(cluster=w34, "Base Voltage"=w32, "Base Ramp [V/step]"=w31, "Base Step [ms]"=w30, "High Voltage"=w29, "High Ramp [V/step]"=w28, "High Step [ms]"=w27) -> (w33:T1)
          n73 = local write "Single Needle"(w25) -> ()
          n74 = local write "Minimum fraction\nof good strips"(w23) -> ()
          n75 = local write "Resistance Y/N"(w19) -> ()
          n76 = local write "Temperature"(w24) -> ()
          n77 = local write "Frequency [Hz] Setup"(w22) -> ()
          n78 = local write "Pinholes Y/N"(w21) -> ()
          n79 = local write "Capacitance Y/N"(w20) -> ()
          n80 = local write "Batch No. IN:"(w15) -> ()
          n81 = local write "Device Category IN:"(w17) -> ()
          n82 = local write "Pinhole Parameters IN"(w33) -> ()
          n83 = global read "QC_RunInformation.vi" "LocalConfiguration"() -> (w39:T13)
          n84 = call "InstrumentNames.vi"("Instrument type"=T4."Supply") -> ("error out"=w43:errorcluster, "Instrument names"=w45:string[])  [unwired: 9 in]
          n85 = property on="Bias Supply" class="CmbBox"("Strings[]"=w45) -> ()  [unwired: 2 in, 2 out]
          n86 = property on="Striptest SMU" class="CmbBox"("Strings[]"=w45) -> ()  [unwired: 2 in, 2 out]
          n87 = Unbundle By Name(w39) -> ("List of known users"=w37:string[], "Devices"=w13:string[], "Manufacturers"=w12:string[])
          n88 = call "InstrumentNames.vi"("error in (no error)"=w43, "Instrument type"=T4."LCR") -> ("Instrument names"=w42:string[])  [unwired: 8 in, 1 out]
          n89 = property on="User:" class="CmbBox"("Strings[]"=w37, "AllowUndefStrs"=TRUE) -> ()  [unwired: 2 in, 2 out]
          n90 = property on="Device Category IN:" class="CmbBox"("Strings[]"=w13) -> ()  [unwired: 2 in, 2 out]
          n91 = property on="Manufacturer:" class="CmbBox"("Strings[]"=w12) -> ()  [unwired: 2 in, 2 out]
          n92 = property on="LCR Meter" class="CmbBox"("Strings[]"=w42) -> ()  [unwired: 2 in, 2 out]
        }
        frame #2 {
          # "Hardware/Measurement Configuration using \"Configure Hardware\" and \"Configure Measurement\" buttons in Front Panel"
          n93 = while {
            shift-right: [w90] -> _
            shift-left: FALSE -> [w92]
            stop <- "Continue" stop-if-true
            # "\"Continue\"control button in Front Panel disabled and dimmed (Disabled=2) \nif Sensor Serial No./Batch No./DB Serial No. are not provided"
            # "\"Configure Hardware\" button in \"Hardware\" section\nopens HardwareConfiguration.vi to edit instruments used"
            n94 = local read "Sensor Serial No. IN:"() -> (w98:string)
            n95 = local read "DB Serial No. IN:"() -> (w96:string)
            n96 = local read "Batch No. IN:"() -> (w97:string)
            n97 = case shown="True" "Hardware Configurations" {
              tunnel: [w129 w130] -> w90
              tunnel: w92 -> [w129 _]
              frame False {
              }
              frame True {
                n98 = call "HardwareConfiguration.vi"() -> ("configured?"=w130:bool)  [unwired: 11 in]
              }
            }
            n99 = Empty String/Path?(string/path=w98) -> (empty?=w95:bool)
            n100 = Empty String/Path?(string/path=w97) -> (empty?=w94:bool)
            n101 = Empty String/Path?(string/path=w96) -> (empty?=w93:bool)
            n102 = case shown="True" "Measurement Configurations" {
              frame False {
              }
              frame True {
                # "\"Configure Measurement\" control button in Front Panel allows to change default (QC) measurement parameters"
                n103 = Two Button Dialog(message="With this, you will change QC measurement parameters defined by the collaboration!\n\nDo you really wish to continue?", 2:"YES") -> (T button?=w104:bool)  [unwired: 1 in]
                n104 = case shown="True" w104 {
                  frame False {
                    # "Set default (QC) measurement parameters"
                    n105 = global read "QC_MeasurementSetup.vi" "Striptest Measurement Parameters"() -> (w117:T8)
                    n106 = Unbundle By Name(w117) -> ("Bias Voltage [V]"=w107:dbl, "Base Voltage [V]"=w114:dbl, "Base Ramp Step [V]"=w113:dbl, "Base Ramp Interval [ms]"=w112:u32, "High Voltage [V]"=w111:dbl, "High Ramp Step [V]"=w110:dbl, "High Ramp Interval [ms]"=w109:u32, "Fraction of good strips [%]"=w108:dbl)
                    n107 = local read "Pinhole Parameters IN"() -> (w116:T1)
                    n108 = local write "Bias Voltage [V]"(w107) -> ()
                    n109 = local write "Minimum fraction\nof good strips"(w108) -> ()
                    n110 = Bundle By Name(cluster=w116, "Base Voltage"=w114, "Base Ramp [V/step]"=w113, "Base Step [ms]"=w112, "High Voltage"=w111, "High Ramp [V/step]"=w110, "High Step [ms]"=w109) -> (w115:T1)
                    n111 = local write "Pinhole Parameters IN"(w115) -> ()
                  }
                  frame True {
                    # "Set custom measurement parameters"
                    n112 = Unbundle By Name("Pinhole Parameters IN") -> ("Base Voltage"=w124:dbl, "Base Ramp [V/step]"=w123:dbl, "Base Step [ms]"=w122:i32, "High Voltage"=w121:dbl, "High Ramp [V/step]"=w120:dbl, "High Step [ms]"=w119:i32)
                    n113 = global read "QC_MeasurementSetup.vi" "Striptest Measurement Parameters"() -> (w128:T8)
                    n114 = Bundle By Name(cluster=w128, "Bias Voltage [V]"="Bias Voltage [V]", "Base Voltage [V]"=w124, "Base Ramp Step [V]"=w123, "Base Ramp Interval [ms]"=w122, "High Voltage [V]"=w121, "High Ramp Step [V]"=w120, "High Ramp Interval [ms]"=w119, "Fraction of good strips [%]"="Minimum fraction\nof good strips") -> (w127:T8)
                    n115 = global write "QC_MeasurementSetup.vi" "Striptest Measurement Parameters"(w127) -> ()
                  }
                }
              }
            }
            n116 = Compound Arithmetic op=OR(w95, w94, w93) -> (invert w99:bool)
            n117 = Select(t=0, s=w99, f=2) -> (s? t:f=w89:i32)
            n118 = property on="Continue" class="Bool"("DisabledEnum"=w89) -> ()  [unwired: 2 in, 2 out]
            n119 = Stop(stop? (T)="Quit") -> ()
          }
        }
        frame #3 {
          # "SubVI to obtain Date/Time in\nstandard DB format independently\nof the OS language"
          # "Update final Striptest Measurement Parameters and instruments for Bias Supply, Striptest SMU, LCR Meter and Switching matrix"
          # "Update final ProbePlan parameters"
          # "Update final Run information and establish initial Date/Time"
          # "Upload final Striptest measurement parameters, Probeplan parameters and Run information to be used during the tests"
          n120 = call "InstrumentSelection.vi"("Verify GPIB address"=TRUE, "Instrument type"=T4."Supply", "Instrument name IN"="Bias Supply") -> ("error out"=w166:errorcluster, "Instrument name OUT"=w135:string, "Supply"=w161:refnum<class "SupplyControl.lvclass">)  [unwired: 3 in, 3 out]
          n121 = Build Array("Enable1", "Enable2", "Enable3", "Enable4") -> (w187:bool[])
          n122 = call "InstrumentSelection.vi"("error in (no error)"=w166, "Verify GPIB address"=TRUE, "Instrument type"=T4."Supply", "Instrument name IN"="Striptest SMU") -> ("error out"=w154:errorcluster, "Instrument name OUT"=w134:string, "Supply"=w158:refnum<class "SupplyControl.lvclass">)  [unwired: 2 in, 3 out]
          n123 = Build Array("From 1", "From2", "From3", "From4") -> (w186:u16[])
          n124 = Build Array("To 1", "To2", "To3", "To4") -> (w185:u16[])
          n125 = global read "ProbePlanParams.vi" "ProbePlan Parameters IN"() -> (w189:T9)
          n126 = Bundle By Name(cluster=w189, "Test ProbePoints.Regions Enabled"=w187, "Test ProbePoints.From index"=w186, "Test ProbePoints.To index"=w185) -> (w188:T9)
          n127 = call "InstrumentSelection.vi"("error in (no error)"=w154, "Verify GPIB address"=TRUE, "Instrument type"=T4."LCR", "Instrument name IN"="LCR Meter") -> ("error out"=w155:errorcluster, "Instrument name OUT"=w133:string, "LCR"=w157:refnum<class "LCRControl.lvclass">)  [unwired: 2 in, 3 out]
          n128 = Format Into String(format string="%s, %s, %s", w135, w134, w133) -> (resulting string=w145:string)  [unwired: 2 in, 1 out]
          n129 = Unbundle By Name(w189) -> ("Probeplan description"=w149:string)
          n130 = global write "ProbePlanParams.vi" "ProbePlan Parameters IN"(w188) -> ()
          n131 = call "InstrumentSelection.vi"("error in (no error)"=w155, "Verify GPIB address"=TRUE, "Instrument type"=T4."Switching", "Instrument name IN"="Switching") -> ("Switching"=w156:refnum<class "Switching.lvclass">)  [unwired: 2 in, 5 out]
          n132 = call "GetDateTimeDBFormat.vi"() -> ("Time in 24h format, e.g. 13:40:54"=w131:string, "Abbreviated Date, e.g. 13 Nov 2020"=w132:string)  [unwired: 10 in]
          n133 = global read "QC_MeasurementSetup.vi" "Striptest Measurement Parameters"() -> (w163:T8)
          n134 = global read "QC_RunInformation.vi" "Run info"() -> (w164:T10)
          n135 = Bundle By Name(cluster=w164, "Sensor Serial No.:"="Sensor Serial No. IN:", "Batch:"="Batch No. IN:", "Manufacturer:"="Manufacturer:", "Device Category:"="Device Category IN:", "Database Serial No.:"="DB Serial No. IN:", "Date Initiated:"=w132, "Time Initiated:"=w131, "Instruments used:"=w145, "Probeplan used:"=w149, "User:"="User:") -> (w172:T10)
          n136 = Bundle By Name(cluster=w163, "Bias Supply"=w161, "SMU"=w158, "LCR"=w157, "Switching"=w156, "Temperature Readout"="Temperature", "AC frequency [Hz]"="Frequency [Hz] Setup", "Pinholes Y/N"="Pinholes Y/N", "Capacitance Y/N"="Capacitance Y/N", "Resistance Y/N"="Resistance Y/N", "Bias Supply Name"=w135, "SMU Name"=w134, "LCR Name"=w133) -> (w162:T8)
          n137 = global write "QC_RunInformation.vi" "Run info"(w172) -> ()
          n138 = global write "QC_MeasurementSetup.vi" "Striptest Measurement Parameters"(w162) -> ()
        }
      }
    }
    frame #1 {
      # "Initialise \"Bad Strip List\" array\nin section \"Statistical information:\""
      # "Striptest measurement procedure"
      n139 = global read "ProbePlanParams.vi" "ProbePlan Parameters IN"() -> (w197:T9)
      n140 = global read "QC_MeasurementSetup.vi" "Striptest Measurement Parameters"() -> (w190:T8)
      n141 = Unbundle By Name(w197) -> ("Test ProbePoints.Regions Enabled"=w193:bool[], "ProbePlan array"=w192:T11)
      n142 = Unbundle By Name(w190) -> ("ProbeStation"=w191:refnum<class "ProbeStationControl.lvclass">)
      n143 = Initialize Array(0) -> (w195:i32[])  [unwired: 1 in]
      n144 = stacked-sequence {
        tunnel: w195 -> [w221 _ _ _ w469 _ _]
        tunnel: "Simulation?" -> [w200 _ w323 w447 _ w1100 w1157]
        tunnel: w193 -> [_ w285 _ _ w472 _ w1156]
        tunnel: w192 -> [_ w284 _ _ w470 _ _]
        tunnel: w191 -> [_ _ _ w445 _ w1099 _]
        frame #0 {
          w201 = FALSE
          (unwired) FALSE
          w202 = 0
          w223 = "N/A"
          w218 = FALSE
          w231 = 2
          w240 = 0
          # "\"Auto ReCheck\" button off (has been removed)"
          # "\"Quit w/o Saving\", \"Abort\" and \"Save Data\" buttons off"
          # "\"Bias On/Off\" indicator Off and not blinking"
          # "\"Measurement Parameters:\" Section"
          # "Assign and show default QC threshold for the different parameters"
          # "Indicators of number of pinholes/punchthroughs\n/shorts/opens/Rpoly/implant set to 0"
          # "Set # total defects and % OK to 0"
          # "Current/Resistance/Capacitance Graphs Section"
          # "\"Current Segment:\" Section"
          # "\"Statistical Information:\" Section"
          # "\"Current Status:\" Section"
          # "\"DUT & Test Description:\" Section"
          # "Show warning message \"Ensure detector bias is on!\""
          # "\"Quit w/o Saving\", \"ReCheck Defects\" and \"Save Data\" buttons\ndisabled and dimmed (Disabled=2)"
          # "Message \"N/A\" shown in indicators \"Run Duration\" and \"Estimated Completion\""
          # "x0=Delta x=y=0 in all the plots"
          # "Message \"INITIALISING RUN\" shown in indicator"
          # "Provide \"Run information\" to indicators"
          # "Update of final Pinhole parameters"
          # "BUG??: Wrong connections!!"
          # "First steps + Arduino initialisation"
          n145 = global read "QC_RunInformation.vi" "Run info"() -> (w238:T10)
          n146 = local write "Bad Strip List"(w221) -> ()
          n147 = global read "QC_MeasurementSetup.vi" "Striptest Measurement Parameters"() -> (w210:T8)
          n148 = Unbundle By Name(w238) -> ("Date Initiated:"=→"Initiated:":string, "Device Category:"=→"Device Category:":string, "Sensor Serial No.:"=→"Sensor No.:":string, "Database Serial No.:"=→"DB Serial No.:":string)
          n149 = property on="Quit w/o saving" class="Bool (strict)"("DisabledEnum"=w231) -> ()  [unwired: 2 in, 2 out]
          n150 = property on="Save Data" class="Bool (strict)"("DisabledEnum"=w231) -> ()  [unwired: 2 in, 2 out]
          n151 = property on="Bias On/Off:" class="Bool (strict)"("Blinking"=w201) -> ()  [unwired: 2 in, 2 out]
          n152 = local write "Tab Control"(enum32{"Striptest Setup", "Striptest"}."Striptest" ("Tab Control")) -> ()
          n153 = Unbundle By Name(w210) -> ("Base Voltage [V]"=w214:dbl, "Base Ramp Step [V]"=w215:dbl, "Base Ramp Interval [ms]"=w206:u32, "High Voltage [V]"=w203:dbl, "High Ramp Step [V]"=w204:dbl, "High Ramp Interval [ms]"=w205:u32, "Probe Card Channels"=→"Probe Card Channels":i32, "Single Needle"=w209:bool)  [unwired: 1 out]
          "Single Needle" <- w209
          n154 = One Button Dialog(message="Ensure detector bias is on!") -> ()  [unwired: 1 in, 1 out]
          n155 = local write "Show:"(w202) -> ()
          n156 = local write "Quit w/o saving"(w218) -> ()
          n157 = local write "Abort"(w218) -> ()
          n158 = local write "Save Data"(w218) -> ()
          n159 = case shown="True" w209 {
            tunnel: [50 50] -> w211
            frame False {
              # "No Single Needle: \"Rolling Current Readout\" activated and button enabled. Settling delay = 50ms"
            }
            frame True {
              # "Single Needle: \"Rolling Current Readout\" deactivated and button disabled. Settling delay = 1000ms"
            }
          }
          n160 = case shown="False" w200 {
            frame False {
              w250 = dbl[] []
              # "Initialise Arduino and read temperature if Single Needle mode is not selected nor Simulation"
              n161 = global read "InstrumentSetup.vi" "Arduino Configuration"() -> (w262:T14)
              n162 = Unbundle By Name(w262) -> ("Arduino"=w255:refnum<class "ArduinoControl.lvclass">)
              n163 = call "ArduinoOpen.vi"("ArduinoControl in"=w255) -> ("error out"=w246:errorcluster, "ArduinoControl out"=w247:refnum<class "ArduinoControl.lvclass">)  [unwired: 9 in]
              n164 = while {
                tunnel: w247 -> [w270]
                tunnel: w246 -> [w269]
                tunnel: [w268] -> w245
                tunnel: [w267] -> w244
                stop <- w263 stop-if-true
                # "Loop to wait until %RH drops\nbelow 10%."
                n165 = call "ArduinoRead.vi"("Arduino function"=enum16{"T/RH", "Interlock", "Edgesense"}."T/RH", "error in (no error)"=w269, "ArduinoControl in"=w270) -> ("error out"=w267:errorcluster, "rel. Humidity [%]"=w265:dbl, "ArduinoControl out"=w268:refnum<class "ArduinoControl.lvclass">)  [unwired: 3 in, 3 out]
                n166 = Less?(x=w265, y=10.0) -> (x < y?=w263:bool)
              }
              n167 = call "ArduinoRead.vi"("Arduino function"=enum16{"T/RH", "Interlock", "Edgesense"}."T/RH", "error in (no error)"=w244, "Humidity IN"=w250, "Temperature IN"=w250, "ArduinoControl in"=w245) -> ("rel. Humidity [%]"=w248:dbl, "Temperature [°C]"=w257:dbl, "ArduinoControl out"=w251:refnum<class "ArduinoControl.lvclass">)  [unwired: 1 in, 3 out]
              "Start Temperature [°C]" <- w257
              n168 = global read "QC_MeasurementSetup.vi" "Striptest Measurement Parameters"() -> (w253:T8)
              n169 = Build Array("0:00:00") -> (w258:string[])
              n170 = Build Array(w257) -> (w256:dbl[])
              n171 = Build Array(w248) -> (w249:dbl[])
              n172 = local read "Temperature Progression"() -> (w261:T3)
              n173 = Bundle By Name(cluster=w253, "Arduino"=w251) -> (w252:T8)
              n174 = Bundle By Name(cluster=w261, "Time Array"=w258, "Temperature Array [°C]"=w256, "Humidity Array [RH %]"=w249) -> (→"Temperature Progression":T3)
              n175 = global write "QC_MeasurementSetup.vi" "Striptest Measurement Parameters"(w252) -> ()
            }
            frame True {
            }
          }
          n176 = Bundle By Name(cluster="Pinhole Parameters", "Base Voltage"=w214, "Base Ramp [V/step]"=w215, "Base Step [ms]"=w203, "High Voltage"=w204, "High Ramp [V/step]"=w205, "High Step [ms]"=w206) -> (w216:T1)
          n177 = local write "Run Duration:"(w223) -> ()
          n178 = local write "Estimated Completion:"(w223) -> ()
          n179 = local write "% OK:"(0.0) -> ()
          n180 = Initialize Array(0, 7 ("Dimension Size")) -> (w219:i32[])
          n181 = local write "defect type array"(w219) -> ()
          n182 = local write "Pinhole Parameters"(w216) -> ()
          n183 = Bundle By Name(cluster="Thresholds:", "Current [nA]"=200.0 ("CapLo"), "Ccoupl Lo [pF/cm]"=20.0 ("CapLo"), "Ccoupl Hi [pF/cm]"=50.0 ("CapHi"), "Rbias Hi [MW]"=2.0 ("Rpolyhi"), "Rbias Lo [MW]"=1.0 ("RpolyLo")) -> (w229:T2)
          n184 = local write "settling\ndelay [ms]"(w211) -> ()
          n185 = Initialize Array(0.0, 0 ("dimension size")) -> (w241:dbl[])
          n186 = local write "Thresholds:"(w229) -> ()
          n187 = Bundle(w240, w240, w241) -> (w239:cluster{i32, i32, dbl[]})  [unwired: 1 in]
          n188 = local write "Current [nA]"(w239) -> ()
          n189 = local write "Resistance [MW]"(w239) -> ()
          n190 = local write "Capacitance [pF]"(w239) -> ()
          "# total defects:" <- 0
          "# probed" <- w202
          "Status:" <- "INITIALISING RUN"
          "Bias On/Off:" <- w201
        }
        frame #1 {
          w280 = u16 3 items=["Nothing", "Write", "Read", "Initialise"] ("action")
          n191 = Array Size(array=w285) -> (size(s)=w286:i32)
          n192 = call "DefectArrays.vi"("action"=w280) -> ("Region Indices"=→"Region Indices":i32[], "To"=w279:i32[], "max. No. of points in region"=w271:i32, "From"=w278:i32[], "No. of points in region"=w273:i32[])  [unwired: 2 in, 3 out]
          "max scale array" <- w279
          "min scale array" <- w278
          "probe points per region" <- w273
          n193 = Initialize Array(0, w271, 4) -> (→"Z profile":i32[][])
          n194 = for {
            N: w286 -> [_]
            tunnel: w285 -> [w298] mode=indexing
            shift-right: [w297] -> w283
            shift-left: cluster{string, i32}[] [] -> [w296]
            tunnel: w284 -> [w295] mode=indexing
            tunnel: w273 -> [w290] mode=indexing
            tunnel: w279 -> [w291] mode=indexing
            tunnel: w278 -> [w288] mode=indexing
            shift-right: [w292] -> w282
            shift-left: 0 -> [w289]
            tunnel: w273 -> [w287] mode=indexing
            i -> [w293]
            n195 = case shown="True" w298 {
              tunnel: w296 -> [w299 w314]
              tunnel: [w299 w313] -> w297
              tunnel: w295 -> [_ w315]
              tunnel: [0 w309] -> w294
              tunnel: w293 -> [_ w304]
              tunnel: w291 -> [_ w311]
              tunnel: w288 -> [_ w310]
              tunnel: w290 -> [_ w309]
              tunnel: w289 -> [_ w308]
              tunnel: w287 -> [_ w302]
              frame False {
              }
              frame True {
                w306 = u32 0 items=["Reset", "Read Array", "Read Element", "Write Element", "Write Array"] ("Action")
                n196 = Unbundle(w315) -> ("Region"=w305:string)  [unwired: 1 out]
                n197 = Bundle(cluster=cluster{string, i32} {"", 0}, w305, w304) -> (w303:cluster{string, i32})
                n198 = call "MultiRegionData.vi"("Action"=w306, "Array Size / Index"=w302, "Data IN"=0.0, "Region index"=w304) -> ()  [unwired: 2 in, 2 out]
                n199 = Equal To 0?(x=w308) -> (x = 0?=w312:bool)
                n200 = Build Array (concatenate)(w314, w303) -> (w313:cluster{string, i32}[])
                n201 = case shown="True" w312 {
                  tunnel: w311 -> [_ w317]
                  tunnel: w310 -> [_ w319]
                  tunnel: w304 -> [_ w320]
                  frame False {
                  }
                  frame True {
                    w322 = u16 2 items=["Nothing", "Write", "Read", "Initialise"] ("action")
                    n202 = Increment(x=w317) -> (x+1=w316:i32)
                    n203 = Increment(x=w319) -> (x+1=w318:i32)
                    n204 = property on="Current [nA]" class="WFGraph (strict)"("XScale.Maximum"=w316) -> ()  [unwired: 2 in, 2 out]
                    n205 = property on="Capacitance [pF]" class="WFGraph (strict)"("XScale.Maximum"=w316) -> ()  [unwired: 2 in, 2 out]
                    n206 = property on="Defects" class="IntGraph (strict)"("XScale.Maximum"=w316) -> ()  [unwired: 2 in, 2 out]
                    n207 = property on="Resistance [MW]" class="WFGraph (strict)"("XScale.Maximum"=w316) -> ()  [unwired: 2 in, 2 out]
                    n208 = property on="Capacitance [pF]" class="WFGraph (strict)"("XScale.Minimum"=w318) -> ()  [unwired: 2 in, 2 out]
                    n209 = property on="Defects" class="IntGraph (strict)"("XScale.Minimum"=w318) -> ()  [unwired: 2 in, 2 out]
                    n210 = property on="Current [nA]" class="WFGraph (strict)"("XScale.Minimum"=w318) -> ()  [unwired: 2 in, 2 out]
                    n211 = property on="Resistance [MW]" class="WFGraph (strict)"("XScale.Minimum"=w318) -> ()  [unwired: 2 in, 2 out]
                    n212 = call "DefectArrays.vi"("action"=w322, "Region Index"=w320) -> ("Defect array OUT"=w321:i32[][])  [unwired: 1 in, 7 out]
                    n213 = local write "Defects"(w321) -> ()
                  }
                }
              }
            }
            n214 = Add(x=w294, y=w289) -> (x+y=w292:i32)
          }
          "total strip number" <- w282
          n215 = property on="Show:" class="Ring (strict)"("StringsAndValues[]"=w283) -> ()  [unwired: 2 in, 2 out]
        }
        frame #2 {
          # "Bias Supply/SMU/Switching Matrix/LCR Meter Initialisation + Contact Mode"
          n216 = case shown="False" w323 {
            frame False {
              # "Voltage Ramp"
              # "Striptest Bias Switching \nMatrix Selection"
              # "SMU Initialisation"
              # "Bias Supply Initialisation"
              n217 = global read "QC_MeasurementSetup.vi" "Striptest Measurement Parameters"() -> (w356:T8)
              n218 = Unbundle By Name(w356) -> ("ProbeStation"=w333:refnum<class "ProbeStationControl.lvclass">, "LCR"=w338:refnum<class "LCRControl.lvclass">, "SMU"=w339:refnum<class "SupplyControl.lvclass">, "Bias Voltage [V]"=w331:dbl, "Bias Supply"=w332:refnum<class "SupplyControl.lvclass">, "Switching"=w329:refnum<class "Switching.lvclass">, "Probe Card Channels"=w336:i32, "Single Needle"=w335:bool)
              n219 = call-dynamic "MatrixSwitch.vi"("Action"=T5."Reset", "Switching in"=w329) -> ("error out"=w327:errorcluster, "Switching out"=w330:refnum<class "Switching.lvclass">)  [unwired: 7 in, 1 out]
              n220 = call-dynamic "MatrixSwitch.vi"("error in (no error)"=w327, "Action"=T5."Striptest Bias", "Switching in"=w330) -> ("error out"=w326:errorcluster, "Switching out"=w325:refnum<class "Switching.lvclass">)  [unwired: 6 in, 1 out]
              n221 = call-dynamic "Supply_Reset.vi"("error in (no error)"=w326, "SupplyControl in"=w332) -> ("error out"=w349:errorcluster, "SupplyControl out"=w352:refnum<class "SupplyControl.lvclass">)  [unwired: 8 in]
              n222 = call-dynamic "Supply_Init.vi"("error in (no error)"=w349, "SupplyControl in"=w352) -> ("error out"=w350:errorcluster, "SupplyControl out"=w351:refnum<class "SupplyControl.lvclass">)  [unwired: 8 in]
              n223 = call-dynamic "Supply_Arm.vi"("error in (no error)"=w350, "SupplyControl in"=w351) -> ("error out"=w347:errorcluster, "SupplyControl out"=w348:refnum<class "SupplyControl.lvclass">)  [unwired: 8 in]
              n224 = call "SupplyRamp.vi"("error in"=w347, "Requested Voltage"=w331, "Step Size"=10.0, "Step Delay"=1000, "Supply IN"=w348, "Starting Voltage"=0.0) -> ("error out"=w346:errorcluster, "Supply OUT"=w337:refnum<class "SupplyControl.lvclass">, "Compliance exceeded"=w340:bool, "Current Voltage"=→"Current Bias Voltage [V]":dbl)  [unwired: 2 in]
              n225 = call-dynamic "Supply_Reset.vi"("error in (no error)"=w346, "SupplyControl in"=w339) -> ("error out"=w344:errorcluster, "SupplyControl out"=w343:refnum<class "SupplyControl.lvclass">)  [unwired: 8 in]
              n226 = call-dynamic "Supply_Init.vi"("error in (no error)"=w344, "SupplyControl in"=w343) -> ("error out"=w345:errorcluster, "SupplyControl out"=w342:refnum<class "SupplyControl.lvclass">)  [unwired: 8 in]
              n227 = call-dynamic "Supply_Arm.vi"("error in (no error)"=w345, "SupplyControl in"=w342) -> ("error out"=w324:errorcluster)  [unwired: 8 in, 1 out]
              n228 = case shown="False" w340 {
                selector: w340 -> [_ w444]
                tunnel: w325 -> [w363 _]
                tunnel: w324 -> [w362 _]
                tunnel: w338 -> [w361 _]
                tunnel: w333 -> [w360 _]
                tunnel: w337 -> [w359 _]
                tunnel: w336 -> [w358 _]
                tunnel: w335 -> [w357 _]
                frame False {
                  n229 = stacked-sequence {
                    seq-local: [w366 _ _ _ _ _] -> [_ w372 _ _ _ _]
                    seq-local: [_ w376 _ _ _ _] -> [_ _ _ w388 _ _]
                    seq-local: [_ _ _ w389 _ _] -> [_ _ _ _ w405 _]
                    seq-local: [_ _ _ _ w403 _] -> [_ _ _ _ _ w424]
                    tunnel: w363 -> [_ _ _ w385 _ w425]
                    tunnel: w362 -> [w367 _ _ _ _ _]
                    tunnel: w361 -> [_ w375 _ _ w404 _]
                    tunnel: w360 -> [w365 _ _ _ _ _]
                    tunnel: w359 -> [_ w370 _ _ _ w426]
                    tunnel: w358 -> [_ _ _ w386 _ w422]
                    tunnel: w357 -> [_ _ _ w387 _ w421]
                    frame #0 {
                      n230 = call-dynamic "Prober_ChuckUpDown.vi"("error in (no error)"=w367, "Direction"=enum16{"up", "down"}."down", "ProbeStationControl in"=w365) -> ("error out"=w366:errorcluster)  [unwired: 6 in, 2 out]
                    }
                    frame #1 {
                      # "Bias Supply Zero Check"
                      # "LCR Initialisation"
                      n231 = call-dynamic "Supply_ZeroCheck.vi"("error in (no error)"=w372, "enable/disable"=TRUE, "SupplyControl in"=w370) -> ("error out"=w371:errorcluster)  [unwired: 7 in, 1 out]
                      n232 = local write "Status:"("Trimming LCR ..." ("STATUS 1")) -> ()
                      n233 = case shown="True" TRUE {
                        tunnel: [w377 w380] -> w376
                        tunnel: w375 -> [_ w379]
                        tunnel: w371 -> [w377 w378]
                        frame False {
                        }
                        frame True {
                          n234 = call-dynamic "LCR_Init.vi"("error in (no error)"=w378, "LCRControl in"=w379) -> ("error out"=w380:errorcluster)  [unwired: 8 in, 1 out]
                        }
                      }
                    }
                    frame #2 {
                      n235 = Wait (ms)(milliseconds to wait=u32 1000) -> ()  [unwired: 1 out]
                    }
                    frame #3 {
                      # "Sets up the MUX and Matrix for the LCR Measurement. \nThis should connect the MUX for free."
                      n236 = case shown="False" FALSE {
                        tunnel: [w392 w400] -> w390
                        tunnel: w388 -> [w392 w399]
                        tunnel: w387 -> [_ w398]
                        tunnel: w386 -> [_ w397]
                        tunnel: w385 -> [w393 w396]
                        tunnel: [w393 w395] -> w384
                        frame False {
                        }
                        frame True {
                          n237 = call-dynamic "MuxCardSwitch.vi"("Instrument"=enum16{"SMU", "LCR"}."LCR", "Single Needle"=w398, "Probe Card Channels"=w397, "error in (no error)"=w399, "Switch to channel"=1, "Switching in"=w396) -> ("error out"=w400:errorcluster, "Switching out"=w395:refnum<class "Switching.lvclass">)  [unwired: 3 in, 1 out]
                        }
                      }
                      n238 = Wait (ms)(milliseconds to wait=1000) -> ()  [unwired: 1 out]
                      n239 = call-dynamic "MatrixSwitch.vi"("error in (no error)"=w390, "Action"=T5."Striptest LCR", "Switching in"=w384) -> ("error out"=w389:errorcluster)  [unwired: 6 in, 2 out]
                    }
                    frame #4 {
                      n240 = case shown="True" TRUE {
                        tunnel: w405 -> [w406 w411]
                        tunnel: w404 -> [_ w410]
                        tunnel: [w406 w409] -> w403
                        frame False {
                        }
                        frame True {
                          n241 = flat-sequence {
                            tunnel: w411 -> [w415]
                            tunnel: w410 -> [w414]
                            tunnel: [w413] -> w408
                            tunnel: [w412] -> w407
                            tunnel: [w416] -> w409
                            tunnel: w408 -> [w419]
                            tunnel: w407 -> [w418]
                            frame #0 {
                              n242 = call-dynamic "LCR_TrimOC.vi"("error in (no error)"=w415, "LCRControl in"=w414) -> ("error out"=w413:errorcluster, "LCRControl out"=w412:refnum<class "LCRControl.lvclass">)  [unwired: 8 in]
                            }
                            frame #1 {
                              n243 = call "SendCommand.vi"("error in (no error)"=w419, "Command string"=":MEAS;", "InstControl in"=w418) -> ("error out"=w416:errorcluster)  [unwired: 7 in, 1 out]
                            }
                          }
                        }
                      }
                    }
                    frame #5 {
                      n244 = call-dynamic "Supply_ZeroCheck.vi"("error in (no error)"=w424, "enable/disable"=TRUE, "SupplyControl in"=w426) -> ("error out"=w423:errorcluster)  [unwired: 7 in, 1 out]
                      n245 = case shown="False" TRUE {
                        tunnel: w425 -> [w433 _]
                        tunnel: w423 -> [w432 _]
                        tunnel: w422 -> [w430 _]
                        tunnel: w421 -> [w429 _]
                        frame False {
                          w438 = u16 0 items=["Open", "Close"] ("Switch action")
                          n246 = call-dynamic "MatrixSwitchSingle.vi"("Switch action"=w438, "error in (no error)"=w432, "Matrix Y"=1, "Matrix X"=3, "Switching in"=w433) -> ("error out"=w435:errorcluster, "Switching out"=w436:refnum<class "Switching.lvclass">)  [unwired: 4 in, 1 out]
                          n247 = call-dynamic "MatrixSwitchSingle.vi"("Switch action"=w438, "error in (no error)"=w435, "Matrix Y"=2, "Matrix X"=4, "Switching in"=w436) -> ("error out"=w434:errorcluster, "Switching out"=w431:refnum<class "Switching.lvclass">)  [unwired: 4 in, 1 out]
                          n248 = call-dynamic "MuxCardSwitch.vi"("Instrument"=enum16{"SMU", "LCR"}."SMU", "Single Needle"=w429, "Probe Card Channels"=w430, "error in (no error)"=w434, "Switch to channel"=-1, "Switching in"=w431) -> ()  [unwired: 3 in, 3 out]
                        }
                        frame True {
                        }
                      }
                    }
                  }
                  n249 = local write "Bias On/Off:"(TRUE ("Bias On?")) -> ()
                }
                frame True {
                  n250 = property on="Bias On/Off:" class="Bool (strict)"("Blinking"=w444) -> ()  [unwired: 2 in, 2 out]
                  n251 = local write "Status:"("Compliance exceeded\nRUN ABORTED") -> ()
                }
              }
            }
            frame True {
            }
          }
        }
        frame #3 {
          # "Here, current is corrected if using a probe card to eliminate discrepancies between needles."
          # "Current Reference Measurement + Correction"
          n252 = property on="Bias On/Off:" class="Bool (strict)"() -> ("Blinking"=w446:bool)  [unwired: 2 in, 2 out]
          n253 = case shown="False" w446 {
            tunnel: w447 -> [w451 _]
            tunnel: w445 -> [w448 _]
            frame False {
              n254 = local read "Single Needle"() -> (w450:bool)
              n255 = property on="Abort" class="Bool (strict)"("DisabledEnum"=0) -> ()  [unwired: 2 in, 2 out]
              n256 = Or(x=w450, y=w451) -> (x .or. y?=w449:bool)
              n257 = case shown="False" w449 {
                tunnel: [w455 FALSE] -> w453
                tunnel: w448 -> [w454 _]
                frame False {
                  n258 = stacked-sequence {
                    tunnel: [_ w464] -> w455
                    tunnel: w454 -> [_ _]
                    frame #0 {
                      n259 = global read "QC_MeasurementSetup.vi" "Striptest Measurement Parameters"() -> (w457:T8)
                      n260 = local write "Status:"("Reference measurement") -> ()
                      n261 = Unbundle By Name(w457) -> ("Switching"=w458:refnum<class "Switching.lvclass">)
                      n262 = call-dynamic "MatrixSwitch.vi"("Action"=T5."Striptest SMU", "Switching in"=w458) -> ()  [unwired: 7 in, 3 out]
                    }
                    frame #1 {
                      n263 = local read "settling\ndelay [ms]"() -> (w463:i32)
                      n264 = call "CurrentCorrection.vi"("Action"=T6."Reference measurement", "settling\ndelay"=w463) -> ("Compliance exceeded?"=w464:bool, "Current Reference 100V"=→"Current Reference 100V":dbl[], "Current Reference 10V"=→"Current Reference 10V":dbl[])  [unwired: 3 in, 2 out]
                    }
                  }
                }
                frame True {
                }
              }
              n265 = case shown="True" w453 {
                frame False {
                  n266 = local write "Status:"("RUN IN PROGRESS" ("STATUS 1")) -> ()
                }
                frame True {
                  n267 = property on="Bias On/Off:" class="Bool (strict)"("Blinking"=TRUE ("Compliance?")) -> ()  [unwired: 2 in, 2 out]
                  n268 = local write "Status:"("Compliance exceeded\nRUN ABORTED") -> ()
                }
              }
            }
            frame True {
            }
          }
        }
        frame #4 {
          # "Measurement"
          n269 = property on="Bias On/Off:" class="Bool (strict)"() -> ("Blinking"=w471:bool)  [unwired: 2 in, 2 out]
          n270 = case shown="False" w471 {
            tunnel: w472 -> [w482 _]
            tunnel: w470 -> [w481 _]
            tunnel: w469 -> [w480 _]
            frame False {
              n271 = local read "probe points per region"() -> (w475:i32[])
              n272 = local read "Temperature Progression"() -> (w474:T3)
              n273 = local read "max scale array"() -> (w478:i32[])
              n274 = local read "min scale array"() -> (w477:i32[])
              n275 = Array Size(array=w482) -> (size(s)=w483:i32)
              n276 = for {
                N: w483 -> [_]
                tunnel: w482 -> [w496] mode=indexing
                tunnel: w481 -> [w495] mode=indexing
                tunnel: w480 -> [w494]
                shift-right: [w488] -> _
                shift-left: 0 -> [w493]
                tunnel: w478 -> [w491] mode=indexing
                tunnel: w477 -> [w492] mode=indexing
                shift-right: [w487] -> _
                shift-left: 0 -> [w489]
                tunnel: w475 -> [w486] mode=indexing
                shift-right: [w484] -> w473
                shift-left: w474 -> [w485]
                i -> [w490]
                n277 = case shown="True" w496 {
                  tunnel: w495 -> [_ w512]
                  tunnel: w494 -> [_ _]
                  tunnel: w493 -> [w498 w513]
                  tunnel: w492 -> [_ w508]
                  tunnel: w491 -> [_ w505]
                  tunnel: w490 -> [_ w510]
                  tunnel: w489 -> [w500 w507]
                  tunnel: [w497 w506] -> w488
                  tunnel: [w500 w504] -> w487
                  tunnel: w486 -> [_ w503]
                  tunnel: w485 -> [w499 w502]
                  tunnel: [w499 w501] -> w484
                  frame False {
                    n278 = Increment(x=w498) -> (x+1=w497:i32)
                  }
                  frame True {
                    n279 = Unbundle By Name(w512) -> ("Region"=→"Probing Region:":string, "ProbePoints"=w509:T12)
                    n280 = local write "Show:"(w513) -> ()
                    n281 = while {
                      tunnel: w510 -> [w515]
                      tunnel: w509 -> [w534]
                      shift-right: [w527] -> _
                      shift-left: w508 -> [w516]
                      shift-right: [w528] -> w504
                      shift-left: w507 -> [w529]
                      tunnel: w505 -> [w526]
                      tunnel: w503 -> [_]
                      shift-right: [w524] -> w501
                      shift-left: w502 -> [w525]
                      i -> [w530]
                      stop <- w533 stop-if-true
                      # "FULL STRIP TEST MEASUREMENT LOOP"
                      n282 = Equal To 0?(x=w529) -> (x = 0?=w536:bool)
                      n283 = Equal?(x=w516, y=w526) -> (x = y?=w514:bool)
                      n284 = Index Array(array=w534, index=w516) -> (element=w535:T15)
                      n285 = case shown="True" w536 {
                        frame False {
                        }
                        frame True {
                          # "Estimation of test time"
                          n286 = local read "Probe Card Channels"() -> (w1096:i32)
                          n287 = local read "total strip number"() -> (w1097:u32)
                          n288 = Divide(x=w1097, y=w1096) -> (x/y=w1095:dbl)
                          n289 = To Long Integer(number=w1095) -> (32bit integer=w1094:i32)
                          n290 = call "RunTime.vi"("no. measurements"=w1094, "Flag"=1) -> ()  [unwired: 2 in, 4 out]
                        }
                      }
                      n291 = property on="Bias On/Off:" class="Bool (strict)"() -> ("Blinking"=w531:bool)  [unwired: 2 in, 2 out]
                      n292 = Build Array(w531, "Abort", w514) -> (w532:bool[])
                      n293 = Unbundle By Name(w535) -> ("CardViable?"=w521:bool)
                      n294 = Or Array Elements(Boolean array=w532) -> (logical OR=w533:bool)
                      n295 = property on="Bias On/Off:" class="Bool (strict)"() -> ("Blinking"=w523:bool)  [unwired: 2 in, 2 out]
                      n296 = local read "Abort"() -> (w519:bool)
                      n297 = Not(x=w523) -> (.not. x?=w522:bool)
                      n298 = Not(x=w519) -> (.not. x?=w518:bool)
                      n299 = Compound Arithmetic op=AND(w521, w522, w518) -> (w520:bool)
                      n300 = case shown="True" w520 {
                        tunnel: w515 -> [_ w555]
                        tunnel: w534 -> [_ w554]
                        tunnel: w516 -> [w537 w549]
                        tunnel: w530 -> [_ w553]
                        tunnel: w529 -> [w540 w552]
                        tunnel: [w540 w551] -> w528
                        tunnel: [w538 w550] -> w527
                        tunnel: w525 -> [w539 w548]
                        tunnel: [w539 w547] -> w524
                        tunnel: w514 -> [_ w541]
                        frame False {
                          n301 = Increment(x=w537) -> (x+1=w538:i32)
                        }
                        frame True {
                          n302 = global read "QC_MeasurementSetup.vi" "Striptest Measurement Parameters"() -> (w545:T8)
                          n303 = Unbundle By Name(w545) -> ("ProbeStation"=w544:refnum<class "ProbeStationControl.lvclass">, "Switching"=w546:refnum<class "Switching.lvclass">, "Temperature Readout"=w542:enum16{"Read Arduino", "Enter manually"}, "Arduino"=w543:refnum<class "ArduinoControl.lvclass">)
                          n304 = stacked-sequence {
                            tunnel: w555 -> [w570 w851 w941 w1052 w1068]
                            tunnel: w554 -> [w559 _ _ _ _]
                            tunnel: w549 -> [w558 _ _ _ w1074]
                            tunnel: w552 -> [_ _ _ _ w1083]
                            tunnel: w553 -> [_ w850 w940 w1051 w1072]
                            tunnel: [_ _ _ _ w1075] -> w551
                            tunnel: [_ _ _ _ w1082] -> w550
                            tunnel: w548 -> [_ w845 _ _ _]
                            tunnel: [_ w844 _ _ _] -> w547
                            tunnel: w546 -> [_ w848 w938 _ _]
                            tunnel: w544 -> [w557 _ _ _ _]
                            tunnel: w543 -> [_ w847 _ _ _]
                            tunnel: w542 -> [_ w846 _ _ _]
                            tunnel: w541 -> [_ _ _ _ w1067]
                            frame #0 {
                              w569 = u32 4 items=["Reset", "Read Array", "Read Element", "Write Element", "Write Array"] ("Action")
                              # "Huge inefficinecy here that could be exploited"
                              # ">min scale>"
                              # ">min scale>"
                              # "MOVE TO NEXT STRIP TO TEST"
                              n305 = Index Array(array=w559, index=w558) -> (element=w577:T15)
                              n306 = local write "disabled channels"(i32[] []) -> ()
                              n307 = Unbundle(w577) -> ("Label"=w573:string)  [unwired: 3 out]
                              "Probe Point:" <- w573
                              n308 = Format Into String(format string="Moving to %s", w573) -> (resulting string=w576:string)  [unwired: 2 in, 1 out]
                              n309 = local write "Status:"(w576) -> ()
                              n310 = local read "Simulation?"() -> (w563:bool)
                              n311 = local read "Abort"() -> (w565:bool)
                              n312 = xnode "Match Regular Expression"("input string"=w573, "regular expression"="(Strip|Channel)\\s+(\\d+)", "ignore case? (F)"=TRUE) -> ("submatch 2"=w562:string)  [unwired: 3 in, 6 out]
                              n313 = local read "Probe Card Channels"() -> (w566:i32)
                              n314 = local read "Probe Card Channels"() -> (w556:i32)
                              n315 = Empty String/Path?(string/path=w562) -> (empty?=w561:bool)
                              n316 = Or(x=w565, y=w563) -> (x .or. y?=w564:bool)
                              n317 = Not(x=w561) -> (.not. x?=w560:bool)
                              n318 = case shown="True" w560 {
                                tunnel: [w579 w589] -> w571
                                tunnel: w558 -> [w581 w587]
                                tunnel: w556 -> [w580 w588]
                                tunnel: w559 -> [_ w586]
                                frame False {
                                n319 = for {
                                N: w580 -> [_]
                                tunnel: w581 -> [w584]
                                tunnel: [w582] -> w579 mode=indexing
                                i -> [w585]
                                # "Actually use the probepoint\nindex"
                                n320 = Add(x=w584, y=w585) -> (x+y=w583:i32)
                                n321 = Increment(x=w583) -> (x+1=w582:i32)
                                }
                                }
                                frame True {
                                # "If probepoint label defined as Strip or Channel, use that as the channel number in the data array"
                                n322 = for {
                                N: w588 -> [_]
                                tunnel: [w598] -> w589 mode=indexing
                                tunnel: w587 -> [w595]
                                tunnel: w586 -> [w593]
                                i -> [w596]
                                n323 = Add(x=w595, y=w596) -> (x+y=w594:i32)
                                n324 = Index Array(array=w593, index=w594) -> (element=w592:T15)
                                n325 = Unbundle By Name(w592) -> ("Label"=w591:string)
                                n326 = xnode "Match Regular Expression"("input string"=w591, "regular expression"="(Strip|Channel)\\s+(\\d+)") -> ("submatch 2"=w590:string)  [unwired: 4 in, 6 out]
                                n327 = Scan From String(format string="%d", input string=w590) -> (output 1=w598:i32)  [unwired: 3 in, 3 out]
                                }
                                }
                              }
                              n328 = case shown="False" w564 {
                                tunnel: w570 -> [w836 _]
                                tunnel: w558 -> [w837 _]
                                tunnel: w566 -> [w838 _]
                                tunnel: w557 -> [w834 _]
                                frame False {
                                # "Move to strip"
                                n329 = local read "Single Needle"() -> (w840:bool)
                                n330 = call "MoveToStrip.vi"("Single Needle"=w840, "Strip No."=w837, "Region"=w836, "ProbeStationControl in"=w834) -> ("Z [µm]"=w835:i32)  [unwired: 5 in, 2 out]
                                n331 = local read "Z profile"() -> (w843:i32[][])
                                n332 = Initialize Array(w835, w838, 1) -> (w841:i32[][])
                                n333 = Replace Array Subset(array=w843, new element=w841, index (row)=w837, index (col)=w836) -> (w842:i32[][])
                                n334 = local write "Z profile"(w842) -> ()
                                }
                                frame True {
                                }
                              }
                              n335 = To Double Precision Float(number=w571) -> (double precision float=w567:dbl[])
                              n336 = call "MultiRegionData.vi"("Action"=w569, "Array No."=0 ("Array Size / Index"), "Array Size / Index"=w558, "Array IN"=w567, "Region index"=w570) -> ()  [unwired: 1 in, 2 out]
                            }
                            frame #1 {
                              # "PINHOLE MEASUREMENT"
                              n337 = local read "Simulation?"() -> (w849:bool)
                              n338 = stacked-sequence {
                                tunnel: w849 -> [w867 w888]
                                tunnel: w851 -> [_ w890]
                                tunnel: w850 -> [_ w889]
                                tunnel: w848 -> [w866 _]
                                tunnel: w847 -> [w864 _]
                                tunnel: w846 -> [w865 _]
                                tunnel: w845 -> [w859 _]
                                tunnel: [w858 _] -> w844
                                frame #0 {
                                # "Setup the Matrix for SMU measurement."
                                # "Temperature/Humidity Readout"
                                n339 = Unbundle By Name(w859) -> ("Temperature Array [°C]"=w857:dbl[], "Humidity Array [RH %]"=w856:dbl[], "Time Array"=w853:string[])
                                n340 = case shown="\"Read Arduino\", Default" w865 {
                                tunnel: w864 -> [w875 _]
                                tunnel: [w874 _] -> w863
                                tunnel: w857 -> [w870 w879]
                                tunnel: w856 -> [w871 w881]
                                tunnel: [w869 w878] -> w855
                                tunnel: [w868 w877] -> w854
                                frame "Read Arduino", Default {
                                n341 = call "ArduinoRead.vi"("Arduino function"=enum16{"T/RH", "Interlock", "Edgesense"}."T/RH", "ArduinoControl in"=w875) -> ("error out"=w874:errorcluster, "rel. Humidity [%]"=w872:dbl, "Temperature [°C]"=w873:dbl)  [unwired: 4 in, 3 out]
                                n342 = Build Array (concatenate)(w870, w873) -> (w869:dbl[])
                                n343 = Build Array (concatenate)(w871, w872) -> (w868:dbl[])
                                }
                                frame "Enter manually" {
                                n344 = Index Array(array=w879, index=0) -> (element=w880:dbl)
                                n345 = Index Array(array=w881, index=0) -> (element=w882:dbl)
                                n346 = Build Array (concatenate)(w879, w880) -> (w878:dbl[])
                                n347 = Build Array (concatenate)(w881, w882) -> (w877:dbl[])
                                }
                                }
                                n348 = case shown="False" w867 {
                                tunnel: w866 -> [w887 _]
                                tunnel: w863 -> [w886 _]
                                frame False {
                                n349 = call-dynamic "MatrixSwitch.vi"("error in (no error)"=w886, "Action"=T5."Striptest SMU", "Switching in"=w887) -> ()  [unwired: 6 in, 3 out]
                                }
                                frame True {
                                }
                                }
                                n350 = call "RunTime.vi"("Probing done - new estimation"=FALSE, "Flag"=0) -> ("Time so far"=w860:string)  [unwired: 2 in, 3 out]
                                n351 = Build Array (concatenate)(w853, w860) -> (w852:string[])
                                n352 = Bundle By Name(cluster=w859, "Temperature Array [°C]"=w855, "Humidity Array [RH %]"=w854, "Time Array"=w852) -> (w858:T3)
                                }
                                frame #1 {
                                # "Pinhole test"
                                n353 = local read "Abort"() -> (w891:bool)
                                n354 = case shown="False" w891 {
                                tunnel: w890 -> [w901 _]
                                tunnel: w889 -> [w900 _]
                                tunnel: w888 -> [w892 _]
                                frame False {
                                w897 = u32 4 items=["Reset", "Read Array", "Read Element", "Write Element", "Write Array"] ("Action")
                                w898 = u32 4 items=["Reset", "Read Array", "Read Element", "Write Element", "Write Array"] ("Action")
                                # "Pinhole test"
                                n355 = Get Date/Time String(want seconds? (F)=TRUE) -> (time string=→"Last Probe at:":string)  [unwired: 2 in, 1 out]
                                n356 = case shown="False" w892 {
                                tunnel: [w913 w926] -> w893
                                tunnel: [w910 w925] -> w899
                                frame False {
                                # "Pinhole test"
                                n357 = local read "Thresholds:"() -> (w912:T2)
                                n358 = Unbundle By Name(w912) -> ("Current [nA]"=w911:dbl)
                                n359 = case shown="False" FALSE {
                                tunnel: [w918 w920] -> w913
                                tunnel: w911 -> [w914 w923]
                                tunnel: [w917 w922] -> w910
                                tunnel: [w916 w921] -> w909
                                tunnel: "settling\ndelay [ms]" -> [w915 w919]
                                frame False {
                                n360 = call "Pinholes.vi"("Current Threshold [nA]"=w914, "settling\ndelay"=w915) -> ("excluded channels"=w916:i32[], "Current [nA]"=w918:dbl[], "Flag"=w917:i32[])  [unwired: 3 in]
                                }
                                frame True {
                                n361 = call "PinholesRolling.vi"("Current Threshold [nA]"=w923, "settling\ndelay"=w919) -> ("excluded channels"=w921:i32[], "Current [nA]"=w920:dbl[], "Flag"=w922:i32[])  [unwired: 3 in]
                                }
                                }
                                "disabled channels" <- w909
                                }
                                frame True {
                                # "Pinhole test SIMULATION"
                                n362 = local read "Probe Card Channels"() -> (w924:i32)
                                n363 = for {
                                N: w924 -> [_]
                                tunnel: [w928] -> w926 mode=indexing
                                tunnel: [w927] -> w925 mode=indexing
                                n364 = Random Number (0-1)() -> (number: 0 to 1=w931:dbl)
                                n365 = Greater?(x=w931, y=0.95) -> (0:w932:bool)
                                n366 = case shown="True" w932 {
                                tunnel: [w936 5000.0] -> w928
                                tunnel: w931 -> [w936 _]
                                frame False {
                                }
                                frame True {
                                }
                                }
                                n367 = Greater?(x=w928, y=50.0) -> (0:w929:bool)
                                n368 = case shown="False" w929 {
                                tunnel: [0 1] -> w927
                                frame False {
                                }
                                frame True {
                                }
                                }
                                }
                                }
                                }
                                n369 = local write "Status:"("Measuring Ipinhole") -> ()
                                n370 = Index Array(array=w893, index=0) -> (element=→"Current [nA]:":dbl)
                                n371 = call "MultiRegionData.vi"("Action"=w897, "Array No."=1, "Array Size / Index"=w900, "Array IN"=w893, "Region index"=w901) -> ()  [unwired: 1 in, 2 out]
                                n372 = To Double Precision Float(number=w899) -> (double precision float=w896:dbl[])
                                n373 = call "MultiRegionData.vi"("Action"=w898, "Array No."=2, "Array Size / Index"=w900, "Array IN"=w896, "Region index"=w901) -> ()  [unwired: 1 in, 2 out]
                                }
                                frame True {
                                }
                                }
                                }
                              }
                            }
                            frame #2 {
                              # "Capacitance and Resistance"
                              # "CAPACITANCE/RESISTANCE MEASUREMENT"
                              n374 = local read "Simulation?"() -> (w939:bool)
                              n375 = stacked-sequence {
                                seq-local: [_ _ w952 _] -> [_ _ _ w1024]
                                tunnel: w941 -> [_ _ w965 _]
                                tunnel: w940 -> [_ _ w964 _]
                                tunnel: w939 -> [w943 w947 w955 w1023]
                                tunnel: w938 -> [w942 w946 w954 w1022]
                                frame #0 {
                                # "Switching Matrix Ground"
                                n376 = case shown="False" w943 {
                                tunnel: w942 -> [w945 _]
                                frame False {
                                n377 = call-dynamic "MatrixSwitch.vi"("Action"=T5."Ground", "Switching in"=w945) -> ()  [unwired: 7 in, 3 out]
                                }
                                frame True {
                                }
                                }
                                }
                                frame #1 {
                                # "LCR Mode in Switching Matrix"
                                n378 = case shown="False" w947 {
                                tunnel: w946 -> [w950 _]
                                frame False {
                                n379 = call-dynamic "MatrixSwitch.vi"("Action"=T5."Striptest LCR", "Switching in"=w950) -> ()  [unwired: 7 in, 3 out]
                                }
                                frame True {
                                }
                                }
                                n380 = local write "Status:"("Measuring capacitance..." ("STATUS 1")) -> ()
                                }
                                frame #2 {
                                w962 = u32 4 items=["Reset", "Read Array", "Read Element", "Write Element", "Write Array"] ("Action")
                                w963 = u32 4 items=["Reset", "Read Array", "Read Element", "Write Element", "Write Array"] ("Action")
                                # "Same as in pinhole test... have removed unnecessary switching for single needle tests."
                                # "Capacitance/Resistance Test"
                                n381 = local read "Probe Card Channels"() -> (w956:i32)
                                n382 = local read "disabled channels"() -> (w958:i32[])
                                n383 = for {
                                N: w956 -> [_]
                                tunnel: [w974] -> w957 mode=indexing
                                tunnel: [w973] -> w960 mode=indexing
                                tunnel: w958 -> [w970]
                                tunnel: w956 -> [w972]
                                tunnel: w955 -> [w969]
                                tunnel: w954 -> [w968]
                                i -> [w971]
                                n384 = case shown="False" w969 {
                                tunnel: [w983 w1013] -> w974
                                tunnel: [w982 w1012] -> w973
                                tunnel: w972 -> [w979 _]
                                tunnel: w971 -> [w977 _]
                                tunnel: w970 -> [w978 _]
                                tunnel: w968 -> [w975 _]
                                frame False {
                                n385 = Increment(x=w977) -> (x+1=w976:i32)
                                n386 = Search 1D Array(1D array=w978, element=w976) -> (index of element=w981:i32)  [unwired: 1 in]
                                n387 = Less Than 0?(x=w981) -> (x < 0?=w980:bool)
                                n388 = case shown="True" w980 {
                                tunnel: [w986 w992] -> w983
                                tunnel: [w984 w991] -> w982
                                tunnel: w979 -> [_ w990]
                                tunnel: w976 -> [_ w989]
                                tunnel: w978 -> [_ w988]
                                tunnel: w975 -> [_ w987]
                                frame False {
                                w986 = -1.0
                                n389 = Divide(x=w986, y=1000000.0) -> (x/y=w984:dbl)
                                }
                                frame True {
                                n390 = stacked-sequence {
                                tunnel: w990 -> [w995 _ _]
                                tunnel: w989 -> [w997 _ _]
                                tunnel: w988 -> [w996 _ _]
                                tunnel: [_ _ w1011] -> w992
                                tunnel: [_ _ w1006] -> w991
                                tunnel: w987 -> [w994 _ _]
                                frame #0 {
                                n391 = local read "Single Needle"() -> (w993:bool)
                                n392 = case shown="True" w993 {
                                tunnel: w997 -> [w1003 _]
                                tunnel: w996 -> [w1002 _]
                                tunnel: w995 -> [w1001 _]
                                tunnel: w994 -> [w1000 _]
                                tunnel: w993 -> [w999 _]
                                frame False {
                                n393 = call-dynamic "MuxCardSwitch.vi"("Instrument"=enum16{"SMU", "LCR"}."LCR", "Single Needle"=w999, "Probe Card Channels"=w1001, "disabled channels"=w1002, "Switch to channel"=w1003, "Switching in"=w1000) -> ()  [unwired: 3 in, 3 out]
                                }
                                frame True {
                                }
                                }
                                }
                                frame #1 {
                                n394 = local read "settling\ndelay [ms]"() -> (w1004:i32)
                                n395 = Wait (ms)(milliseconds to wait=w1004) -> ()  [unwired: 1 out]
                                }
                                frame #2 {
                                n396 = global read "QC_MeasurementSetup.vi" "Striptest Measurement Parameters"() -> (w1010:T8)
                                n397 = Unbundle By Name(w1010) -> ("LCR"=w1009:refnum<class "LCRControl.lvclass">, "AC frequency [Hz]"=w1008:i32)
                                n398 = call-dynamic "LCR_Readout.vi"("Frequency in Hz"=w1008, "LCRControl in"=w1009) -> ("Resistance in Ohm"=w1007:dbl, "Capacitance in pF"=w1011:dbl)  [unwired: 6 in, 2 out]
                                n399 = Divide(x=w1007, y=1000000.0) -> (x/y=w1006:dbl)
                                }
                                }
                                }
                                }
                                }
                                frame True {
                                n400 = Random Number (0-1)() -> (number: 0 to 1=w1017:dbl)
                                n401 = Random Number (0-1)() -> (number: 0 to 1=w1021:dbl)
                                n402 = Multiply(x=w1021, y=18.0) -> (x*y=w1019:dbl)
                                n403 = Multiply(x=w1017, y=0.6) -> (x*y=w1014:dbl)
                                n404 = Add(x=w1019, y=64.0) -> (x+y=w1013:dbl)
                                n405 = Add(x=1.5 ("Resistance"), y=w1014) -> (x+y=w1012:dbl)
                                }
                                }
                                }
                                n406 = Index Array(array=w960, index=0) -> (element=→"Reistance [MW]:":dbl)
                                n407 = Index Array(array=w957, index=0) -> (element=→"Capacitance [pF]:":dbl)
                                n408 = local read "Probe Card Channels"() -> (w952:i32)
                                n409 = call "MultiRegionData.vi"("Action"=w963, "Array No."=3, "Array Size / Index"=w964, "Array IN"=w957, "Region index"=w965) -> ()  [unwired: 1 in, 2 out]
                                n410 = call "MultiRegionData.vi"("Action"=w962, "Array No."=4, "Array Size / Index"=w964, "Array IN"=w960, "Region index"=w965) -> ()  [unwired: 1 in, 2 out]
                                }
                                frame #3 {
                                n411 = case shown="False" w1023 {
                                tunnel: w1024 -> [w1028 _]
                                tunnel: w1022 -> [w1027 _]
                                frame False {
                                n412 = local read "Single Needle"() -> (w1025:bool)
                                n413 = case shown="True" w1025 {
                                tunnel: w1028 -> [w1032 _]
                                tunnel: w1025 -> [w1031 _]
                                tunnel: w1027 -> [w1030 _]
                                tunnel: enum16{"SMU", "LCR"}."LCR" ("Instrument") -> [w1029 _]
                                frame False {
                                n414 = call-dynamic "MuxCardSwitch.vi"("Instrument"=w1029, "Single Needle"=w1031, "Probe Card Channels"=w1032, "Switch to channel"=-1, "Switching in"=w1030) -> ()  [unwired: 4 in, 3 out]
                                }
                                frame True {
                                }
                                }
                                }
                                frame True {
                                }
                                }
                                }
                              }
                            }
                            frame #3 {
                              # "Display results in plots"
                              # "If selected region is CURRENT region being probed,\nuse number probed so far\notherwise total number of probepoints in this region"
                              # "UPDATE PLOTS + INDICATORS + ANALYSIS DEFECTS/BAD STRIPS"
                              n415 = local read "Region Indices"() -> (w1054:i32[])
                              n416 = local read "max scale array"() -> (w1046:i32[])
                              n417 = local read "min scale array"() -> (w1035:i32[])
                              n418 = Index Array(array=w1054, index="Show:") -> (element=w1050:i32)
                              n419 = Index Array(array=w1035, index="Show:") -> (element=w1045:i32)
                              n420 = Index Array(array=w1046, index="Show:") -> (element=w1043:i32)
                              n421 = Equal?(x=w1050, y=w1052) -> (x = y?=w1053:bool)
                              n422 = Increment(x=w1043) -> (x+1=w1042:i32)
                              n423 = Increment(x=w1045) -> (x+1=w1044:i32)
                              n424 = Increment(x=w1042) -> (x+1=w1041:i32)
                              n425 = case shown="True" w1053 {
                                tunnel: w1051 -> [_ w1066]
                                tunnel: [w1062 w1065] -> w1049
                                tunnel: w1050 -> [w1061 _]
                                frame False {
                                n426 = local read "probe points per region"() -> (w1063:i32[])
                                n427 = Index Array(array=w1063, index=w1061) -> (element=w1062:i32)
                                }
                                frame True {
                                n428 = local read "Probe Card Channels"() -> (w1064:i32)
                                n429 = Add(x=w1064, y=w1066) -> (x+y=w1065:i32)
                                }
                              }
                              n430 = property on="Capacitance [pF]" class="WFGraph (strict)"("XScale.Maximum"=w1042) -> ()  [unwired: 2 in, 2 out]
                              n431 = property on="Defects" class="IntGraph (strict)"("XScale.Maximum"=w1041) -> ()  [unwired: 2 in, 2 out]
                              n432 = property on="Resistance [MW]" class="WFGraph (strict)"("XScale.Maximum"=w1042) -> ()  [unwired: 2 in, 2 out]
                              n433 = property on="Current [nA]" class="WFGraph (strict)"("XScale.Maximum"=w1042) -> ()  [unwired: 2 in, 2 out]
                              n434 = property on="Capacitance [pF]" class="WFGraph (strict)"("XScale.Minimum"=w1044) -> ()  [unwired: 2 in, 2 out]
                              n435 = property on="Resistance [MW]" class="WFGraph (strict)"("XScale.Minimum"=w1044) -> ()  [unwired: 2 in, 2 out]
                              n436 = property on="Current [nA]" class="WFGraph (strict)"("XScale.Minimum"=w1044) -> ()  [unwired: 2 in, 2 out]
                              n437 = property on="Defects" class="IntGraph (strict)"("XScale.Minimum"=w1044) -> ()  [unwired: 2 in, 2 out]
                              n438 = local read "Thresholds:"() -> (w1060:T2)
                              n439 = local read "min scale array"() -> (w1048:i32[])
                              n440 = local read "max scale array"() -> (w1034:i32[])
                              n441 = call "DisplayStriptestData.vi"("min scale array"=w1048, "max scale array"=w1034, "# probed"=w1049, "Display Stats?"=TRUE, "Thresholds"=w1060, "Region"=w1050) -> ("Defects"=→"Defects":i32[][], "Resistance [MW]"=→"Resistance [MW]":cluster{u32, i32, "Array OUT":dbl[]}, "Capacitance [pF]"=→"Capacitance [pF]":cluster{u32, i32, "Array OUT":dbl[]}, "Current [nA]"=→"Current [nA]":cluster{u32, i32, "Array OUT":dbl[]}, "Strip Quality Data"=w1056:T16)
                              n442 = Unbundle By Name(w1056) -> ("pass Rate in %"=→"% OK:":dbl, "Bad channel list"=→"Bad Strip List":i32[], "No of bad strips"=w1039:i32, "Number of defects per category"=→"defect type array":i32[])
                              n443 = local write "# total defects:"(w1039) -> ()
                            }
                            frame #4 {
                              # "Removed image capture as has been cannot find the path. Likely a small \nbug but I do not think we need these images anyhow."
                              # "SAVE IMAGE + TEST TIME UPDATE"
                              n444 = local read "Probe Card Channels"() -> (w1073:i32)
                              n445 = case shown="True" w1067 {
                                tunnel: w1068 -> [_ w1089]
                                frame False {
                                }
                                frame True {
                                # "Create temp data file."
                                n446 = local read "Temperature Progression"() -> (w1086:T3)
                                n447 = Unbundle By Name(w1086) -> ("Temperature Array [°C]"=w1088:dbl[], "Humidity Array [RH %]"=w1087:dbl[])
                                n448 = call <vilib>:"Std Deviation and Variance.vi"("X"=w1088) -> ("mean"=w1085:dbl)  [unwired: 1 in, 2 out]
                                n449 = call <vilib>:"Std Deviation and Variance.vi"("X"=w1087) -> ("mean"=w1084:dbl)  [unwired: 1 in, 2 out]
                                n450 = local read "Probing Region:"() -> (w1090:string)
                                n451 = call "SaveStriptestRecoveryFiles.vi"("Array Titles"="ProbeplanIndex\tCurrent[nA]\tCapacitance[pF]\tResistance[MOhm]\n", "Strip Segment"=w1090, "Humidity"=w1084, "Temperature"=w1085, "Region #"=w1089) -> ()  [unwired: 1 in, 2 out]
                                }
                              }
                              n452 = Quotient & Remainder(x=w1072, y=w1073) -> (floor(x/y)=w1071:i32)  [unwired: 1 out]
                              n453 = Add(x=w1073, y=w1083) -> (x+y=w1075:i32)
                              n454 = Increment(x=w1071) -> (x+1=w1070:i32)
                              n455 = local write "# probed"(w1075) -> ()
                              n456 = case shown="False" FALSE {
                                tunnel: w1070 -> [_ w1093]
                                frame False {
                                }
                                frame True {
                                n457 = call "SaveJPEG.vi"("Picture No."=w1093, "Test"="Striptest") -> ()  [unwired: 1 in, 2 out]
                                }
                              }
                              n458 = call "RunTime.vi"("Probing done - new estimation"=TRUE, "Flag"=0) -> ("Estimated Completion Time"=w1079:string, "Time so far"=→"Run Duration:":string)  [unwired: 2 in, 2 out]
                              n459 = Scan From String(format string="%s %s", input string=w1079) -> (output 2=→"Estimated Completion:":string)  [unwired: 5 in, 3 out]
                              n460 = Increment(x=w1074) -> (x+1=w1082:i32)
                            }
                          }
                        }
                      }
                    }
                    n461 = Increment(x=w513) -> (x+1=w506:i32)
                  }
                }
              }
              n462 = local write "Temperature Progression"(w473) -> ()
            }
            frame True {
            }
          }
        }
        frame #5 {
          # "End of run"
          n463 = local read "Abort"() -> (w1112:bool)
          n464 = property on="Bias On/Off:" class="Bool (strict)"() -> ("Blinking"=w1111:bool)  [unwired: 2 in, 2 out]
          n465 = case shown="False" w1100 {
            tunnel: w1099 -> [w1121 _]
            frame False {
              w1119 = "none"
              w1124 = "0"
              n466 = property on="Abort" class="Bool (strict)"("DisabledEnum"=2) -> ()  [unwired: 2 in, 2 out]
              n467 = call-dynamic "Prober_ChuckUpDown.vi"("Direction"=enum16{"up", "down"}."down", "ProbeStationControl in"=w1121) -> ("error out"=w1123:errorcluster, "ProbeStationControl out"=w1122:refnum<class "ProbeStationControl.lvclass">)  [unwired: 7 in, 1 out]
              n468 = case shown="True" FALSE {
                frame False {
                }
                frame True {
                  n469 = local read "# probed"() -> (w1127:i32)
                  n470 = call "SaveJPEG.vi"("Picture No."=w1127, "Test"="Striptest") -> ()  [unwired: 1 in, 2 out]
                }
              }
              n471 = call-dynamic "Prober_MoveToXYZTheta.vi"("Theta location [mdeg]"=w1119, "ProbeStationControl in"=w1122, "error in (no error)"=w1123, "Z location [µm]"=w1119, "Y location [µm]"=w1124, "X location [µm]"=w1124) -> ()  [unwired: 3 in, 3 out]
            }
            frame True {
            }
          }
          n472 = Not Or(1:w1112, 2:w1111) -> (0:w1110:bool)
          n473 = Build Array(w1110, w1111, w1112) -> (w1113:bool[])
          n474 = Search 1D Array(1D array=w1113, element=TRUE) -> (index of element=w1115:i32)  [unwired: 1 in]
          n475 = Increment(x=w1115) -> (x+1=w1101:i32)
          n476 = Pick Line(multi-line string=" null\n Run ended normally.\n Compliance exceeded. \n Run aborted early.", line index=w1101) -> (output string=w1102:string)  [unwired: 1 in]
          n477 = global read "QC_RunInformation.vi" "Run info"() -> (w1104:T10)
          n478 = Bundle By Name(cluster=w1104, "End of Run comment:"=w1102) -> (w1103:T10)
          n479 = global write "QC_RunInformation.vi" "Run info"(w1103) -> ()
          n480 = Concatenate Strings(" End of Run.", "\r\n", w1102) -> (w1105:string)
          n481 = Concatenate Strings(w1102, "\r\n", "RAMPING DOWN VOLTS") -> (w1108:string)
          n482 = stacked-sequence {
            tunnel: w1108 -> [w1128 _ _ _]
            tunnel: w1105 -> [_ _ w1132 _]
            frame #0 {
              n483 = local write "Status:"(w1128) -> ()
            }
            frame #1 {
              n484 = local read "Simulation?"() -> (w1129:bool)
              n485 = case shown="False" w1129 {
                frame False {
                  n486 = global read "QC_MeasurementSetup.vi" "Striptest Measurement Parameters"() -> (w1131:T8)
                  n487 = Unbundle By Name(w1131) -> ("SMU"=w1130:refnum<class "SupplyControl.lvclass">)
                  n488 = call-dynamic "Supply_Stby.vi"("SupplyControl in"=w1130) -> ()  [unwired: 9 in, 2 out]
                }
                frame True {
                }
              }
            }
            frame #2 {
              n489 = local write "Status:"(w1132) -> ()
            }
            frame #3 {
              w1134 = 0
              n490 = property on="Save Data" class="Bool (strict)"("DisabledEnum"=w1134) -> ()  [unwired: 2 in, 2 out]
              n491 = property on="Quit w/o saving" class="Bool (strict)"("DisabledEnum"=w1134) -> ()  [unwired: 2 in, 2 out]
              n492 = local write "Status:"("Run finished. \nSave data?" ("STATUS 1")) -> ()
            }
          }
        }
        frame #6 {
          # "LAST STEPS: SAVE DATA + SWITCH OFF ARDUINO + SAVE IMAGE + DISPLAY DATA + GENERATES DB FILE + SENSOR PASS/FAIL DECISION"
          n493 = stacked-sequence {
            tunnel: [w1168 _ _ _] -> w1164
            tunnel: [w1167 _ _ _] -> w1163
            tunnel: w1157 -> [_ w1270 w1286 _]
            tunnel: w1156 -> [w1166 _ _ _]
            frame #0 {
              # "Save data"
              n494 = local read "Show:"() -> (w1169:u16)
              n495 = while {
                shift-right: [w1177] -> _
                shift-left: w1169 -> [w1172]
                tunnel: ["Save Data"] -> w1167
                tunnel: ["Quit w/o saving"] -> w1168
                tunnel: w1166 -> [w1173]
                stop <- w1179 stop-if-true
                w1170 = FALSE
                # "Did not remove recheck code \nbut removed ability for user to \naccess it."
                # "Loop and await decision on whether to save or junk data"
                n496 = local read "Show:"() -> (w1171:u16)
                n497 = Wait (ms)(milliseconds to wait=u32 200) -> ()  [unwired: 1 out]
                n498 = Not Equal?(x=w1172, y=w1171) -> (x != y?=w1178:bool)
                n499 = case shown="True" w1170 {
                  tunnel: w1170 -> [_ w1181]
                  tunnel: w1173 -> [_ w1180]
                  frame False {
                  }
                  frame True {
                    n500 = case shown="True" w1181 {
                      tunnel: w1180 -> [_ w1211]
                      frame False {
                        n501 = local read "Show:"() -> (w1187:u16)
                        n502 = local read "probe points per region"() -> (w1188:i32[])
                        n503 = local read "Region Indices"() -> (w1189:i32[])
                        n504 = Index Array(array=w1189, index=w1187) -> (element=w1186:i32)
                        n505 = Index Array(array=w1188, index=w1187) -> (element=w1185:i32)
                        n506 = flat-sequence {
                          tunnel: w1186 -> [w1191]
                          tunnel: w1185 -> [w1194]
                          tunnel: [w1191] -> w1184
                          tunnel: [w1194] -> w1183
                          tunnel: [w1193] -> w1182
                          tunnel: w1184 -> [w1210]
                          tunnel: w1183 -> [w1207]
                          tunnel: w1182 -> [w1196]
                          frame #0 {
                            n507 = local read "Thresholds:"() -> (w1195:T2)
                            n508 = local read "Probe Card Channels"() -> (w1192:i32)
                            n509 = call "ReCheckStrips.vi"("Probe Card Channels"=w1192, "Auto Re-Check"=FALSE, "Thresholds"=w1195, "region in"=w1191, "Number of strips probed"=w1194) -> ("Thresholds copy"=w1193:T17)  [unwired: 6 in]
                            n510 = local write "Thresholds:"(w1193) -> ()
                          }
                          frame #1 {
                            n511 = local read "min scale array"() -> (w1208:i32[])
                            n512 = local read "max scale array"() -> (w1209:i32[])
                            n513 = call "DisplayStriptestData.vi"("min scale array"=w1208, "max scale array"=w1209, "# probed"=w1207, "Display Stats?"=TRUE, "Thresholds"=w1196, "Region"=w1210) -> ("Defects"=w1202:i32[][], "Resistance [MW]"=w1203:cluster{u32, i32, "Array OUT":dbl[]}, "Capacitance [pF]"=w1205:cluster{u32, i32, "Array OUT":dbl[]}, "Current [nA]"=w1204:cluster{u32, i32, "Array OUT":dbl[]}, "Strip Quality Data"=w1201:T16)
                            n514 = Unbundle By Name(w1201) -> ("pass Rate in %"=w1200:dbl, "Bad channel list"=w1199:i32[], "No of bad strips"=w1198:i32, "Defect description list"=w1197:i32[])
                            n515 = local write "Current [nA]"(w1204) -> ()
                            n516 = local write "Capacitance [pF]"(w1205) -> ()
                            n517 = local write "Resistance [MW]"(w1203) -> ()
                            n518 = local write "Defects"(w1202) -> ()
                            n519 = local write "% OK:"(w1200) -> ()
                            n520 = local write "Bad Strip List"(w1199) -> ()
                            n521 = local write "# total defects:"(w1198) -> ()
                            n522 = local write "defect type array"(w1197) -> ()
                          }
                        }
                      }
                      frame True {
                        # "Auto ReCheck Option"
                        n523 = flat-sequence {
                          tunnel: w1211 -> [w1212]
                          frame #0 {
                            n524 = local read "Region Indices"() -> (w1213:i32[])
                            n525 = Array Size(array=w1213) -> (size(s)=w1214:i32)
                            n526 = for {
                              N: w1214 -> [_]
                              tunnel: w1213 -> [w1216] mode=indexing
                              tunnel: w1212 -> [w1215] mode=indexing
                              n527 = case shown="True" w1215 {
                                tunnel: w1216 -> [_ w1220]
                                frame False {
                                }
                                frame True {
                                n528 = local read "probe points per region"() -> (w1222:i32[])
                                n529 = Index Array(array=w1222, index=w1220) -> (element=w1221:i32)
                                n530 = flat-sequence {
                                tunnel: w1220 -> [w1227]
                                tunnel: w1221 -> [w1226]
                                tunnel: [w1227] -> w1219
                                tunnel: [w1226] -> w1218
                                tunnel: [w1225] -> w1217
                                tunnel: w1219 -> [w1243]
                                tunnel: w1218 -> [w1240]
                                tunnel: w1217 -> [w1229]
                                frame #0 {
                                n531 = local read "Probe Card Channels"() -> (w1224:i32)
                                n532 = local read "Thresholds:"() -> (w1228:T2)
                                n533 = call "ReCheckStrips.vi"("Probe Card Channels"=w1224, "Auto Re-Check"=FALSE, "Thresholds"=w1228, "region in"=w1227, "Number of strips probed"=w1226) -> ("Thresholds copy"=w1225:T17)  [unwired: 6 in]
                                n534 = local write "Thresholds:"(w1225) -> ()
                                }
                                frame #1 {
                                n535 = local read "max scale array"() -> (w1242:i32[])
                                n536 = local read "min scale array"() -> (w1241:i32[])
                                n537 = call "DisplayStriptestData.vi"("min scale array"=w1241, "max scale array"=w1242, "# probed"=w1240, "Display Stats?"=TRUE, "Thresholds"=w1229, "Region"=w1243) -> ("Defects"=w1235:i32[][], "Resistance [MW]"=w1236:cluster{u32, i32, "Array OUT":dbl[]}, "Capacitance [pF]"=w1238:cluster{u32, i32, "Array OUT":dbl[]}, "Current [nA]"=w1237:cluster{u32, i32, "Array OUT":dbl[]}, "Strip Quality Data"=w1234:T16)
                                n538 = local write "Current [nA]"(w1237) -> ()
                                n539 = local write "Capacitance [pF]"(w1238) -> ()
                                n540 = local write "Resistance [MW]"(w1236) -> ()
                                n541 = local write "Defects"(w1235) -> ()
                                n542 = Unbundle By Name(w1234) -> ("pass Rate in %"=w1233:dbl, "Bad channel list"=w1232:i32[], "No of bad strips"=w1231:i32, "Number of defects per category"=w1230:i32[])
                                n543 = local write "% OK:"(w1233) -> ()
                                n544 = local write "Bad Strip List"(w1232) -> ()
                                n545 = local write "# total defects:"(w1231) -> ()
                                n546 = local write "defect type array"(w1230) -> ()
                                }
                                }
                                }
                              }
                            }
                          }
                          frame #1 {
                          }
                        }
                      }
                    }
                  }
                }
                n547 = case shown="True" w1178 {
                  tunnel: w1171 -> [w1244 w1254]
                  tunnel: [w1244 w1254] -> w1177
                  frame False {
                  }
                  frame True {
                    # "Display data if selected region changes"
                    n548 = local read "probe points per region"() -> (w1264:i32[])
                    n549 = local read "Region Indices"() -> (w1255:i32[])
                    n550 = local read "max scale array"() -> (w1246:i32[])
                    n551 = local read "min scale array"() -> (w1247:i32[])
                    n552 = Index Array(array=w1255, index=w1254) -> (element=w1253:i32)
                    n553 = Index Array(array=w1264, index=w1254) -> (element=w1269:i32)
                    n554 = Index Array(array=w1246, index=w1254) -> (element=w1252:i32)
                    n555 = Index Array(array=w1247, index=w1254) -> (element=w1251:i32)
                    n556 = local read "Thresholds:"() -> (w1268:T2)
                    n557 = Increment(x=w1252) -> (x+1=w1249:i32)
                    n558 = Increment(x=w1251) -> (x+1=w1250:i32)
                    n559 = local read "max scale array"() -> (w1245:i32[])
                    n560 = local read "min scale array"() -> (w1265:i32[])
                    n561 = Increment(x=w1249) -> (x+1=w1248:i32)
                    n562 = property on="Resistance [MW]" class="WFGraph (strict)"("XScale.Minimum"=w1250) -> ()  [unwired: 2 in, 2 out]
                    n563 = property on="Defects" class="IntGraph (strict)"("XScale.Minimum"=w1250) -> ()  [unwired: 2 in, 2 out]
                    n564 = property on="Current [nA]" class="WFGraph (strict)"("XScale.Minimum"=w1250) -> ()  [unwired: 2 in, 2 out]
                    n565 = property on="Capacitance [pF]" class="WFGraph (strict)"("XScale.Minimum"=w1250) -> ()  [unwired: 2 in, 2 out]
                    n566 = call "DisplayStriptestData.vi"("min scale array"=w1265, "max scale array"=w1245, "# probed"=w1269, "Display Stats?"=TRUE, "Thresholds"=w1268, "Region"=w1253) -> ("Defects"=w1266:i32[][], "Resistance [MW]"=w1261:cluster{u32, i32, "Array OUT":dbl[]}, "Capacitance [pF]"=w1262:cluster{u32, i32, "Array OUT":dbl[]}, "Current [nA]"=w1263:cluster{u32, i32, "Array OUT":dbl[]}, "Strip Quality Data"=w1267:T16)
                    n567 = property on="Defects" class="IntGraph (strict)"("XScale.Maximum"=w1248) -> ()  [unwired: 2 in, 2 out]
                    n568 = property on="Resistance [MW]" class="WFGraph (strict)"("XScale.Maximum"=w1249) -> ()  [unwired: 2 in, 2 out]
                    n569 = property on="Current [nA]" class="WFGraph (strict)"("XScale.Maximum"=w1249) -> ()  [unwired: 2 in, 2 out]
                    n570 = property on="Capacitance [pF]" class="WFGraph (strict)"("XScale.Maximum"=w1249) -> ()  [unwired: 2 in, 2 out]
                    n571 = local write "Defects"(w1266) -> ()
                    n572 = local write "Current [nA]"(w1263) -> ()
                    n573 = local write "Capacitance [pF]"(w1262) -> ()
                    n574 = local write "Resistance [MW]"(w1261) -> ()
                    n575 = Unbundle By Name(w1267) -> ("pass Rate in %"=w1258:dbl, "Bad channel list"=w1256:i32[], "No of bad strips"=w1259:i32, "Number of defects per category"=w1257:i32[])
                    n576 = local write "% OK:"(w1258) -> ()
                    n577 = local write "Bad Strip List"(w1256) -> ()
                    n578 = local write "# total defects:"(w1259) -> ()
                    n579 = local write "defect type array"(w1257) -> ()
                  }
                }
                n580 = Or(x="Save Data", y="Quit w/o saving") -> (x .or. y?=w1179:bool)
              }
              n581 = local write "Save Data"("Auto quit &\nswitch off bias") -> ()
            }
            frame #1 {
              # "Bias supply to standby and Reset Switching Matrix"
              n582 = case shown="False" w1270 {
                frame False {
                  n583 = global read "QC_MeasurementSetup.vi" "Striptest Measurement Parameters"() -> (w1284:T8)
                  n584 = Unbundle By Name(w1284) -> ("Bias Supply"=w1276:refnum<class "SupplyControl.lvclass">, "Switching"=w1274:refnum<class "Switching.lvclass">)
                  n585 = local read "Current Bias Voltage [V]"() -> (w1279:dbl)
                  n586 = call "SupplyRamp.vi"("Requested Voltage"=0.0, "Step Size"=10.0, "Step Delay"=1000, "Supply IN"=w1276, "Starting Voltage"=w1279) -> ("error out"=w1282:errorcluster, "Supply OUT"=w1281:refnum<class "SupplyControl.lvclass">, "Current Voltage"=w1280:dbl)  [unwired: 3 in, 1 out]
                  n587 = local write "Current Bias Voltage [V]"(w1280) -> ()
                  n588 = call-dynamic "Supply_Stby.vi"("error in (no error)"=w1282, "SupplyControl in"=w1281) -> ("error out"=w1273:errorcluster)  [unwired: 8 in, 1 out]
                  n589 = call-dynamic "MatrixSwitch.vi"("error in (no error)"=w1273, "Action"=T5."Reset", "Switching in"=w1274) -> ("error out"=w1271:errorcluster, "Switching out"=w1272:refnum<class "Switching.lvclass">)  [unwired: 6 in, 1 out]
                  n590 = call-dynamic "Close.vi"("error in (no error)"=w1271, "Switching in"=w1272) -> ()  [unwired: 8 in, 2 out]
                }
                frame True {
                }
              }
            }
            frame #2 {
              # "Switch off Arduino + Save image"
              n591 = case shown="False" FALSE {
                frame False {
                }
                frame True {
                  n592 = local read "# probed"() -> (w1289:i32)
                  n593 = call "SaveJPEG.vi"("Picture No."=w1289, "Test"="Striptest") -> ()  [unwired: 1 in, 2 out]
                }
              }
              n594 = case shown="False" w1286 {
                frame False {
                  n595 = global read "QC_MeasurementSetup.vi" "Striptest Measurement Parameters"() -> (w1292:T8)
                  n596 = local read "Temperature Progression"() -> (w1291:T3)
                  n597 = Unbundle By Name(w1292) -> ("Arduino"=w1297:refnum<class "ArduinoControl.lvclass">)
                  n598 = Unbundle(w1291) -> ("Time Array"=w1300:string[], "Temperature Array [°C]"=w1295:dbl[])  [unwired: 1 out]
                  n599 = call "ArduinoRead.vi"("Arduino function"=enum16{"T/RH", "Interlock", "Edgesense"}."T/RH", "ArduinoControl in"=w1297) -> ("error out"=w1302:errorcluster, "Temperature [°C]"=w1294:dbl, "ArduinoControl out"=w1303:refnum<class "ArduinoControl.lvclass">)  [unwired: 4 in, 3 out]
                  "Last Temperature [°C]" <- w1294
                  n600 = local read "Run Duration:"() -> (w1299:string)
                  n601 = call "ArduinoClose.vi"("error in (no error)"=w1302, "ArduinoControl in"=w1303) -> ()  [unwired: 8 in, 2 out]
                  n602 = local read "Temperature Progression"() -> (w1290:T3)
                  n603 = Build Array (concatenate)(w1300, w1299) -> (w1298:string[])
                  n604 = Build Array (concatenate)(w1295, w1294) -> (w1293:dbl[])
                  n605 = Bundle(cluster=w1290, "Time Array"=w1298, "Temperature Array [°C]"=w1293) -> (w1301:T3)  [unwired: 1 in]
                  n606 = local write "Temperature Progression"(w1301) -> ()
                }
                frame True {
                }
              }
              n607 = One Button Dialog(message="Please switch bias off NOW and then open\nprobestation enclosure and raise needle.") -> ()  [unwired: 1 in, 1 out]
            }
            frame #3 {
              n608 = One Button Dialog(message="Please ensure detector bias is OFF!") -> ()  [unwired: 1 in, 1 out]
            }
          }
          n609 = global read "ProbePlanParams.vi" "ProbePlan Parameters IN"() -> (w1161:T9)
          n610 = case shown="False" w1164 {
            tunnel: [FALSE w1408] -> w1162
            frame False {
            }
            frame True {
              n611 = Two Button Dialog(message="Are you sure you don't want to save the data?", 1:"Quit" ("F button name (\"Cancel\")"), 2:"Save data" ("T button name (\"OK\")")) -> (T button?=w1408:bool)
            }
          }
          n612 = Unbundle By Name(w1161) -> ("Test ProbePoints.Regions Enabled"=w1159:bool[], "ProbePlan array"=w1158:T11)
          n613 = Or(x=w1163, y=w1162) -> (x .or. y?=w1152:bool)
          n614 = Array Size(array=w1159) -> (size(s)=w1160:i32)
          n615 = case shown="True" w1152 {
            tunnel: w1160 -> [w1311 w1339]
            tunnel: w1159 -> [w1310 w1338]
            tunnel: w1158 -> [_ w1337]
            tunnel: [w1306 w1335] -> w1155
            tunnel: [w1308 w1333] -> w1154
            tunnel: ["" w1330] -> w1153
            frame False {
              n616 = for {
                N: w1311 -> [_]
                tunnel: w1310 -> [w1315] mode=indexing
                tunnel: [w1314] -> w1309 mode=indexing
                tunnel: [w1313] -> w1307 mode=indexing
                i -> [w1312]
                n617 = case shown="True" w1315 {
                  tunnel: [100.0 w1320] -> w1314
                  tunnel: [TRUE w1319] -> w1313
                  tunnel: w1312 -> [_ w1318]
                  frame False {
                  }
                  frame True {
                    n618 = local read "probe points per region"() -> (w1326:i32[])
                    n619 = local read "max scale array"() -> (w1325:i32[])
                    n620 = local read "min scale array"() -> (w1324:i32[])
                    n621 = local read "Thresholds:"() -> (w1328:T2)
                    n622 = Index Array(array=w1326) -> (element=w1322:i32)  [unwired: 1 in]
                    n623 = call "DisplayStriptestData.vi"("min scale array"=w1324, "max scale array"=w1325, "# probed"=w1322, "Display Stats?"=TRUE, "Thresholds"=w1328, "Region"=w1318) -> ("Strip Quality Data"=w1323:T16)  [unwired: 4 out]
                    n624 = Unbundle By Name(w1323) -> ("pass Rate in %"=w1320:dbl)
                    n625 = Greater?(x=w1320, y=98.0) -> (0:w1319:bool)
                  }
                }
              }
              n626 = And Array Elements(Boolean array=w1307) -> (logical AND=w1306:bool)
              n627 = Array Max & Min(array=w1309) -> (min value=w1308:dbl)  [unwired: 3 out]
            }
            frame True {
              n628 = for {
                N: w1339 -> [_]
                tunnel: w1338 -> [w1349] mode=indexing
                tunnel: w1337 -> [w1348] mode=indexing
                tunnel: [w1346] -> w1336 mode=indexing
                tunnel: [w1345] -> w1334 mode=indexing
                tunnel: [w1344] -> w1332
                shift-right: [w1343] -> w1329
                shift-left: _ -> [w1340]
                i -> [w1347]
                n629 = case shown="True" w1349 {
                  tunnel: w1347 -> [_ w1362]
                  tunnel: w1348 -> [_ w1361]
                  tunnel: [TRUE w1358] -> w1346
                  tunnel: [100.0 w1356] -> w1345
                  tunnel: [w1350 w1355] -> w1344
                  tunnel: [w1350 w1354] -> w1341
                  frame False {
                    w1350 = ""
                  }
                  frame True {
                    n630 = Unbundle By Name(w1361) -> ("Region"=w1360:string)
                    n631 = flat-sequence {
                      tunnel: w1362 -> [w1387]
                      tunnel: w1360 -> [w1371]
                      tunnel: [w1387] -> w1359
                      tunnel: [w1388] -> w1357
                      tunnel: [w1373] -> w1355
                      tunnel: [w1372] -> w1354
                      tunnel: [w1371] -> w1353
                      tunnel: w1359 -> [w1397]
                      tunnel: [w1399] -> w1358
                      tunnel: w1357 -> [w1395]
                      tunnel: [w1396] -> w1356
                      tunnel: w1353 -> [w1394]
                      frame #0 {
                        n632 = Concatenate Strings("Saving data for " ("string"), w1371) -> (w1391:string)
                        n633 = call "MultiRegionData.vi"("Action"=T7."Read Array", "Array No."=0, "Region index"=w1387) -> ("Array OUT"=w1379:dbl[])  [unwired: 3 in, 1 out]
                        n634 = call "MultiRegionData.vi"("Action"=T7."Read Array", "Array No."=1, "Region index"=w1387) -> ("Array OUT"=w1380:dbl[])  [unwired: 3 in, 1 out]
                        n635 = call "MultiRegionData.vi"("Action"=T7."Read Array", "Array No."=3, "Region index"=w1387) -> ("Array OUT"=w1364:dbl[])  [unwired: 3 in, 1 out]
                        n636 = call "MultiRegionData.vi"("Action"=T7."Read Array", "Array No."=4, "Region index"=w1387) -> ("Array OUT"=w1363:dbl[])  [unwired: 3 in, 1 out]
                        n637 = call "MultiRegionData.vi"("Action"=T7."Read Array", "Array No."=2, "Region index"=w1387) -> ()  [unwired: 3 in, 2 out]
                        n638 = local write "Status:"(w1391) -> ()
                        n639 = local read "Temperature Progression"() -> (w1376:T3)
                        n640 = Build Array(w1379, w1380, w1364, w1363) -> (w1378:dbl[][])
                        n641 = Transpose 2D Array(2D array=w1378) -> (transposed array=w1377:dbl[][])
                        n642 = Unbundle By Name(w1376) -> ("Humidity Array [RH %]"=w1375:dbl[], "Temperature Array [°C]"=w1374:dbl[])
                        n643 = call <vilib>:"Std Deviation and Variance.vi"("X"=w1375) -> ("mean"=w1367:dbl)  [unwired: 1 in, 2 out]
                        n644 = call <vilib>:"Std Deviation and Variance.vi"("X"=w1374) -> ("mean"=w1366:dbl)  [unwired: 1 in, 2 out]
                        n645 = call "SaveDataFile.vi"("Data Array"=w1377, "Temperature"=w1366, "Humidity"=w1367, "Array Titles"="ProbeplanIndex\tCurrent[nA]\tCapacitance[pF]\tResistance[MOhm]\n", "Strip Segment"=w1371) -> ("Filename OUT"=w1372:string, "Pathname OUT"=w1373:string, "Path + Filename OUT"=w1388:string)  [unwired: 7 in, 1 out]
                      }
                      frame #1 {
                        n646 = local read "probe points per region"() -> (w1404:i32[])
                        n647 = local read "max scale array"() -> (w1403:i32[])
                        n648 = local read "min scale array"() -> (w1402:i32[])
                        n649 = local read "Thresholds:"() -> (w1406:T2)
                        n650 = Index Array(array=w1404, index=w1397) -> (element=w1398:i32)
                        n651 = call "DisplayStriptestData.vi"("min scale array"=w1402, "max scale array"=w1403, "# probed"=w1398, "Display Stats?"=TRUE, "Thresholds"=w1406, "Region"=w1397) -> ("Strip Quality Data"=w1401:T16)  [unwired: 4 out]
                        n652 = Unbundle By Name(w1401) -> ("pass Rate in %"=w1396:dbl, "No of bad strips"=w1393:i32, "Bad channel list"=w1392:i32[], "Defect description list"=w1400:i32[])
                        n653 = call "CreateDefectFile.vi"("Segment:"=w1394, "Pass rate"=w1396, "Defect description list"=w1400, "Bad channel array"=w1392, "No of bad strips"=w1393, "Filename IN"=w1395) -> ("passed"=w1399:bool)  [unwired: 3 in, 2 out]
                      }
                    }
                  }
                }
                n654 = call <vilib>:"Space Constant.vi"() -> ("String"=w1342:string)
                n655 = Concatenate Strings(w1340, w1342, w1341) -> (w1343:string)
              }
              n656 = call <vilib>:"Space Constant.vi"() -> ("String"=w1331:string)
              n657 = And Array Elements(Boolean array=w1336) -> (logical AND=w1335:bool)
              "Module failed/passed" <- w1335
              n658 = Array Max & Min(array=w1334) -> (min value=w1333:dbl)  [unwired: 3 out]
              n659 = Concatenate Strings(w1332, w1331, w1329) -> (w1330:string)
            }
          }
          n660 = local read "Temperature Progression"() -> (w1151:T3)
          n661 = Unbundle By Name(w1151) -> ("Temperature Array [°C]"=w1149:dbl[], "Humidity Array [RH %]"=w1150:dbl[])
          n662 = call <vilib>:"Std Deviation and Variance.vi"("X"=w1149) -> ("standard deviation"=w1143:dbl)  [unwired: 1 in, 2 out]
          n663 = call <vilib>:"Std Deviation and Variance.vi"("X"=w1150) -> ("standard deviation"=w1142:dbl)  [unwired: 1 in, 2 out]
          n664 = Greater?(x=w1143, y=5) -> (0:w1140:bool)
          n665 = Greater?(x=w1142, y=10) -> (0:w1141:bool)
          n666 = Select(t="large humidity fluctuations", s=w1141, f="") -> (s? t:f=w1138:string)
          n667 = Select(t="large temperature fluctuations", s=w1140, f="") -> (s? t:f=w1137:string)
          n668 = Concatenate Strings(w1137, "\t", w1138) -> (w1136:string)
          n669 = call "WriteLogFile.vi"("Automatic warning"=w1136, "Data File"=w1153, "DUT passed?"=w1155, "Value TechSpec criteria"=w1154, "Files saved?"=w1152) -> ()  [unwired: 6 in, 1 out]
        }
      }
    }
  }
